vi "SetList.vi"() -> ()   [LabVIEW 2013]
uses:
  ColumnVIs/Column/Column.lvclass
  ColumnVIs/ModeCol/ModeCol.lvclass
  ColumnVIs/GroupCol/GroupCol.lvclass
  ColumnVIs/DigitalCol/DigitalCol.lvclass
  ColumnVIs/TriggerCol/TriggerCol.lvclass
  ColumnVIs/SingleValCol/SingleValCol.lvclass
  <vilib>/event_ctls.llb/eventvkey.ctl
  <vilib>/Utility/miscctls.llb/LVRowAndColumnTypeDef.ctl
  TypeDefs/RowType.ctl
  TypeDefs/TableHistory.ctl
  TypeDefs/TableArray.ctl
  DeviceVIs/Device/Device.lvclass
  TypeDefs/PreviousVersionSelect.ctl
  VariableManagerCodes/VariableManager/VariableManager.lvclass
  <vilib>/Utility/miscctls.llb/LVRowAndColumnUnsignedTypeDef.ctl
  Utils/InsertMenu/InsertFunctionMenu.lvclass
  Utils/ExternalFeedback/JSON/JSONVarSet.ctl
  PackedLibraries/LuaEvaluatorAPI.lvlibp/API/t_Caching_Expression_Evaluator_Methods_Table.ctl
  <vilib>/Utility/miscctls.llb/LVPointTypeDef.ctl
  SetListPrefs/SetListPrefs.lvclass
  <vilib>/Utility/error.llb/DialogType.ctl
  SetListPrefs/SetListPrefs.lvclass/SetListPrefs.ctl
  TypeDefs/SaveCluster.ctl
  <vilib>/Utility/miscctls.llb/LVStringsAndValuesArrayTypeDef_I32.ctl
  TypeDefs/ClickEvent.ctl
  <vilib>/Utility/miscctls.llb/LVPoint32TypeDef.ctl
  TypeDefs/SetListRefs.ctl
  Utils/LVGitInterface/GitCommitCluster/CommitCluster.ctl
  VariableManagerCodes/SequenceIndex/SequenceIndex.lvclass
  Globals/PrefsGlobal.vi
  <vilib>/Utility/cursorutil.llb/Set Cursor (Icon Pict).vi
  VariableManagerCodes/API/VariableManagerAPI.lvlib
  Globals/UserFunctions.vi
  PackedLibraries/LuaEvaluatorAPI.lvlibp
panel:
  in  "CheckSave":bool
  out "Loading Text":string="Loading..."
  in  "Launch Viewer":bool
  out "Cycle Time (s)":dbl
  in  "UpdateHWI Button":bool
  in  "StopExperiment":bool
  in  "Run Seq Button":bool
  in  "RandomSequence":bool
  in  "Run Button":bool
  in  "Cycle":bool
  out "Procedure Name":string="test_branch"
  in  "Tab Control":T1(tab)
  in  "Resume Button":bool
  in  "Program only changes":bool=TRUE
  out "SequenceHistory":string[][](table)
  in  "File Number":i32
  in  "Program during MOT loading":bool
  in  "Additional wait time (s)":dbl
  out "Igor Inform String":string
  in  "FitCol2Text Button":bool
  in  "SetList Table":string[][](table)=[["initialize", "", "Ramp", "1", "1", "0", "0", "0", "0", "0", "0", "0", "0", "0", "0", "0", "0", "0", "0", "0", "0", "0", "0", "0", "0", "0", "0", "0", "0", "100m"]]
  in  "Undo":bool
  in  "Redo":bool
  in  "Select Layout":i32(ring)=-1 items=["(On-the-fly)"=-2, "All"=-1]
  in  "ConfigLayoutsButton":bool
  in  "ManageDevicesButton":bool
  in  "User defined functions":string="-- --------------------------------------------------------------------------\n-- RbYb Beatnote Command \"frequency\" functions\n--      These functions allow us to run a sequence using absolute frequency \n--      detuning by calculating the proper command \"frequency\"\n--\n--      NOTE: Only use one TA or Re \"comm\" function, or it isn't clear which setpoint will be used\n--\n--      18.Aug.2010: Updated Master AOM offset (40 --> 42.342).\n-----------------------------------------------------------------------------\nfunction TASlowComm(Detuning,AOM)\n    return (-1*Detuning+1126.48-60.32-42.342-2*AOM)/8\n   --positive detuning is BLUE detuned, zero detuning sets TA slower beam to the 87-Rb F=2 to F'=3\nend\n\nfunction TAMOTComm(Detuning,AOM)\n    return (-1*Detuning+1126.48-60.32-42.342+AOM)/8\n   --positive detuning is BLUE detuned, zero detuning sets TA MOT beam to the 87-Rb F=2 to F'=3\nend\n\nfunction TAPComm(Detuning,AOM)\n    return (-1*Detuning+1126.48-60.32-42.342+AOM)/8\n   --positive detuning is BLUE detuned, zero detuning sets TA Probe beam to the 87-Rb F=2 to F'=3\nend\n\nfunction ReMOTComm(Detuning,AOM)\n    return (Detuning+6568.03-1126.48+60.32+42.342-2*AOM)/64\n    --positive detuning is BLUE detuned, zero detuning sets Repump MOT beam to the 87-Rb F=1 to F'=2\nend\n\nfunction ReSlowComm(Detuning,AOM)\n    return (Detuning+6568.03-1126.48+60.32+42.342+2*AOM)/64\n    --positive detuning is BLUE detuned, zero detuning sets Repump slower beam to the 87-Rb F=1 to F'=2\nend\n\n--RbLi Probe (transverse coolign launch)\nfunction PComm(Detuning)\n    return (-1*Detuning+986.16)/8\n    --positive detuning is BLUE detuned, zero detuning sets Repump slower beam to the 87-Rb F=1 to F'=2\nend\n\n-- Creates an exponential ramp from A to B in tEnd seconds\n-- useful for stopping a ramp at different times to measure T, N\nfunction ExpRampStep(t, a, b, tau, tEnd)\n   return (b - a*exp(tEnd / tau) + (a-b)*exp(t/tau))/ ( 1 - exp(tEnd / tau) );\nend\n\nfunction ExpRampEnd(tEv, a, b, tau, tEnd)\n   return (b - a*exp(tEnd / tau) + (a-b)*exp(tEv/tau))/ ( 1 - exp(tEnd / tau) );\nend\n\nfunction ExpRamp2(t,a,tau)\n   return a*exp(-t/tau)\nend\n\nfunction ExpRamp2End(tEnd,a,tau)\n   return a*exp(-tEnd/tau)\nend\n\n-- Added log chip amplifier (1 V per decade) so now we provide linear ramp to get exponential\n--     note: log() is base 'e', log10 base '10'\nfunction LineEvap(t,a,tau)\n   return 1.027*(log10(a)-t/(2.30*tau))+0.0343\nend\n\n-- final value log(V) for LineEvap\nfunction LineEvapEnd(tEnd,a,tau)\n   return 1.027*(log10(a)-tEnd/(2.30*tau))+0.0343\nend\n\n-- Convert real dipole power to log chip request V\nfunction PtoV(pow)\n   return 1.010*log10(pow/0.770)\nend\n\n-- Convert 532 horizontal (main) beam power (in mW) to V-req\nfunction PtoV532m(pow)\n   return 1.01378*log10(pow/0.54672)\nend\n\n-- Convert 532 vertical (crossing) beam power (in mW) to V-req\nfunction PtoV532c(pow)\n   return 1.03459*log10(pow/0.619665)\nend\n\n-- Convert 1064 horizontal (main) beam power (in mW) to V-req\nfunction PtoV1064m(pow)\n   return 1.0035*log10(pow/1.2104)\nend\n----------------------------------------\n-- The following functions are part of the \"standard load\" of functions and should not be messed with\n-- They are here for reference only.\n-- Please add any user functions above this comment\n-- -------------------------------------------------------------------------------------------\n\n-- Creates a linear ramp from A to B\nfunction LineRamp(f, Initial, Final)\n    return (1-f)*Initial + f*Final;\nend\n\n-- Creates an exponential ramp from A to B\nfunction ExpRamp(t, a, b, tau)\n   return (b - a*exp(tMax / tau) + (a-b)*exp(t/tau))/ ( 1 - exp(tMax / tau) );\nend\n\n-- Creates a sinewave\nfunction SinRamp(t,Offset,A,Freq, Phase)\n    return Offset + A * sin(2*pi*Freq*t + Phase)\nend\n\n-- Creates a blackman pulse\nfunction Blackman(f, Offset, A)\n    return Offset +  A*sqrt(0.5*cos(3.1415*(2*f-1))+0.08*cos(2*pi*(2*f-1))+0.42);\nend\n\n-- Creates a half-gauss ramp\nfunction HalfGaussRamp(t, a, b, Width)\n    local y;\n    y = exp(-(tMax^2)/Width^2);\n    y = (a -  b*y)/(1-y)  +  ((b-a)/(1-y))*exp(-((t-tMax)^2)/Width^2);\n    return y;\nend\n\n-- Creates an \"O'Hara\" ramp from A to B, for dipole evaporation\nfunction EvapRamp(t, a, b, tau)\n   local y;\n  y = log(a/b) / log(1+tMax/tau);\n  y = a * (1+t/tau)^(-y);\n  return y;\nend\n"
  in  "Save to File":bool
  in  "ImportToRepo":bool
  in  "Author":u16(ring) items=["SetList Program <JQIbot@users.noreply.github.com>"]
  out "Loaded Description":string
  out "LoadHash":string caption="Loaded Hash"
  in  "Load from File":bool
  in  "Description (Repo Only)":string
  in  "SaveTitle":string caption="Title/Filename"
  in  "Load keep cur. format":bool
  in  "Version Selection":T2=enum."Load DDS 4.10"
  in  "Old HWGlobals Path":path=path "C:/Experiment/Data Acquisition/Hardware Control/Hardware/2014/6Jun2014_PowerCal" caption="This file has not been loaded or saved"
  in  "Old HWGlobals History":string(combo)
  in  "Old Procedure Path":path=path "C:/Experiment/Data Acquisition/Hardware Control/procedures/Benchmarks/12Feb2014_RbQuad" caption="This file has not been loaded or saved"
  in  "Old Procedure History":string(combo)
  in  "Load Old":bool
  in  "Load Recent":string(combo)
  in  "Save to Repo":bool
  in  "Load from Repo":bool
  out "Loaded Version":string="testing"
  out "SaveHash":string caption="Saved Hash"
  in  "Error Log":i32(listbox)
  out "Table error":errorcluster
  out "Run/Sequence Error":errorcluster
  out "Update Error":errorcluster
  out "Load Long Hash/Filename":string
  out "LoadRecentFile":string
  out "TCP Quit Signal":bool
  in  "FunctionMenu":refnum<class "InsertFunctionMenu.lvclass">
  out "Index Values":T3
  out "#chg":i16
  out "Defer Pnl Upd":bool=TRUE
  out "diag. loop cnt":i32
  out "Key Focus":bool
  out "Edit Position":T4={"Row"=-2, "Column"=-2}
  out "withinSelection?":bool
  out "Val Change":bool=TRUE
  out "Selection Size":T4
  out "Selection Start":T4={"Row"=25, "Column"=30}
  out "Char":i16
  out "VKey":T5
  out "withinData?":bool=TRUE
  out "data cols":i32=134
  out "data rows":i32=26
  out "Number of Rows":u32=36
  out "Number of Columns":u32=62
  in  "Devices":refnum<class "Device.lvclass">[](array[class])
  out "Devices queue":refnum<queue>
  out "DevNums":i32[](array[numeric])=[0, 0, 0, 0, 0, 0, 0, 0, 0, 0, 0, 0, 0, 0, 0, 0, 0, 0, 0, 0, 0, 0, 0, 0, 0, 0, 0, 0, 0, 0, 1, 1, 1, 1, 1, 1, 1, 1, 1, 1, 1, 1, 1, 1, 1, 1, 1, 1, 1, 1, 2, 2, 2, 2, 2, 2, 2, 2, 2, 2, 2, 2, 2, 2, 2, 2, 2, 2, 2, 2, 3, 3, 3, 3, 3, 3, 3, 3, 3, 3, 3, 3, 3, 3, 3, 3, 3, 3, 3, 3, 4, 4, 4, 4, 4, 4, 4, 4, 5, 5, 5, 5, 5, 5, 5, 5, 5, 5, 5, 5, 6, 6, 6, 6, 6, 6, 6, 6, 6, 6, 6, 6, 7, 7, 7, 7, 7, 7, 7, 7, 7, 7, 7, 7]
  out "Col array":refnum<class "Column.lvclass">[](array[class])
  out "Seq. Event":refnum<user-event>
  out "Update Event":refnum<user-event>
  out "Update Notifier":refnum<notifier>
  out "Dyn. Regist. Update Event":refnum<event-registration>
  out "Dyn.\nRegist.\nSeq.\nEvent":refnum<event-registration>
  out "Dyn.\nRegist.\nCycleX\nEvent":refnum<event-registration>
  out "CycleX Event":refnum<user-event>
  in  "row type":T6=enum."within data"
  out "Button\n(Mouse Down?)":u16
  in  "VariableManager":refnum<class "VariableManager.lvclass">=refnum
  out "Igor Inform Array":string[](array[string])
  out "Clipboard":string[][](array[string])
  out "Table History":T7
  in  "Diag. loop?":bool
  in  "PreserveHist?":bool
  out "Hist. size":i32=2
  in  "Defer Updates?":bool=TRUE
  in  "initialize?":bool
  in  "Debug: apply appearance":bool
  out "Viewer ref":refnum<vi>
  out "LoadRecentHash":string
  out "FBVarSeqSetJSON queue":refnum<queue>
  in  "SetSharedVarIP":bool
  in  "Shared Variable Deploy IP":string
  in  "Git Authors":string[][](table)
  in  "ManGitCmd":bool
  in  "AutoGitCmd":bool
  out "Git Command":string
  in  "Procedure Repository":path
  in  "DetachVMUIonStart":bool
  in  "Auto PressHWUpdate":bool
  in  "Hide Checked Devices":i32(listbox)=3
  in  "Reset to Saved Window Position":bool
  in  "Save Current Window Position":bool
  in  "Reset at Startup":bool
  in  "quit":bool
  # "What do we actually need from old CycleX here?\n   - Inform Igor?\n   - Program changes/ during MOT load?"
  # "(not presently implemented)"
  # "To End Table Editing:\n  - Press <Ctrl>-<Return>\n  - Press <Keypad Enter>\n  - Click outside the table"
  # "Variable Manager will be initialized when the VI is run.\n\nIf it is currently running and you can see this message, then you've \"popped out\" the Variable manager.\nClose it with the \"red-x\" to replace it here."
  # "Note: For each index <idx>, the names <idx>_f and <idx>_max\nare also defined as the fractional sequence step and max steps."
  # "NOTE: these persist until LabVIEW is closed or you overwrite them."
  # "In the context of ramps several variables are passed or specified that may be used here:\n\n   - f the fractional position of a point in a ramp\n   - t the current time in a ramp\n   - dt the current timestep size.\n   - tMax the total duration of the ramp\n\ntemporary \"storage\":\n-- not functionality for strings (always treated as double)\nfunction bnot(a)\n   -- this \"(bool exp.) and b or c\" is equivalent to \"(bool exp.) ? b : c\" syntax.\n   -- caution: undefined variables evaluate to \"false\" so will NOT throw an error as argument\n   return a==0 and 1 or 0\nend"
  # "Present Version"
  # "Save/Load from present version (select single file):\nWe need to save the following:\n   - Devices (with the columns and data pushed from table first!)\n   - Layout ring (for layout names, #s)\n   - variables\n   - user functions\n   - ... ?"
  # "Load... and Save... bring up dialog box.\nLoad Recent will load the selected procedure.\nBUG: not a value change if select what's on top!"
  # "Load from older versions (select Procedure and Hardware globals)\n(1) reformat old file to give device array\n(2) collect variables and send them to variable manager\n(3) load user functions\n(4) construct layouts, if any (at least a default \"all on\" layout)\n(5) ...?"
  # "Previous Versions"
  # "Most of these controls/indicators MUST exist. At the bottom and right are some diagnostics."
  # "\"Diagnostics\" we can't delete:\nRow Type, ..."
  # "(must abort to stop,\nstill better to QUIT first)"
  # "diagnostics:"
  # "presently not set\nfor row header"
  # "The table size in (rows, cols) is NOT same as\nthe size of the data array displayed in table."
  # "SetList was developed for the JQI neutral atom cooling/trapping groups. \nPrimary contributions authored by Zack Seigel, Creston Herold, Joe Tiamsuphat, Bob Wyllie, Zach Smith.\n\nFAQs\n------\n * How are digital variables interpreted?\n     Any value not equal to 0 is high, only 0 is low.\n\n * What does Ramp mean?\n     Slave devices will be triggered (if necessary) during a Ramp line with a period given by \"Step.\" The output\n     is determined with Lua \"User Functions\" and the reserved f,t variables described on that tab.\n     Master (PulseBlaster) channels will output a *static* output during ramps. That means functions of f or t\n     will only be evaluated at their *first* point for Master channels.\n\n * How do you use Loop - EndLoop?\n     The \"Step\" column on a Loop line is for # loops and is ignored on an EndLoop line. Nesting is supported\n     up to 7 levels deep, but only Master (PulseBlaster) outputs can change. Therefore Ramps are not allowed \n     within loops.\n\n * How does Halt work?\n     On a Halt line, the Master (PulseBlaster) will change to the selected outputs and then wait for a trigger.\n     Upon receiving a trigger (hardware or software), it will wait for the specified Delay and then go to the \n     next instruction.\n\n * Where can I learn more?\n     Complete documentation of this code, including adding your own custom device can be found on the\n     JQI wiki (https://jqi-wiki.physics.umd.edu, login required)."
  # "Git Save System Settings"
  # "To setup git:\n     1) Click 'Auto-Detect Command' to find the git installation on your computer\n     2) Point 'Procedure Repository' to the path to store save files by typing or browsing.\n     (Optional) Add authors"
  # "Leave email blank to use \"JQIbot@users.noreply.github.com\""
  # "Won't show checked items in the \"Add Device...\" dropdown of the \"Manage Devices\" window"
  # "Window Position"
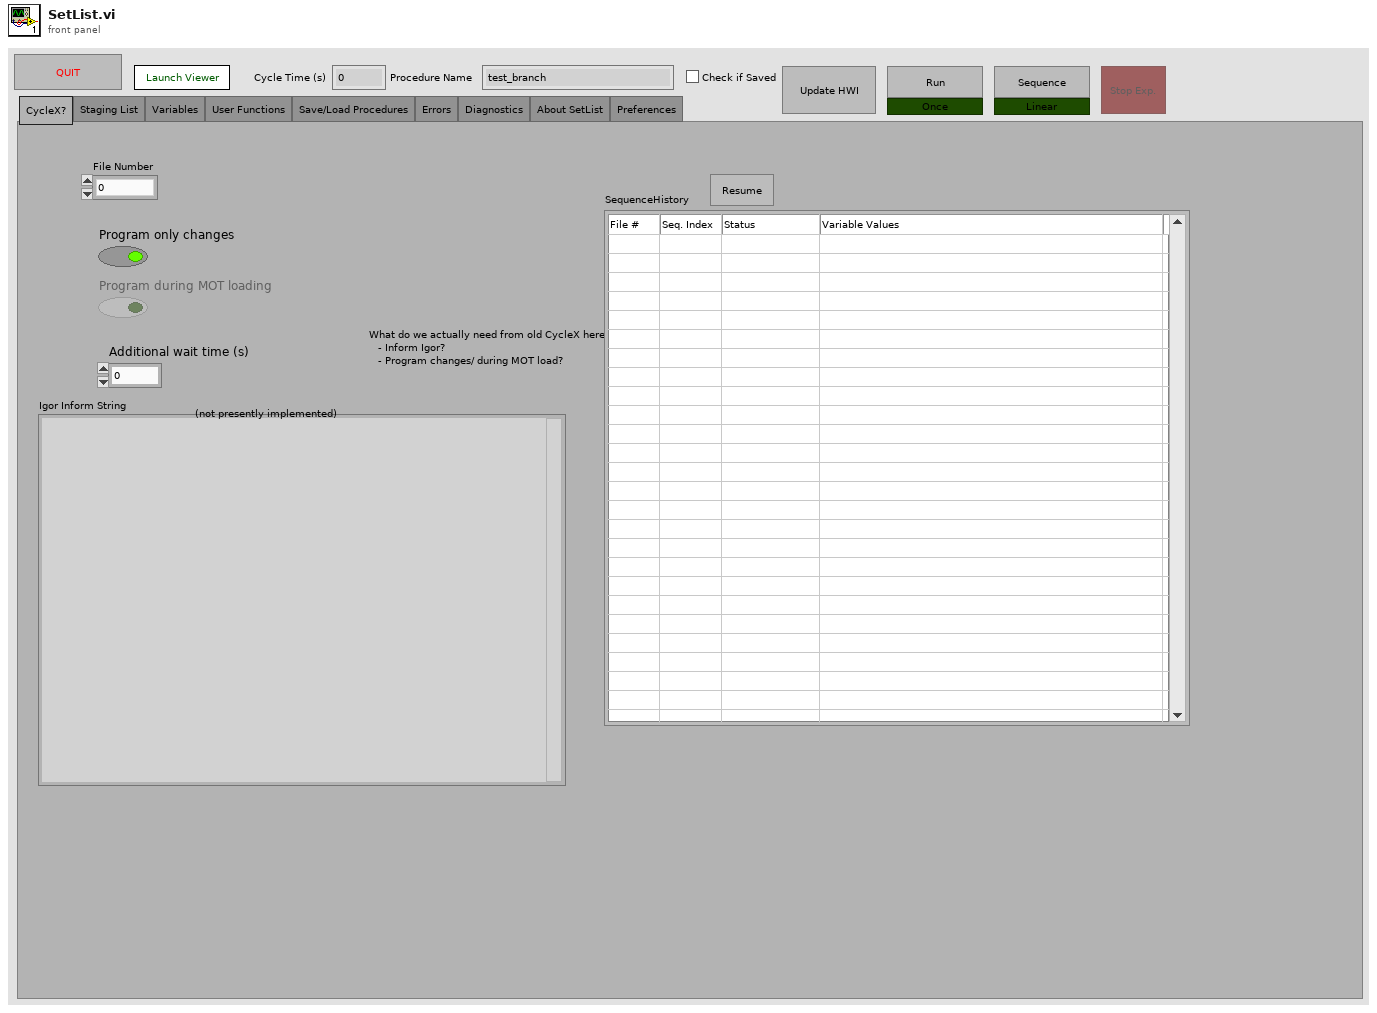
[diagram p1: front panel]
types:
  T1 = enum32{"CycleX?", "Staging List", "Variables", "User Functions", "Save/Load Procedures", "Errors", "Diagnostics", "About SetList", "Preferences"}
  T2 = typedef "PreviousVersionSelect.ctl" = enum32{"Load PreDDS 4.10", "Load early 2009 files", "Load 2009-2010 files", "Load DDS 4.10", "Load v4.09"}
  T3 = typedef "LVRowAndColumnUnsignedTypeDef.ctl" = cluster{"Row":u32, "Column":u32}
  T4 = typedef "LVRowAndColumnTypeDef.ctl" = cluster{"Row":i32, "Column":i32}
  T5 = typedef "eventvkey.ctl" = enum16{"ASCII", "Enter", "Return", "Shift", "Ctrl", "Alt", "Cmd", "Opt", "Caps", "NumLock", "Clear", "Break", "Up", "Down", "Left", "Right", "Insert", "Delete", "Home", "End", "PageUp", "PageDown", "Escape", "Help", "Pause", "ScrollLock", "F1", "F2", "F3", "F4", "F5", "F6", "F7", "F8", "F9", "F10", "F11", "F12", "F13", "F14", "F15", "F16", "F17", "F18", "F19", "F20", "F21", "F22", "F23", "F24", "Play", "VolumeUp", "VolumeDown", "Mute", "Two Byte Char"}
  T6 = typedef "RowType.ctl" = enum16{"below data", "within data", "column header", "first row"}
  T7 = typedef "TableHistory.ctl" = cluster{"Undo pointer":i32, "OldTable Array":T8}
  T8 = typedef "TableArray.ctl" = string[]
  T9 = typedef "JSONVarSet.ctl" = string[]
  T10 = typedef "LVPointTypeDef.ctl" = cluster{"Horizontal":i16, "Vertical":i16}
  T11 = typedef "LuaEvaluatorAPI.lvlibp/t_Caching_Expression_Evaluator_Methods_Table.ctl" = enum16{"set", "get", "eval", "assign", "isvalid", "execute", "evaltable", "close"}
  T12 = enum8{"Enabled", "Disabled", "Disabled and Grayed Out"}
  T13 = typedef "LVRectTypeDef.ctl" = cluster{"Left":i16, "Top":i16, "Right":i16, "Bottom":i16}
  T14 = cluster{"WindowBounds":T13, "ResetPositionAtStartup":bool}
  T15 = cluster{"Device Class Name":string, "Class Path":path}[]
  T16 = typedef "ClickEvent.ctl" = cluster{"CtlRef":refnum<vi>, "Coords":T17, "Button":u16, "Mods":cluster{"Double Click":bool, "Menu Key":bool}, "PlatMods":cluster{"Shift":bool, "Ctrl":bool, "Alt":bool, "Cmd":bool, "Opt":bool}}
  T17 = typedef "LVPoint32TypeDef.ctl" = cluster{"Horizontal":i32, "Vertical":i32}
  T18 = typedef "SetListRefs.ctl" = cluster{"Clipboard":refnum<vi>, "Layout Ring Refnum":refnum<vi>, "Col Array Ref in":refnum<vi>, "VariableManagerRef":refnum<vi>, "Table CtlRef In":refnum<vi>, "Table History ref":refnum<vi>, "Devices queue":refnum<queue>, "FunctionMenu Ref":refnum<vi>}
  T19 = typedef "SaveCluster.ctl" = cluster{"Version":string, "Devices":refnum<class "Device.lvclass">[], "Select Layout":i32, "Layout:Strings And Values []":T20, "User defined functions":string, "VariableManager":refnum<class "VariableManager.lvclass">}
  T20 = typedef "LVStringsAndValuesArrayTypeDef_I32.ctl" = cluster{"String":string, "Value":i32}[]
  T21 = cluster{"Title":string, "Description":string, "Author":string}
  T22 = typedef "CommitCluster.ctl" = cluster{"Hash":string, "Date":string, "Name":string}
  T23 = enum32{"CycleX?", "Staging List", "Variables", "User Functions", "Save/Load Procedures", "Errors", "Diagnostics", "About SetList"}
  T24 = cluster{"Shift":bool, "Ctrl":bool, "Alt":bool, "Cmd":bool, "Opt":bool}
  T25 = typedef "ClickReturn.ctl" = cluster{"Button":u16, "Mods":cluster{"Double Click":bool, "Menu Key":bool}, "PlatMods":cluster{"Shift":bool, "Ctrl":bool, "Alt":bool, "Cmd":bool, "Opt":bool}, "Discard?":bool}
  T26 = typedef "DialogType.ctl" = u16
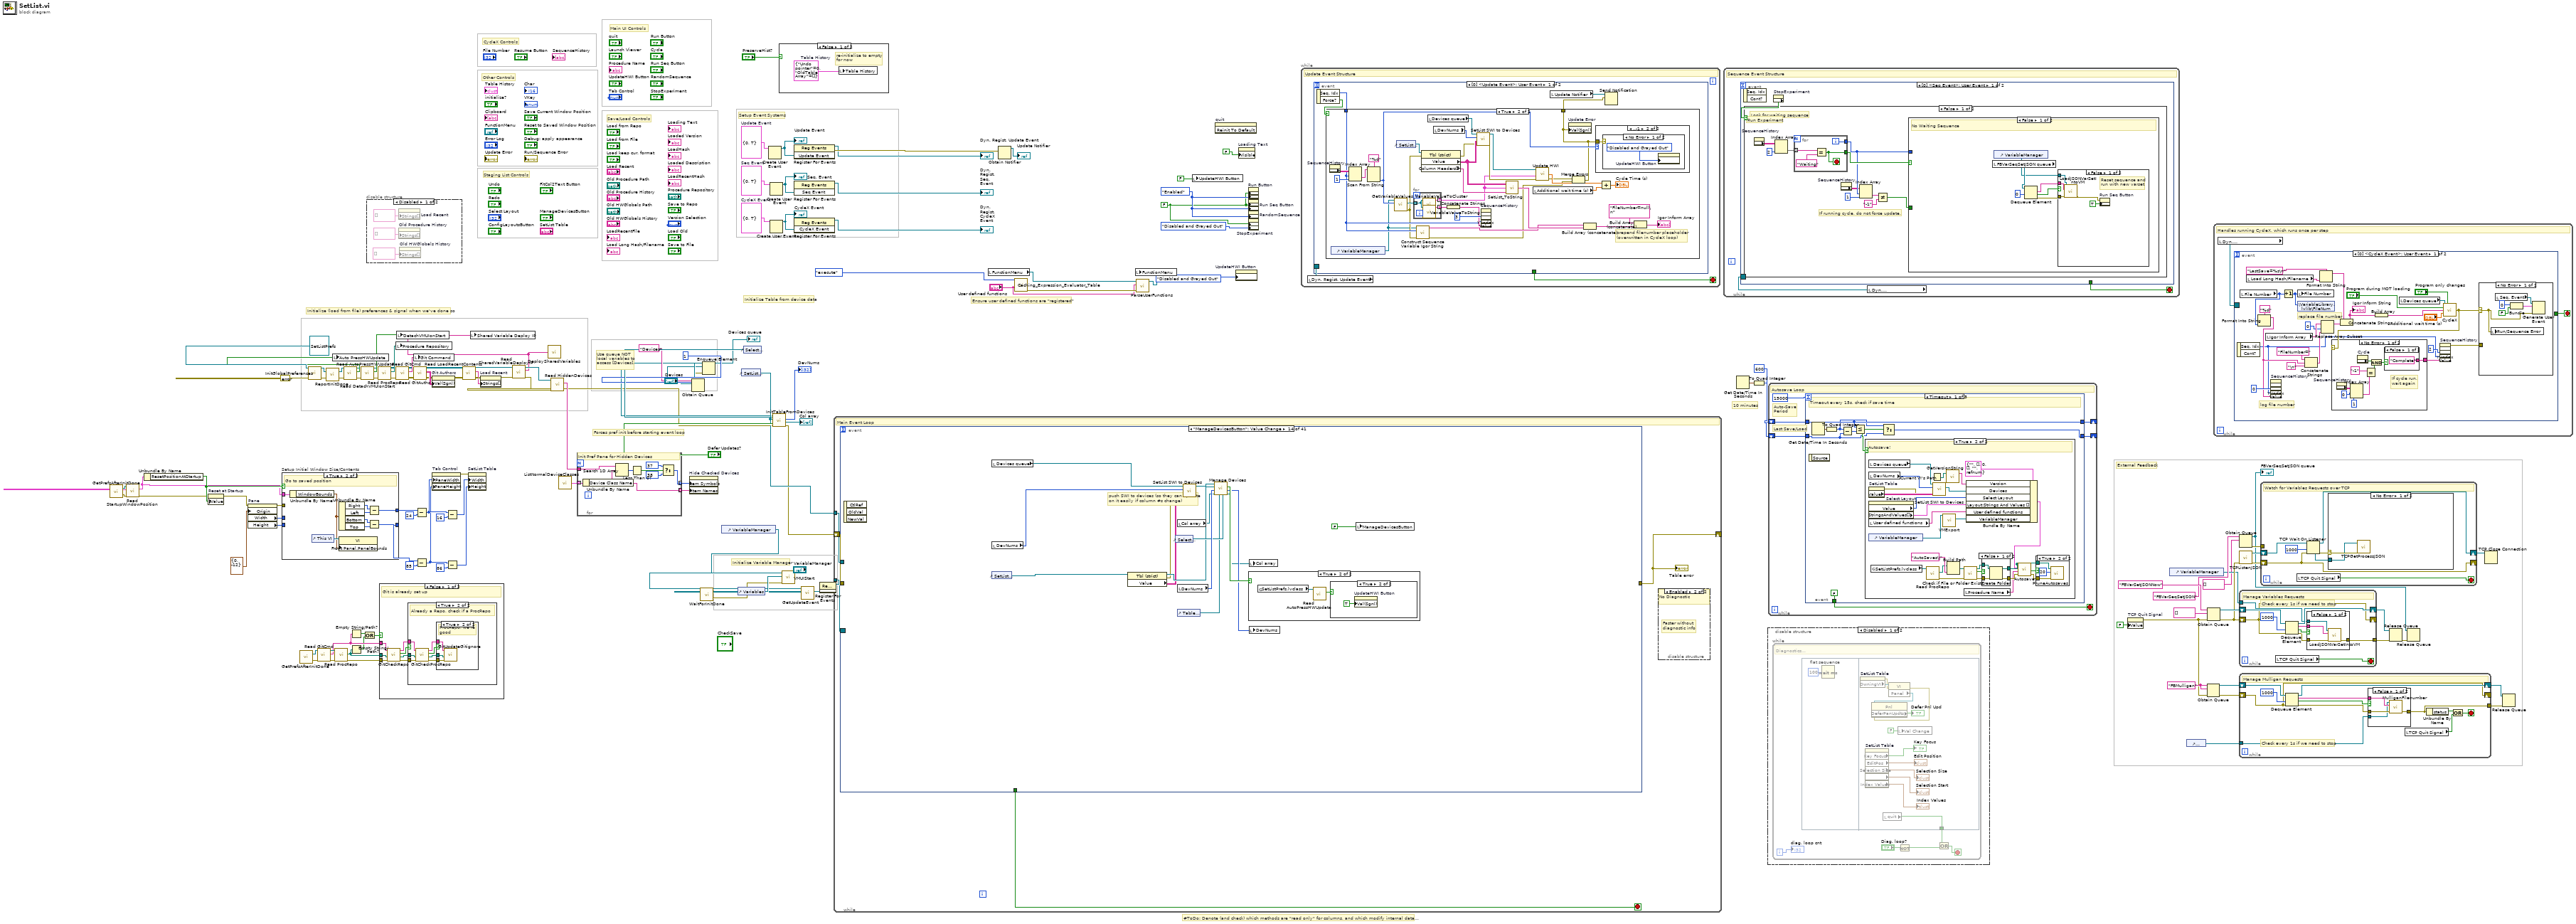
[diagram p0: block diagram]
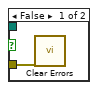
[diagram p8: hidden frame]
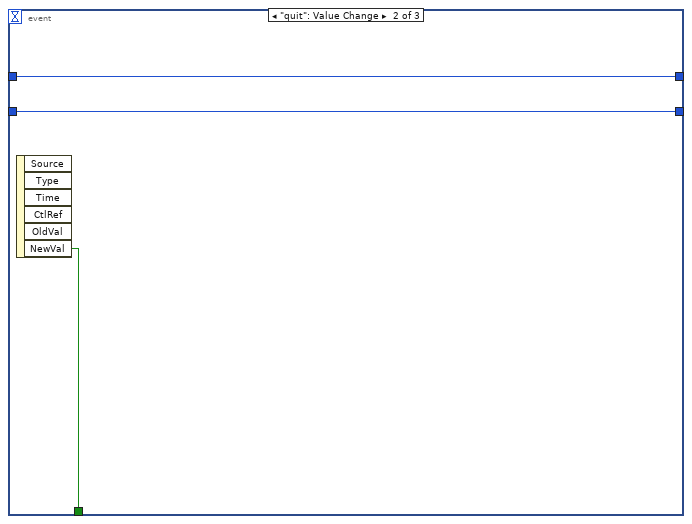
[diagram p9: hidden frame]
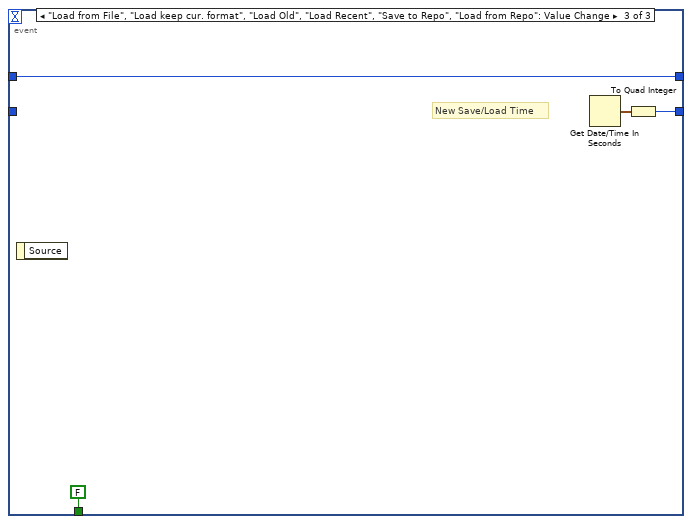
[diagram p10: hidden frame]
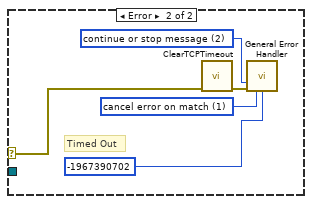
[diagram p11: hidden frame]
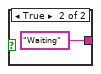
[diagram p15: hidden frame]
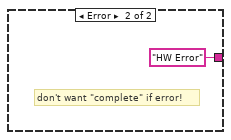
[diagram p16: hidden frame]
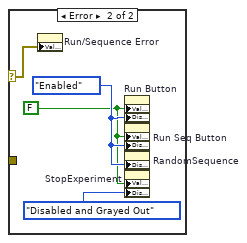
[diagram p17: hidden frame]
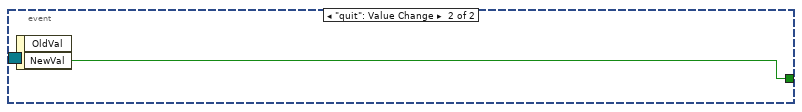
[diagram p18: hidden frame]
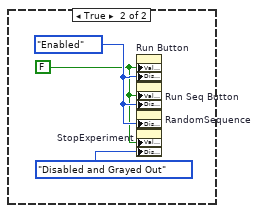
[diagram p20: hidden frame]
diagram:
  w56 = "FBMulligan" ("name (unnamed)")
  w110 = T12."Enabled" ("Disabled")
  w109 = FALSE
  w120 = cluster{"Seq. Idx":i32, "Cont?":bool} {"Seq. Idx"=0, "Cont?"=TRUE}  # CycleX Event
  w129 = cluster{"Seq. Idx":i32, "Cont?":bool} {"Seq. Idx"=0, "Cont?"=TRUE}  # Seq Event
  w130 = cluster{"Seq. Idx":i32, "Force?":bool} {"Seq. Idx"=0, "Force?"=TRUE}  # Update Event
  # "External Feedback"
  # "10 minutes"
  # "Forces pref init before starting event loop"
  # "Initialize (load from file) preferences & signal when we've done so"
  # "CycleX Controls"
  # "Main UI Controls"
  # "Other Controls"
  # "Save/Load Controls"
  # "Staging List Controls"
  # "Setup Event Systems"
  # "Use queue NOT\nlocal variables to\naccess [Devices]."
  # "Ensure user defined functions are \"registered\""
  # "Initialize Variable Manager"
  # "Initialize Table from device data"
  # "#ToDo: Denote (and check) which methods are \"read only\" for columns, and which modify internal data..."
  n1 = call "GetPrefsAfterInitDone.vi"() -> ("error out"=w82:errorcluster, "Preferences out"=w81:refnum<class "SetListPrefs.lvclass">)  [unwired: 2 in]
  n2 = call "Read StartupWindowPosition.vi"("error in (no error)"=w82, "SetListPrefs in"=w81) -> ("error out"=w79:errorcluster, "StartupWindowPosition"=w78:T14)  [unwired: 7 in, 1 out]
  n3 = Unbundle By Name(w78) -> ("ResetPositionAtStartup"=w80:bool)
  n4 = property on="Reset at Startup" class="Bool (strict)"(error in=w79, "Value"=w80) -> (error out=w77:errorcluster)  [unwired: 1 in, 1 out]
  n5 = property on="Pane" class="Pane"(error in=w77, "Origin"=T10 {"Horizontal"=0, "Vertical"=-12}) -> (error out=w76:errorcluster, "Width"=w75:u32, "Height"=w74:u32)  [unwired: 1 in, 1 out]
  n6 = case "Setup Initial Window Size/Contents" shown="True" w80 {
    tunnel: w78 -> [_ w142]
    tunnel: w76 -> [_ _]
    tunnel: w75 -> [w133 _]
    tunnel: w74 -> [w134 _]
    tunnel: [w133 w136] -> w73
    tunnel: [w134 w135] -> w72
    frame False {
      # "Keep current, but still resize contents"
    }
    frame True {
      # "Go to saved position"
      n7 = Unbundle By Name(w142) -> ("WindowBounds"=w137:T13)
      n8 = control-ref of="This VI"() -> (w143:refnum<vi>)
      n9 = Unbundle By Name(w137) -> ("Right"=w141:i16, "Left"=w140:i16, "Bottom"=w139:i16, "Top"=w138:i16)
      n10 = property class="VI"(reference=w143, "Front Panel.PanelBounds"=w137) -> ()  [unwired: 1 in, 2 out]
      n11 = Subtract(x=w141, y=w140) -> (x-y=w136:i16)
      n12 = Subtract(x=w139, y=w138) -> (x-y=w135:i16)
    }
  }
  n13 = call "GetPrefsAfterInitDone.vi"() -> ("error out"=w20:errorcluster, "Preferences out"=w19:refnum<class "SetListPrefs.lvclass">)  [unwired: 2 in]
  n14 = call-dynamic "InitGlobalPreferences.vi"("error in (no error)"=errorcluster {"status"=FALSE, "code"=0, "source"=""} ("error out"), "Preferences in"=refnum<class "SetListPrefs.lvclass"> refnum ("SetListPrefs.lvclass")) -> ("error out"=w84:errorcluster, "Preferences out"=w83:refnum<class "SetListPrefs.lvclass">)  [unwired: 7 in, 1 out]
  n15 = call "Read GitCmd.vi"("error in (no error)"=w20, "SetListPrefs in"=w19) -> ("error out"=w18:errorcluster, "GitCmd"=w15:string, "SetListPrefs out"=w16:refnum<class "SetListPrefs.lvclass">)  [unwired: 7 in]
  n16 = call "ReportInitDone.vi"("error in (no error)"=w84, "Preferences in"=w83) -> ("error out"=w67:errorcluster, "Preferences out"=w68:refnum<class "SetListPrefs.lvclass">)
  n17 = call "Read ProcRepo.vi"("error in (no error)"=w18, "SetListPrefs in"=w16) -> ("error out"=w17:errorcluster, "ProcRepo"=w14:path)  [unwired: 7 in, 1 out]
  n18 = call "Read AutoPressHWUpdate.vi"("error in (no error)"=w67, "SetListPrefs in"=w68) -> ("error out"=w64:errorcluster, "AutoPressHWUpdate"=w66:bool, "SetListPrefs out"=w63:refnum<class "SetListPrefs.lvclass">)  [unwired: 7 in]
  n19 = local write "Auto PressHWUpdate"(w66) -> ()
  n20 = Empty String/Path?(string/path=w15) -> (empty?=w13:bool)
  n21 = Empty String/Path?(string/path=w14) -> (empty?=w12:bool)
  n22 = call "Read DetachVMUIonStart.vi"("error in (no error)"=w64, "SetListPrefs in"=w63) -> ("error out"=w42:errorcluster, "DetachVMUIonStart"=w62:bool, "SetListPrefs out"=w40:refnum<class "SetListPrefs.lvclass">)  [unwired: 7 in]
  n23 = Or(x=w13, y=w12) -> (x .or. y?=w11:bool)
  n24 = disable-structure shown="Disabled" {
    frame Disabled {
      n25 = property on="Load Recent" class="CmbBox"("Strings[]"=string[] [] ("Strings []")) -> ()  [unwired: 2 in, 2 out]
      n26 = property on="Old Procedure History" class="CmbBox"("Strings[]"=string[] [] ("Strings []")) -> ()  [unwired: 2 in, 2 out]
      n27 = property on="Old HWGlobals History" class="CmbBox"("Strings[]"=string[] [] ("Strings []")) -> ()  [unwired: 2 in, 2 out]
    }
    frame Enabled {
    }
  }
  n28 = call "Read ProcRepo.vi"("error in (no error)"=w42, "SetListPrefs in"=w40) -> ("error out"=w39:errorcluster, "ProcRepo"=w41:path, "SetListPrefs out"=w38:refnum<class "SetListPrefs.lvclass">)  [unwired: 7 in]
  n29 = case shown="False" w11 {
    tunnel: w15 -> [w153 _]
    tunnel: w17 -> [w148 _]
    tunnel: w14 -> [w147 _]
    frame False {
      # "Git is already set up"
      n30 = call "GitCheckRepo.vi"("error in (no error)"=w148, "Directory"=w147, "Git exec"=w153) -> ("error out"=w150:errorcluster, "Directory out"=w151:path, "ProcedureRepo?"=w149:bool, "Git exec out"=w152:string)  [unwired: 5 in]
      n31 = case shown="True" w149 {
        tunnel: w150 -> [_ w160]
        tunnel: w151 -> [_ w159]
        tunnel: w152 -> [_ w158]
        frame False {
          # "Do Nothing"
        }
        frame True {
          # "Already a Repo, check if a ProcRepo"
          n32 = call "GitCheckProcRepo.vi"("error in (no error)"=w160, "Directory"=w159, "Git exec"=w158) -> ("error out"=w156:errorcluster, "Directory out"=w155:path, "ProcedureRepo?"=w154:bool, "Git exec out"=w157:string)  [unwired: 5 in]
          n33 = case shown="True" w154 {
            tunnel: w157 -> [_ w161]
            tunnel: w156 -> [_ w163]
            tunnel: w155 -> [_ w162]
            frame False {
              # "Do Nothing"
            }
            frame True {
              # "ProcRepo, we're good"
              n34 = call "GitUpdateGitignore.vi"("error in (no error)"=w163, "Directory in"=w162, "Git exec in"=w161) -> ()  [unwired: 6 in, 3 out]
            }
          }
        }
      }
    }
    frame True {
      # "Git isn't fully set up yet."
    }
  }
  n35 = local write "Procedure Repository"(w41) -> ()
  n36 = call "Read GitCmd.vi"("error in (no error)"=w39, "SetListPrefs in"=w38) -> ("error out"=w36:errorcluster, "GitCmd"=w37:string, "SetListPrefs out"=w35:refnum<class "SetListPrefs.lvclass">)  [unwired: 7 in]
  n37 = local write "DetachVMUIonStart"(w62) -> ()
  n38 = local write "Git Command"(w37) -> ()
  n39 = call "Read GitAuths.vi"("error in (no error)"=w36, "SetListPrefs in"=w35) -> ("error out"=w33:errorcluster, "GitAuths"=w34:string[][], "SetListPrefs out"=w32:refnum<class "SetListPrefs.lvclass">)  [unwired: 7 in]
  n40 = Subtract(x=w73, y=u32 24) -> (x-y=w89:u32)
  n41 = Subtract(x=w72, y=u32 85) -> (x-y=w88:u32)
  n42 = property on="Git Authors" class="Tbl (strict)"(error in=w33, "Val(Sgnl)"=w34) -> (error out=w31:errorcluster)  [unwired: 1 in, 1 out]
  n43 = property on="Tab Control" class="TabCtl (strict)"("PaneWidth"=w89, "PaneHeight"=w88) -> (error out=w90:errorcluster)  [unwired: 2 in, 1 out]
  n44 = Subtract(x=w89, y=u32 16) -> (x-y=w92:u32)
  n45 = Subtract(x=w88, y=u32 86) -> (x-y=w91:u32)
  n46 = call "Read LoadRecentContents.vi"("error in (no error)"=w31, "SetListPrefs in"=w32) -> ("error out"=w30:errorcluster, "LoadRecentContents"=w29:string[], "SetListPrefs out"=w6:refnum<class "SetListPrefs.lvclass">)  [unwired: 7 in]
  n47 = property on="SetList Table" class="Tbl (strict)"(error in=w90, "Width"=w92, "Height"=w91) -> ()  [unwired: 1 in, 2 out]
  n48 = property on="Load Recent" class="CmbBox"(error in=w30, "Strings[]"=w29) -> (error out=w8:errorcluster)  [unwired: 1 in, 1 out]
  n49 = call "Read SharedVariableDeployIP.vi"("error in (no error)"=w8, "SetListPrefs in"=w6) -> ("error out"=w7:errorcluster, "SharedVariableDeployIP"=w4:string, "SetListPrefs out"=w5:refnum<class "SetListPrefs.lvclass">)  [unwired: 7 in]
  n50 = local write "Shared Variable Deploy IP"(w4) -> ()
  n51 = call "DeploySharedVariables.vi"("Target IPAddress"=w4) -> ()  [unwired: 1 out]
  n52 = call "Read HiddenDevices.vi"("error in (no error)"=w7, "SetListPrefs in"=w5) -> ("error out"=w10:errorcluster, "HiddenDevices"=w69:string[])  [unwired: 7 in, 1 out]
  n53 = call "ListNormalDeviceClasses.vi"() -> ("Detected Device Classes"=w9:T15)  [unwired: 1 in]
  n54 = for {
    tunnel: [w164] -> w71 mode=indexing
    tunnel: [w169] -> w70 mode=indexing
    tunnel: w69 -> [w168]
    tunnel: w9 -> [w165] mode=indexing
    # "Init Pref Pane for Hidden Devices"
    n55 = Unbundle By Name(w165) -> ("Device Class Name"=w164:string)
    n56 = Search 1D Array(1D array=w168, element=w164) -> (index of element=w167:i32)  [unwired: 1 in]
    n57 = Less Than 0?(x=w167) -> (x < 0?=w166:bool)
    n58 = Select(t=37, s=w166, f=38) -> (s? t:f=w169:i32)
  }
  n59 = property on="Hide Checked Devices" class="LstBox (strict)"("Item Symbols"=w70, "Item Names"=w71) -> ()  [unwired: 2 in, 2 out]
  n60 = Obtain Queue(max queue size (-1, unlimited)=1, name (unnamed)="Devices", element data type="Devices") -> (queue out=w103:refnum<queue>, error out=w102:errorcluster)  [unwired: 2 in, 1 out]
  n61 = call "WaitForInitDone.vi"() -> ("error out"=w65:errorcluster)  [unwired: 2 in, 1 out]
  n62 = Enqueue Element(queue=w103, element="Devices", error in (no error)=w102) -> (queue out=w101:refnum<queue>)  [unwired: 1 in, 2 out]
  "Devices queue" <- w101
  n63 = control-ref of="VariableManager"() -> (w23:refnum<vi>)
  n64 = control-ref of="Variables"() -> (w112:refnum<vi>)
  n65 = control-ref of="SetList Table"() -> (w114:refnum<vi>)
  n66 = control-ref of="Select Layout"() -> (w125:refnum<vi>)
  n67 = Create User Event(user event datatype=w130) -> (user event=w131:refnum<user-event>)  [unwired: 1 in, 1 out]
  "Update Event" <- w131
  n68 = Create User Event(user event datatype=w129) -> (user event=w117:refnum<user-event>)  [unwired: 1 in, 1 out]
  "Seq. Event" <- w117
  n69 = Create User Event(user event datatype=w120) -> (user event=w119:refnum<user-event>)  [unwired: 1 in, 1 out]
  "CycleX Event" <- w119
  n70 = call "InitTableFromDevices.vi"("Defer Updates? (T)"="Defer Updates?", "Layout Ref"=w125, "error in (no error)"=w10, "Table Ref in"=w114, "Devices queue"=w101) -> ("error out"=w113:errorcluster, "Col array"=→"Col array":refnum<class "Column.lvclass">[], "DevNums"=→"DevNums":i32[])  [unwired: 3 in, 1 out]
  n71 = case shown="False" "PreserveHist?" {
    frame False {
      w172 = T7 {"Undo pointer"=0, "OldTable Array"=[]}  # Table History
      # "re-initialize to empty\nfor now"
      n72 = local write "Table History"(w172) -> ()
    }
    frame True {
    }
  }
  n73 = call "VMUIStart.vi"("error in (no error)"=w65, "SubPanelRef"=w112, "VariableManagerRef in"=w23) -> ("VariableManagerRef out"=w108:refnum<vi>)  [unwired: 7 in, 1 out]
  n74 = register-events(w131) -> (reference out=→"Dyn. Regist. Update Event":refnum<event-registration>, error out=w127:errorcluster)  [unwired: 2 in]
  n75 = register-events(w117) -> (reference out=→"Dyn.\nRegist.\nSeq.\nEvent":refnum<event-registration>)  [unwired: 2 in, 1 out]
  n76 = register-events(w119) -> (reference out=→"Dyn.\nRegist.\nCycleX\nEvent":refnum<event-registration>)  [unwired: 2 in, 1 out]
  n77 = call "GetUpdateEvent.vi"("VariableManagerRef in"=w108) -> ("UpdateEvent"=w107:refnum<user-event>)  [unwired: 8 in, 2 out]
  n78 = register-events(w107) -> (reference out=w106:refnum<event-registration>)  [unwired: 2 in, 1 out]
  n79 = while {
    shift-right: [w175] -> _
    shift-left: w113 -> [w176]
    tunnel: w114 -> [w174]
    tunnel: w106 -> [w173]
    stop <- w177 stop-if-true
    # "Main Event Loop"
    n80 = event shown="[13] \"ManageDevicesButton\": Value Change" {
      selector: w173 -> [_ _ _ _ _ _ _ _ _ _ _ _ _ _ _ _ _ _ _ _ _ _ _ _ _ _ _ _ _ _ _ _ _ _ _ _ _ _ _ _ _]
      dyn-events: _ -> [_ _ _ _ _ _ _ _ _ _ _ _ _ _ _ _ _ _ _ _ _ _ _ _ _ _ _ _ _ _ _ _ _ _ _ _ _ _ _ _ _]
      timeout: _ -> [_ _ _ _ _ _ _ _ _ _ _ _ _ _ _ _ _ _ _ _ _ _ _ _ _ _ _ _ _ _ _ _ _ _ _ _ _ _ _ _ _]
      tunnel: [_ _ _ _ _ _ _ _ _ _ _ _ _ _ w471 _ _ _ _ _ _ _ _ _ _ _ _ _ _ _ _ _ _ _ _ _ _ _ _ _ _] -> w177
      tunnel: [w183 w191 w257 _ w276 w330 w341 w344 w353 _ w393 w398 w421 _ w461 w483 w512 _ _ _ _ _ _ _ _ w793 _ _ w813 _ _ _ _ _ _ _ _ _ _ _ _] -> w175
      tunnel: w176 -> [w186 w195 w245 w270 w302 w336 w342 w345 w350 _ w394 w400 w425 _ w466 w482 w514 _ _ _ _ _ _ _ _ w789 _ _ _ _ _ _ _ _ _ _ _ _ _ _ _]
      tunnel: w174 -> [_ _ _ _ _ _ _ _ _ _ w392 _ w424 _ _ w480 w509 _ _ _ _ _ _ _ _ _ _ _ _ _ _ _ _ _ _ _ _ _ _ _ _]
      event "initialize?": Value Change {
        # "using invoke node slows down button reset,\ndisplaying \"initializing...\" to user"
        # "This VI is also be called on Load and when the program is first run."
        n81 = event-data() -> ()  [unwired: 1 in, 1 out]
        n82 = local read "Devices queue"() -> (w181:refnum<queue>)
        n83 = control-ref of="Select Layout"() -> (w187:refnum<vi>)
        n84 = control-ref of="SetList Table"() -> (w188:refnum<vi>)
        n85 = local read "Defer Updates?"() -> (w185:bool)
        n86 = call "InitTableFromDevices.vi"("Defer Updates? (T)"=w185, "Layout Ref"=w187, "error in (no error)"=w186, "Table Ref in"=w188, "Devices queue"=w181) -> ("error out"=w184:errorcluster, "Col array"=w182:refnum<class "Column.lvclass">[], "DevNums"=w189:i32[])  [unwired: 3 in, 1 out]
        n87 = local write "Col array"(w182) -> ()
        n88 = local write "DevNums"(w189) -> ()
        n89 = invoke on="initialize?" class="Bool (strict)" method="Reinit To Default"(error in=w184) -> (error out=w183:errorcluster)  [unwired: 2 in, 2 out]
      }
      event "SetList Table": Value Change {
        # "presently assumes value change to single cell!"
        # "need to catch digital value change ->appear change"
        # "Value change (e.g. tab and enter) shouldn't change array size.\nOnly way to add/remove rows is through mouse clicks..."
        # "monitor sizes"
        n90 = event-data() -> ("CtlRef"=w194:refnum<vi>, "OldVal"=w196:string[][], "NewVal"=w193:string[][])  [unwired: 1 in]
        n91 = Array Size(array=w196) -> (size(s)=w204:i32[])
        n92 = Array Size(array=w193) -> (size(s)=w207:i32[])
        n93 = property on="Property Node" class="Tbl (strict)"(reference=w194, error in=w195) -> (error out=w192:errorcluster, "Number of Rows"=→"Number of Rows":u32, "Number of Columns"=→"Number of Columns":u32)  [unwired: 1 out]
        n94 = Index Array(array=w207) -> (element #1=w203:i32, element #2=w202:i32)  [unwired: 2 in]
        n95 = Index Array(array=w204) -> (element #1=w199:i32, element #2=w198:i32)  [unwired: 2 in]
        "data rows" <- w199
        "data cols" <- w198
        n96 = Equal?(x=w203, y=w199) -> (x = y?=w200:bool)
        n97 = Equal?(x=w202, y=w198) -> (x = y?=w201:bool)
        n98 = And(x=w200, y=w201) -> (x .and. y?=w197:bool)
        n99 = case shown="True" w197 {
          tunnel: w196 -> [w209 w216]
          tunnel: w193 -> [_ w220]
          tunnel: w192 -> [w208 w217]
          tunnel: [w208 w221] -> w191
          frame False {
            # "non-allowed resize:\nrevert back to previous table"
            # "Changed outside existing data; discard"
            n100 = local write "SetList Table"(w209) -> ()
          }
          frame True {
            # "Change within existing data"
            n101 = Not Equal?(x=w216, y=w220) -> (x != y?=w214:bool[][])
            n102 = control-ref of="Table History"() -> (w215:refnum<vi>)
            n103 = Boolean To (0,1)(Boolean=w214) -> (0, 1=w213:i16[][])
            n104 = Add Array Elements(numeric array=w213) -> (sum=→"#chg":i16)
            n105 = Or Array Elements(Boolean array=w214) -> (logical OR=w219:bool)
            n106 = call "SaveToTblHist.vi"("error in (no error)"=w217, "OldTable (reset)"=w216, "Table History ref"=w215) -> ("error out"=w218:errorcluster)  [unwired: 8 in]
            n107 = case shown="True" w219 {
              tunnel: w214 -> [_ w238]
              tunnel: w218 -> [w224 w227]
              tunnel: [w224 w235] -> w221
              tunnel: w220 -> [_ w231]
              frame False {
                # "No value change! (debugging event)"
              }
              frame True {
                # "new val"
                # "Find col, row of value change; notify column"
                n108 = for {
                  tunnel: w238 -> [w242] mode=indexing
                  tunnel: [w242] -> w237
                  tunnel: [w241] -> w230
                  i -> [w241]
                  stop <- w243 stop-if-true
                  # "which row?"
                  n109 = Or Array Elements(Boolean array=w242) -> (logical OR=w243:bool)
                }
                n110 = for {
                  tunnel: w237 -> [w239] mode=indexing
                  tunnel: [w240] -> w229
                  i -> [w240]
                  stop <- w239 stop-if-true
                  # "which col?"
                }
                n111 = Bundle By Name(cluster=T4 {"Row"=0, "Column"=0} ("Cell Position"), "Row"=w230, "Column"=w229) -> (w233:T4)
                n112 = Index Array(array=w231, index (row)=w230, index (col)=w229) -> (element=w228:string)
                n113 = local read "Col array"() -> (w226:refnum<class "Column.lvclass">[])
                n114 = Index Array(array=w226, index=w229) -> (element=w232:refnum<class "Column.lvclass">)
                n115 = control-ref of="SetList Table"() -> (w234:refnum<vi>)
                n116 = control-ref of="Col array"() -> (w225:refnum<vi>)
                n117 = call-dynamic "ValChange.vi"("Value"=w228, "Col Array Ref in"=w225, "error in (no error)"=w227, "Table CtlRef In"=w234, "Cell Position"=w233, "Column in"=w232) -> ("error out"=w235:errorcluster)  [unwired: 3 in, 2 out]
              }
            }
            n118 = global read "PrefsGlobal.vi" "SetListPrefs.lvclass"() -> (w211:refnum<class "SetListPrefs.lvclass">)
            n119 = call "Read AutoPressHWUpdate.vi"("SetListPrefs in"=w211) -> ("AutoPressHWUpdate"=w210:bool)  [unwired: 8 in, 2 out]
            n120 = case shown="False" w210 {
              frame False {
                n121 = property on="UpdateHWI Button" class="Bool (strict)"("DisabledEnum"=T12."Enabled" ("Disabled")) -> ()  [unwired: 2 in, 2 out]
              }
              frame True {
                n122 = property on="UpdateHWI Button" class="Bool (strict)"("Val(Sgnl)"=TRUE ("Value (Signaling)")) -> ()  [unwired: 2 in, 2 out]
              }
            }
          }
        }
        "Val Change" <- TRUE ("Val Change")
      }
      event "SetList Table": Mouse Down? {
        # "Note: need to check comments in shortcut menu events and update \"mouse down?\" references to new event."
        # "Filter Mouse Down click so that (1) columns can choose to change button (like mode column) and (2) so that some clicks can (sparingly!) be discarded.\nEach column will provide a MouseDown method.\n\nSortClicks (which ultimately called LeftClick) will be moved to Mouse Up event. (is this possible? if shortcut menu is activated, Mouse Up is skipped!)"
        # "No need for DeferPanUpdts here... In fact it screws up click-and-drag!"
        n123 = event-data() -> ("CtlRef"=w262:refnum<vi>, "Coords"=w261:T17, "Button"=w260:u16, "Mods"=w259:cluster{"Double Click":bool, "Menu Key":bool}, "PlatMods"=w258:T24)  [unwired: 1 in]
        "Button\n(Mouse Down?)" <- w260
        n124 = local read "Col array"() -> (w244:refnum<class "Column.lvclass">[])
        n125 = control-ref of="Table History"() -> (w252:refnum<vi>)
        n126 = Bundle By Name(cluster=T16 {"CtlRef"=refnum, "Coords"={"Horizontal"=0, "Vertical"=0}, "Button"=0, "Mods"={"Double Click"=FALSE, "Menu Key"=FALSE}, "PlatMods"={"Shift"=FALSE, "Ctrl"=FALSE, "Alt"=FALSE, "Cmd"=FALSE, "Opt"=FALSE}} ("ClickEvent"), "CtlRef"=w262, "Coords"=w261, "Button"=w260, "Mods"=w259, "PlatMods"=w258) -> (w251:T16)
        n127 = call "SortClicks.vi"("Table History ref"=w252, "error in (no error)"=w245, "ClickEvent in"=w251, "Col array in"=w244) -> ("error out"=w257:errorcluster, "Row Type"=w254:T6, "Click out"=w250:T25, "Col array out"=w255:refnum<class "Column.lvclass">[], "Update HWI?"=w253:bool, "withinData?"=→"withinData?":bool)  [unwired: 2 in]
        n128 = case shown="True" w253 {
          frame False {
          }
          frame True {
            n129 = global read "PrefsGlobal.vi" "SetListPrefs.lvclass"() -> (w266:refnum<class "SetListPrefs.lvclass">)
            n130 = call "Read AutoPressHWUpdate.vi"("SetListPrefs in"=w266) -> ("AutoPressHWUpdate"=w265:bool)  [unwired: 8 in, 2 out]
            n131 = case shown="True" w265 {
              frame False {
                n132 = property on="UpdateHWI Button" class="Bool (strict)"("DisabledEnum"=T12."Enabled" ("Disabled")) -> ()  [unwired: 2 in, 2 out]
              }
              frame True {
                n133 = property on="UpdateHWI Button" class="Bool (strict)"("Val(Sgnl)"=TRUE ("Value (Signaling)")) -> ()  [unwired: 2 in, 2 out]
              }
            }
          }
        }
        n134 = local write "row type"(w254) -> ()
        n135 = disable-structure shown="Disabled" {
          disable-tunnel: w255 -> [w264 _]
          frame Disabled {
            n136 = local write "Col array"(w264) -> ()
          }
          frame Enabled {
          }
        }
        n137 = Unbundle By Name(w250) -> ("Button"=w248:u16, "Mods"=w247:cluster{"Double Click":bool, "Menu Key":bool}, "PlatMods"=w246:T24, "Discard?"=w249:bool)
        n138 = event-data("Button"=w248, "Mods"=w247, "PlatMods"=w246, "Discard?"=w249) -> ()  [unwired: 1 in, 1 out]
      }
      event "SetList Table": Mouse Up {
        # "Mouse Up is now where the action happens. If up occurs over the same cell as down, it is a \"click\" and left click is called after sorting buttions.\nHowever if up occurs over a different cell than down, we do nothing and let LabVIEW give click-and-drag selection for FREE! Of course, we still\nneed to coerce selection to be within data bounds."
        n139 = event-data() -> ("CtlRef"=w269:refnum<vi>)  [unwired: 1 in, 4 out]
        n140 = call "CoerceSelection.vi"("error in (no error)"=w270, "SetList Table ref"=w269) -> ()  [unwired: 9 in, 1 out]
      }
      event "SetList Table": Shortcut Menu Activation? {
        # "No need for DeferPanUpdts here..."
        # "click within selection?"
        # "row type set after determining click is in a \nvalid column. (Mouse down? event)"
        # "Removed all right-clicks that aren't in a data column\nin Mouse Down? event..."
        n141 = event-data() -> ("CtlRef"=w301:refnum<vi>, "Coords"=w300:T17, "MenuRef"=w289:refnum<k9>)  [unwired: 1 in]
        n142 = invoke class="Tbl (strict)" method="Point To Row Column"(reference=w301, error in=w302, "Point"=w300) -> (reference out=w293:refnum<vi>, error out=w291:errorcluster, "CellPosition"=w281:T4)  [unwired: 3 in, 3 out]
        n143 = Unbundle By Name(w281) -> ("Column"=w298:i32)
        n144 = local read "Col array"() -> (w272:refnum<class "Column.lvclass">[])
        n145 = control-ref of="VariableManager"() -> (w271:refnum<vi>)
        n146 = property class="Tbl (strict)"(reference=w293, error in=w291) -> (reference out=w292:refnum<vi>, error out=w290:errorcluster, "Selection Size"=w288:T4, "Selection Start"=w287:T4)
        n147 = Index Array(array=w272, index=w298) -> (element=w299:refnum<class "Column.lvclass">)
        n148 = Add(x=w288, y=w287) -> (x+y=w296:T4)
        n149 = control-ref of="Clipboard"() -> (w283:refnum<vi>)
        n150 = local read "Button\n(Mouse Down?)"() -> (w282:u16)
        n151 = Greater?(x=w296, y=w281) -> (0:w295:cluster{"Row":bool, "Column":bool})
        n152 = Less Or Equal?(x=w287, y=w281) -> (x <= y?=w294:cluster{"Row":bool, "Column":bool})
        n153 = And(x=w295, y=w294) -> (x .and. y?=w286:cluster{"Row":bool, "Column":bool})
        n154 = Cluster To Array(cluster=w286) -> (array=w285:bool[])
        n155 = local read "FunctionMenu"() -> (w275:refnum<class "InsertFunctionMenu.lvclass">)
        n156 = And Array Elements(Boolean array=w285) -> (logical AND=w284:bool)
        "withinSelection?" <- w284
        n157 = call-dynamic "MenuBuild.vi"("Column in"=w299, "row type"="row type", "Clipboard"=w283, "MenuRef In"=w289, "Click Position"=w281, "Table CtlRef In"=w292, "error in (no error)"=w290, "withinSelection?"=w284, "Button\n(Mouse Down?)"=w282) -> ("MenuRef Out"=w280:refnum<k9>, "error out"=w279:errorcluster)  [unwired: 3 in, 2 out]
        n158 = call "InsertVariableMenuBuild.vi"("error in (no error)"=w279, "Insert Tag"="USERVAR_TOP", "menu reference in"=w280, "VariableManager Ref in"=w271) -> ("error out"=w277:errorcluster, "menu reference out"=w274:refnum<k9>)  [unwired: 6 in]
        n159 = call-dynamic "MenuBuild.vi"("error in (no error)"=w277, "Insert Tag"="USERFUNC_TOP", "menu reference"=w274, "InsertFunctionMenu in"=w275) -> ("error out"=w276:errorcluster)  [unwired: 5 in, 2 out]
        n160 = event-data() -> ()  [unwired: 2 in, 1 out]
      }
      event "SetList Table": Shortcut Menu Selection (User) {
        # "Don't check error or panel it\nmay prevent panel being updated!"
        n161 = event-data() -> ("CtlRef"=w326:refnum<vi>, "Coords"=w335:T17, "ItemTag"=w334:string)  [unwired: 1 in, 2 out]
        n162 = local read "Defer Updates?"() -> (w327:bool)
        n163 = invoke class="Tbl (strict)" method="Point To Row Column"(reference=w326, error in=w336, "Point"=w335) -> (reference out=w317:refnum<vi>, error out=w319:errorcluster, "CellPosition"=w333:T4)  [unwired: 3 in, 3 out]
        n164 = property class="Tbl (strict)"(reference=w317, error in=w319) -> (reference out=w316:refnum<vi>, error out=w318:errorcluster, "Value"=w315:string[][])
        n165 = local read "Devices queue"() -> (w311:refnum<queue>)
        n166 = local read "DevNums"() -> (w323:i32[])
        n167 = call "DefPnlAndCursor.vi"("AllowDefPan? (T)"=w327, "error in (no error)"=w318, "DeferPanUpdts?"=TRUE ("DeferPanUPdts?"), "Tbl Ctrl Refnum"=w316) -> ("error out"=w321:errorcluster)  [unwired: 7 in]
        n168 = control-ref of="VariableManager"() -> (w306:refnum<vi>)
        n169 = control-ref of="FunctionMenu"() -> (w308:refnum<vi>)
        n170 = call "ModeFromDevices.vi"("error in (no error)"=w321, "Devices queue"=w311) -> ("error out"=w322:errorcluster, "Mode Col"=w325:i32)  [unwired: 8 in]
        n171 = control-ref of="Table History"() -> (w309:refnum<vi>)
        n172 = control-ref of="Clipboard"() -> (w303:refnum<vi>)
        n173 = control-ref of="Col array"() -> (w304:refnum<vi>)
        n174 = control-ref of="Select Layout"() -> (w305:refnum<vi>)
        n175 = call "SetList SWI to Devices.vi"("error in (no error)"=w322, "SWI table"=w315, "DevNums In"=w323, "Devices queue"=w311) -> ("error out"=w320:errorcluster, "Devices queue out"=w312:refnum<queue>)  [unwired: 5 in, 1 out]
        n176 = Unbundle By Name(w333) -> ("Column"=w314:i32)
        n177 = local read "Col array"() -> (w313:refnum<class "Column.lvclass">[])
        n178 = Bundle By Name(cluster=T18 {"Clipboard"=refnum, "Layout Ring Refnum"=refnum, "Col Array Ref in"=refnum, "VariableManagerRef"=refnum, "Table CtlRef In"=refnum, "Table History ref"=refnum, "Devices queue"=refnum, "FunctionMenu Ref"=refnum} ("SetList Refs"), "Devices queue"=w312, "Clipboard"=w303, "Layout Ring Refnum"=w305, "Col Array Ref in"=w304, "VariableManagerRef"=w306, "Table CtlRef In"=w317, "Table History ref"=w309, "FunctionMenu Ref"=w308) -> (w310:T18)
        n179 = Index Array(array=w313, index=w314) -> (element=w332:refnum<class "Column.lvclass">)
        n180 = call-dynamic "MenuDo.vi"("ModeCol Index"=w325, "Cell Position"=w333, "error in (no error)"=w320, "SetList Refs"=w310, "ItemTag"=w334, "Column in"=w332) -> ("error out"=w331:errorcluster, "Update HWI?"=w324:bool)  [unwired: 1 in, 3 out]
        n181 = call "DefPnlAndCursor.vi"("AllowDefPan? (T)"=w327, "error in (no error)"=w331, "DeferPanUpdts?"=FALSE ("DeferPanUPdts?"), "Tbl Ctrl Refnum"=w317) -> ("error out"=w330:errorcluster)  [unwired: 7 in]
        n182 = case shown="True" w324 {
          frame False {
          }
          frame True {
            n183 = global read "PrefsGlobal.vi" "SetListPrefs.lvclass"() -> (w338:refnum<class "SetListPrefs.lvclass">)
            n184 = call "Read AutoPressHWUpdate.vi"("SetListPrefs in"=w338) -> ("AutoPressHWUpdate"=w337:bool)  [unwired: 8 in, 2 out]
            n185 = case shown="True" w337 {
              frame False {
                n186 = property on="UpdateHWI Button" class="Bool (strict)"("DisabledEnum"=T12."Enabled" ("Disabled")) -> ()  [unwired: 2 in, 2 out]
              }
              frame True {
                n187 = property on="UpdateHWI Button" class="Bool (strict)"("Val(Sgnl)"=TRUE ("Value (Signaling)")) -> ()  [unwired: 2 in, 2 out]
              }
            }
          }
        }
      }
      event "SetList Table": Mouse Enter {
        # "Change to hand inside table"
        n188 = event-data() -> ()  [unwired: 1 in, 1 out]
        n189 = call-poly <vilib>:"Set Cursor.vi"("error in (no error)"=w342, "icon"=6) -> ("error out"=w341:errorcluster)  [unwired: 8 in, 1 out]
      }
      event "SetList Table": Mouse Leave {
        # "Change back to default pointer outside table control"
        n190 = event-data() -> ()  [unwired: 1 in, 1 out]
        n191 = call-poly <vilib>:"Set Cursor.vi"("error in (no error)"=w345, "icon"=0) -> ("error out"=w344:errorcluster)  [unwired: 8 in, 1 out]
      }
      event "User defined functions": Value Change {
        # "Closing allows a user to delete\na \"defined function\" simply by \nremoving it. Then only what remains\nis re-registered.\n\n(This also throws away cached variables!)"
        n192 = event-data() -> ("OldVal"=w352:string, "NewVal"=w347:string)  [unwired: 1 in, 1 out]
        n193 = call "Caching_Expression_Evaluator_Table.vi"("method"=t_Caching_Expression_Evaluator_Methods_Table."close", "error in (no error)"=w350) -> ("error out"=w349:errorcluster)  [unwired: 11 in, 2 out]
        n194 = call "Caching_Expression_Evaluator_Table.vi"("method"=t_Caching_Expression_Evaluator_Methods_Table."execute", "expression/scriptlet"=w347, "error in (no error)"=w349) -> ("error out"=w354:errorcluster)  [unwired: 10 in, 2 out]
        n195 = case shown="Error" w354 {
          selector: w354 -> [_ w363]
          tunnel: [w359 errorcluster {"status"=FALSE, "code"=0, "source"=""} ("error out")] -> w353
          tunnel: w352 -> [_ w367]
          tunnel: w347 -> [w360 _]
          frame No Error {
            # "successful function \"registration\"; all other \"caching eval table\" calls will know functions now"
            n196 = global read "PrefsGlobal.vi" "SetListPrefs.lvclass"() -> (w355:refnum<class "SetListPrefs.lvclass">)
            n197 = local read "FunctionMenu"() -> (w358:refnum<class "InsertFunctionMenu.lvclass">)
            n198 = call-dynamic "ParseUserFunctions.vi"("User defined functions in"=w360, "FunctionMenu in"=w358) -> ("error out"=w359:errorcluster, "FunctionMenu out"=w357:refnum<class "InsertFunctionMenu.lvclass">)  [unwired: 8 in]
            n199 = call "Read AutoPressHWUpdate.vi"("SetListPrefs in"=w355) -> ("AutoPressHWUpdate"=w356:bool)  [unwired: 8 in, 2 out]
            n200 = local write "FunctionMenu"(w357) -> ()
            n201 = case shown="True" w356 {
              frame False {
                n202 = property on="UpdateHWI Button" class="Bool (strict)"("DisabledEnum"=T12."Enabled" ("Disabled")) -> ()  [unwired: 2 in, 2 out]
              }
              frame True {
                n203 = property on="UpdateHWI Button" class="Bool (strict)"("Val(Sgnl)"=TRUE ("Value (Signaling)")) -> ()  [unwired: 2 in, 2 out]
              }
            }
          }
          frame Error {
            # "reset old, valid functions"
            # "on parsing error: reset functions to last, Clear error (and present warning dialog)"
            n204 = call "Caching_Expression_Evaluator_Table.vi"("method"=t_Caching_Expression_Evaluator_Methods_Table."execute", "expression/scriptlet"=w367) -> ("error out"=w365:errorcluster)  [unwired: 11 in, 2 out]
            n205 = Merge Errors(w365, w363) -> (w364:errorcluster)
            n206 = local write "User defined functions"(w367) -> ()
            n207 = disable-structure shown="Enabled" {
              disable-tunnel: w364 -> [w372 _]
              frame Enabled {
                w374 = T26 1 items=["no dialog", "OK message", "continue or stop message", "OK message + warnings", "continue/stop + warnings"] ("type of dialog (OK msg:1)")
                n208 = Unbundle By Name(w372) -> ("source"=w370:string)
                n209 = Concatenate Strings("\n*User Functions* error: \n" ("string"), w370) -> (w371:string)
                n210 = Bundle By Name(cluster=w372, "source"=w371) -> (w373:errorcluster)
                n211 = call <vilib>:"Simple Error Handler.vi"("type of dialog (OK msg:1)"=w374, "error in (no error)"=w373) -> ()  [unwired: 3 in, 5 out]
              }
              frame Disabled {
              }
            }
          }
        }
      }
      event Panel Resize {
        # "Resize the tab & table controls to match window size"
        n212 = event-data() -> ("NewBnds"=w388:T13)  [unwired: 1 in]
        n213 = Unbundle By Name(w388) -> ("Right"=w387:i16, "Left"=w386:i16, "Bottom"=w384:i16, "Top"=w383:i16)
        n214 = Subtract(x=w387, y=w386) -> (x-y=w385:i16)
        n215 = Subtract(x=w384, y=w383) -> (x-y=w382:i16)
        n216 = Subtract(x=w385, y=u32 24) -> (x-y=w375:u32)
        n217 = Subtract(x=w382, y=u32 85) -> (x-y=w376:u32)
        n218 = property on="Tab Control" class="TabCtl (strict)"("PaneWidth"=w375, "PaneHeight"=w376) -> (error out=w377:errorcluster)  [unwired: 2 in, 1 out]
        n219 = Subtract(x=w375, y=u32 16) -> (x-y=w379:u32)
        n220 = Subtract(x=w376, y=u32 86) -> (x-y=w378:u32)
        n221 = property on="SetList Table" class="Tbl (strict)"(error in=w377, "Width"=w379, "Height"=w378) -> ()  [unwired: 1 in, 2 out]
      }
      event "Select Layout": Value Change {
        n222 = event-data() -> ("NewVal"=w396:i32)  [unwired: 1 in]
        n223 = local read "Defer Updates?"() -> (w395:bool)
        n224 = local read "Col array"() -> (w391:refnum<class "Column.lvclass">[])
        n225 = call "ApplySelectedLayout.vi"("Defer Updates? (T)"=w395, "error in (no error)"=w394, "Layout index"=w396, "Col array"=w391, "Tbl Refnum"=w392) -> ("error out"=w393:errorcluster)  [unwired: 6 in]
      }
      event "ConfigLayoutsButton": Value Change {
        # "Make sure col array is updated \nwith \"filmstrip\" sequence!"
        # "Want preview of layouts as we make them\n-->VI gets panel reference from table control to defer updates as required."
        n226 = event-data() -> ()  [unwired: 1 in, 3 out]
        n227 = disable-structure shown="Enabled" {
          frame Enabled {
            # "reset button"
            n228 = local write "ConfigLayoutsButton"(FALSE) -> ()
          }
          frame Disabled {
          }
        }
        n229 = flat-sequence {
          tunnel: w400 -> [w413]
          tunnel: [w409] -> w399
          tunnel: [w405] -> w397
          tunnel: [w417] -> w398
          tunnel: w399 -> [w418]
          tunnel: w397 -> [w415]
          frame #0 {
            n230 = local read "Devices queue"() -> (w402:refnum<queue>)
            n231 = local read "Defer Updates?"() -> (w410:bool)
            n232 = local read "DevNums"() -> (w408:i32[])
            n233 = control-ref of="SetList Table"() -> (w412:refnum<vi>)
            n234 = control-ref of="Col array"() -> (w401:refnum<vi>)
            n235 = control-ref of="Select Layout"() -> (w411:refnum<vi>)
            n236 = Dequeue Element(queue=w402) -> (queue out=w407:refnum<queue>, element=w404:refnum<class "Device.lvclass">[], error out=w406:errorcluster)  [unwired: 2 in, 1 out]
            n237 = call "GetNameList.vi"("Devices"=w404) -> ("Names in use"=w403:string[])  [unwired: 8 in, 2 out]
            n238 = call "ConfigLayouts.vi"("DevNums"=w408, "Dev Names"=w403, "Defer Updates? (True)"=w410, "Tbl Refnum"=w412, "error in (no error)"=w413, "Col Array Refnum"=w401, "Layout Ring Refnum"=w411) -> ("error out"=w409:errorcluster)  [unwired: 4 in]
            n239 = Enqueue Element(queue=w407, element=w404, error in (no error)=w406) -> (queue out=w405:refnum<queue>)  [unwired: 1 in, 2 out]
          }
          frame #1 {
            # "Need to push appearance changes\nto the columns! (or change layout\nto act on devices...)"
            n240 = local read "Col array"() -> (w414:refnum<class "Column.lvclass">[])
            n241 = local read "DevNums"() -> (w416:i32[])
            n242 = call "SetList Columns to Devices.vi"("error in (no error)"=w418, "Col array in"=w414, "DevNums In"=w416, "Devices queue"=w415) -> ("error out"=w417:errorcluster)  [unwired: 6 in, 1 out]
          }
        }
      }
      event "FitCol2Text Button": Value Change {
        # "Resizes all displayed columns"
        n243 = event-data() -> ()  [unwired: 1 in, 3 out]
        n244 = local read "Col array"() -> (w420:refnum<class "Column.lvclass">[])
        n245 = local read "Defer Updates?"() -> (w422:bool)
        n246 = local read "Select Layout"() -> (w423:i32)
        n247 = local write "FitCol2Text Button"(FALSE ("FitCol2Text Button")) -> ()
        n248 = call "FitCol2Text.vi"("Defer Updates?"=w422, "error in (no error)"=w425, "SetList Table ref"=w424, "Col array"=w420, "Select Layout"=w423) -> ("error out"=w421:errorcluster)  [unwired: 6 in]
      }
      event "ManageDevicesButton": Value Change {
        # "push SWI to devices (so they can operate\non it easily if column #s change)"
        n249 = event-data() -> ()  [unwired: 1 in, 3 out]
        n250 = local read "Devices queue"() -> (w429:refnum<queue>)
        n251 = local read "DevNums"() -> (w436:i32[])
        n252 = control-ref of="SetList Table"() -> (w438:refnum<vi>)
        n253 = property class="Tbl (strict)"(reference=w438) -> (reference out=w437:refnum<vi>, error out=w435:errorcluster, "Value"=w434:string[][])  [unwired: 1 in]
        n254 = control-ref of="Select Layout"() -> (w439:refnum<vi>)
        n255 = local read "Col array"() -> (w428:refnum<class "Column.lvclass">[])
        n256 = local read "DevNums"() -> (w440:i32[])
        n257 = control-ref of="Table History"() -> (w432:refnum<vi>)
        n258 = call "SetList SWI to Devices.vi"("error in (no error)"=w435, "SWI table"=w434, "DevNums In"=w436, "Devices queue"=w429) -> ("Devices queue out"=w431:refnum<queue>)  [unwired: 5 in, 2 out]
        n259 = call "Manage Devices.vi"("Devices queue"=w431, "Table Ref In"=w437, "DevNums In"=w440, "Col array in"=w428, "Table History ref"=w432, "Layout ref"=w439) -> ("Changes Made?"=w433:bool, "DevNums Out"=w430:i32[], "Col array out"=w427:refnum<class "Column.lvclass">[])  [unwired: 1 in, 1 out]
        n260 = case shown="True" w433 {
          frame False {
          }
          frame True {
            n261 = global read "PrefsGlobal.vi" "SetListPrefs.lvclass"() -> (w442:refnum<class "SetListPrefs.lvclass">)
            n262 = call "Read AutoPressHWUpdate.vi"("SetListPrefs in"=w442) -> ("AutoPressHWUpdate"=w443:bool)  [unwired: 8 in, 2 out]
            n263 = case shown="True" w443 {
              frame False {
                n264 = property on="UpdateHWI Button" class="Bool (strict)"("DisabledEnum"=T12."Enabled" ("Disabled")) -> ()  [unwired: 2 in, 2 out]
              }
              frame True {
                n265 = property on="UpdateHWI Button" class="Bool (strict)"("Val(Sgnl)"=TRUE ("Value (Signaling)")) -> ()  [unwired: 2 in, 2 out]
              }
            }
          }
        }
        n266 = local write "Col array"(w427) -> ()
        n267 = local write "DevNums"(w430) -> ()
        n268 = local write "ManageDevicesButton"(FALSE) -> ()
      }
      event "quit": Value Change {
        # "These prefs aren't used after startup, so we only bother writing on quit"
        # "Need to close viewer?"
        # "store devices state on Quit.\nThis should be the ONLY local variable call!!!"
        # "Save SWI to device array. If VI is restarted, the table will be re-initialized\nfrom device array, erasing any bug-causing user edits to table control\nthe user made while VI was stopped."
        # "Stop VMUI when stopping SetList (otherwise Actor stays in memory until LabView closed.)"
        n269 = event-data() -> ("NewVal"=w471:bool)  [unwired: 1 in, 1 out]
        n270 = control-ref of="SetList Table"() -> (w470:refnum<vi>)
        n271 = control-ref of="VariableManager"() -> (w448:refnum<vi>)
        n272 = property class="Tbl (strict)"(reference=w470, error in=w466) -> (error out=w468:errorcluster, "Value"=w467:string[][])  [unwired: 1 out]
        n273 = disable-structure shown="Enabled" {
          frame Enabled {
            # "this goes a long way towards solving bug where\nvariables/functions persist after VI is stopped.\nWe'll also need to add this to Save/Load AND \nmake sure to \"nil\" deleted variables from VM."
            # "test closing Lua state"
            n274 = call "Caching_Expression_Evaluator_Table.vi"("method"=t_Caching_Expression_Evaluator_Methods_Table."close") -> ()  [unwired: 12 in, 3 out]
          }
          frame Disabled {
          }
        }
        n275 = local read "Devices queue"() -> (w447:refnum<queue>)
        n276 = local read "DevNums"() -> (w469:i32[])
        n277 = call "VMUIStop.vi"("VariableManagerRef in"=w448) -> ()  [unwired: 9 in, 2 out]
        n278 = call "SetList SWI to Devices.vi"("error in (no error)"=w468, "SWI table"=w467, "DevNums In"=w469, "Devices queue"=w447) -> ("error out"=w461:errorcluster, "Devices queue out"=w464:refnum<queue>)  [unwired: 5 in, 1 out]
        n279 = Dequeue Element(queue=w464) -> (queue out=w463:refnum<queue>, element=w446:refnum<class "Device.lvclass">[], error out=w462:errorcluster)  [unwired: 2 in, 1 out]
        n280 = global read "PrefsGlobal.vi" "SetListPrefs.lvclass"() -> (w459:refnum<class "SetListPrefs.lvclass">)
        n281 = local write "Devices"(w446) -> ()
        n282 = property on="Load Recent" class="CmbBox"() -> (error out=w458:errorcluster, "Strings[]"=w457:string[])  [unwired: 2 in, 1 out]
        n283 = Release Queue(queue=w463, error in (no error)=w462) -> ()  [unwired: 1 in, 3 out]
        n284 = call "Write LoadRecentContents.vi"("error in (no error)"=w458, "LoadRecentContents"=w457, "SetListPrefs in"=w459) -> ("error out"=w455:errorcluster, "SetListPrefs out"=w456:refnum<class "SetListPrefs.lvclass">)  [unwired: 7 in]
        n285 = call "Write ResetPositionAtStartup.vi"("error in (no error)"=w455, "ResetPositionAtStartup"="Reset at Startup", "SetListPrefs in"=w456) -> ("error out"=w451:errorcluster, "SetListPrefs out"=w452:refnum<class "SetListPrefs.lvclass">)  [unwired: 7 in]
        n286 = call "Write DetachVMUIonStart.vi"("error in (no error)"=w451, "DetachVMUIonStart"="DetachVMUIonStart", "SetListPrefs in"=w452) -> ("error out"=w453:errorcluster, "SetListPrefs out"=w454:refnum<class "SetListPrefs.lvclass">)  [unwired: 7 in]
        n287 = local write "quit"(FALSE ("quit")) -> ()
        n288 = call "SaveOnly.vi"("error in (no error)"=w453, "Preferences in"=w454) -> ()  [unwired: 7 in, 3 out]
        "TCP Quit Signal" <- TRUE ("TCP Quit Signal")
      }
      event "Undo": Value Change {
        n289 = event-data() -> ()  [unwired: 1 in, 3 out]
        n290 = local read "Defer Updates?"() -> (w481:bool)
        n291 = disable-structure shown="Enabled" {
          disable-tunnel: [w495 w497] -> w478
          disable-tunnel: w482 -> [w494 w497]
          disable-tunnel: w481 -> [w493 _]
          disable-tunnel: w480 -> [w492 _]
          frame Disabled {
            n292 = call "DefPnlAndCursor.vi"("AllowDefPan? (T)"=w493, "error in (no error)"=w494, "DeferPanUpdts?"=TRUE ("DeferPanUPdts?"), "Tbl Ctrl Refnum"=w492) -> ("error out"=w495:errorcluster)  [unwired: 7 in]
          }
          frame Enabled {
          }
        }
        n293 = local write "Undo"(FALSE ("Undo")) -> ()
        n294 = local read "Devices queue"() -> (w474:refnum<queue>)
        n295 = call "ModeFromDevices.vi"("error in (no error)"=w478, "Devices queue"=w474) -> ("error out"=w477:errorcluster, "Mode Col"=w479:i32)  [unwired: 8 in]
        n296 = local read "Col array"() -> (w473:refnum<class "Column.lvclass">[])
        n297 = control-ref of="Select Layout"() -> (w486:refnum<vi>)
        n298 = control-ref of="Table History"() -> (w488:refnum<vi>)
        n299 = control-ref of="SetList Table"() -> (w489:refnum<vi>)
        n300 = call "Un(Re)doTblChng.vi"("Undo/Redo"=enum16{"Undo", "Redo"}."Undo", "ModeCol Index"=w479, "Layout Ref"=w486, "error in (no error)"=w477, "Table CtlRef In"=w489, "Col Array in"=w473, "Table History ref"=w488) -> ("error out"=w484:errorcluster)  [unwired: 4 in]
        n301 = disable-structure shown="Enabled" {
          disable-tunnel: w484 -> [w501 w503]
          disable-tunnel: [w500 w503] -> w483
          disable-tunnel: w481 -> [w499 _]
          disable-tunnel: w480 -> [w498 _]
          frame Disabled {
            n302 = call "DefPnlAndCursor.vi"("AllowDefPan? (T)"=w499, "error in (no error)"=w501, "DeferPanUpdts?"=FALSE ("DeferPanUPdts?"), "Tbl Ctrl Refnum"=w498) -> ("error out"=w500:errorcluster)  [unwired: 7 in]
          }
          frame Enabled {
          }
        }
        n303 = global read "PrefsGlobal.vi" "SetListPrefs.lvclass"() -> (w476:refnum<class "SetListPrefs.lvclass">)
        n304 = call "Read AutoPressHWUpdate.vi"("SetListPrefs in"=w476) -> ("AutoPressHWUpdate"=w475:bool)  [unwired: 8 in, 2 out]
        n305 = case shown="True" w475 {
          frame False {
            n306 = property on="UpdateHWI Button" class="Bool (strict)"("DisabledEnum"=T12."Enabled" ("Disabled")) -> ()  [unwired: 2 in, 2 out]
          }
          frame True {
            n307 = property on="UpdateHWI Button" class="Bool (strict)"("Val(Sgnl)"=TRUE ("Value (Signaling)")) -> ()  [unwired: 2 in, 2 out]
          }
        }
      }
      event "Redo": Value Change {
        n308 = event-data() -> ()  [unwired: 1 in, 3 out]
        n309 = local read "Defer Updates?"() -> (w510:bool)
        n310 = disable-structure shown="Enabled" {
          disable-tunnel: w514 -> [w525 w527]
          disable-tunnel: [w524 w527] -> w513
          disable-tunnel: w510 -> [w523 _]
          disable-tunnel: w509 -> [w522 _]
          frame Disabled {
            n311 = call "DefPnlAndCursor.vi"("AllowDefPan? (T)"=w523, "error in (no error)"=w525, "DeferPanUpdts?"=TRUE ("DeferPanUPdts?"), "Tbl Ctrl Refnum"=w522) -> ("error out"=w524:errorcluster)  [unwired: 7 in]
          }
          frame Enabled {
          }
        }
        n312 = local write "Redo"(FALSE) -> ()
        n313 = local read "Devices queue"() -> (w505:refnum<queue>)
        n314 = local read "Col array"() -> (w504:refnum<class "Column.lvclass">[])
        n315 = control-ref of="Select Layout"() -> (w515:refnum<vi>)
        n316 = control-ref of="Table History"() -> (w518:refnum<vi>)
        n317 = control-ref of="SetList Table"() -> (w519:refnum<vi>)
        n318 = call "ModeFromDevices.vi"("Devices queue"=w505) -> ("Mode Col"=w508:i32)  [unwired: 9 in, 1 out]
        n319 = call "Un(Re)doTblChng.vi"("Undo/Redo"=enum16{"Undo", "Redo"}."Redo", "ModeCol Index"=w508, "Layout Ref"=w515, "error in (no error)"=w513, "Table CtlRef In"=w519, "Col Array in"=w504, "Table History ref"=w518) -> ("error out"=w511:errorcluster)  [unwired: 4 in]
        n320 = global read "PrefsGlobal.vi" "SetListPrefs.lvclass"() -> (w507:refnum<class "SetListPrefs.lvclass">)
        n321 = disable-structure shown="Enabled" {
          disable-tunnel: [w531 w533] -> w512
          disable-tunnel: w511 -> [w530 w533]
          disable-tunnel: w510 -> [w529 _]
          disable-tunnel: w509 -> [w528 _]
          frame Disabled {
            n322 = call "DefPnlAndCursor.vi"("AllowDefPan? (T)"=w529, "error in (no error)"=w530, "DeferPanUpdts?"=FALSE ("DeferPanUPdts?"), "Tbl Ctrl Refnum"=w528) -> ("error out"=w531:errorcluster)  [unwired: 7 in]
          }
          frame Enabled {
          }
        }
        n323 = call "Read AutoPressHWUpdate.vi"("SetListPrefs in"=w507) -> ("AutoPressHWUpdate"=w506:bool)  [unwired: 8 in, 2 out]
        n324 = case shown="True" w506 {
          frame False {
            n325 = property on="UpdateHWI Button" class="Bool (strict)"("DisabledEnum"=T12."Enabled" ("Disabled")) -> ()  [unwired: 2 in, 2 out]
          }
          frame True {
            n326 = property on="UpdateHWI Button" class="Bool (strict)"("Val(Sgnl)"=TRUE ("Value (Signaling)")) -> ()  [unwired: 2 in, 2 out]
          }
        }
      }
      event "Launch Viewer": Value Change {
        w538 = refnum<vi> refnum  # type specifier VI Refnum (for type only)
        # "When to close?\nAlso need to handle multiple button presses (they add calls\nto a queue which get called when Viewer \"Close\" is pressed.)"
        # "call and forget."
        # "Asynchronous viewer call (don't block execution in SetList)."
        n327 = event-data() -> ()  [unwired: 1 in, 6 out]
        n328 = control-ref of="Procedure Repository"() -> (w540:refnum<vi>)
        n329 = control-ref of="Git Command"() -> (w539:refnum<vi>)
        n330 = control-ref of="Col array"() -> (w537:refnum<vi>)
        n331 = control-ref of="Clipboard"() -> (w543:refnum<vi>)
        n332 = control-ref of="Select Layout"() -> (w541:refnum<vi>)
        n333 = control-ref of="VariableManager"() -> (w536:refnum<vi>)
        n334 = local read "Devices queue"() -> (w535:refnum<queue>)
        n335 = local write "Launch Viewer"(FALSE ("Launch Viewer")) -> ()
        n336 = Open VI Reference(type specifier VI Refnum (for type only)=w538, vi path=path "Utils/Viewer.vi", options=128) -> (vi reference=w545:refnum<vi>, error out=w544:errorcluster)  [unwired: 3 in]
        n337 = call-by-ref "Start Asynchronous Call"(reference=w545, error in=w544, "Col Array Refnum"=w537, "RepoPath Refnum"=w540, "SetList Layout Ref"=w541, "GitCmd Refnum"=w539, "SetList Dev queue"=w535, "SetList VariableManager ref"=w536, "SetList Clipboard ref"=w543) -> (reference out=→"Viewer ref":refnum<vi>)  [unwired: 5 in, 1 out]
      }
      event "Save to File", "Save to Repo": Value Change {
        n338 = event-data() -> ("CtlRef"=w551:refnum<vi>, "NewVal"=w552:bool)  [unwired: 1 in, 1 out]
        n339 = property class="Bool (strict)"(reference=w551) -> ("Label.Text"=w550:string)  [unwired: 1 in, 2 out]
        n340 = property on="Save to Repo" class="Bool (strict)"() -> ("Label.Text"=w549:string)  [unwired: 2 in, 2 out]
        n341 = Equal?(x=w549, y=w550) -> (x = y?=w548:bool)
        n342 = case shown="True" w552 {
          tunnel: w548 -> [_ w555]
          frame False {
          }
          frame True {
            # "Also need to push SWI to devices prior to saving!\nWhat about HWI?"
            n343 = local read "Devices queue"() -> (w560:refnum<queue>)
            n344 = local read "DevNums"() -> (w573:i32[])
            n345 = property on="SetList Table" class="Tbl (strict)"() -> (error out=w572:errorcluster, "Value"=w568:string[][])  [unwired: 2 in, 1 out]
            n346 = property on="Select Layout" class="Ring (strict)"() -> ("Value"=w558:i32, "StringsAndValues[]"=w557:T20)  [unwired: 2 in, 2 out]
            n347 = local read "User defined functions"() -> (w556:string)
            n348 = control-ref of="VariableManager"() -> (w562:refnum<vi>)
            n349 = Current VI's Path() -> (path=w567:path)
            n350 = call "SetList SWI to Devices.vi"("error in (no error)"=w572, "SWI table"=w568, "DevNums In"=w573, "Devices queue"=w560) -> ("error out"=w571:errorcluster, "Devices out"=w561:refnum<class "Device.lvclass">[])  [unwired: 5 in, 1 out]
            n351 = call "VMExport.vi"("VariableManagerRef in"=w562) -> ("VariableManagerExportCopy"=w563:refnum<class "VariableManager.lvclass">)  [unwired: 8 in, 2 out]
            n352 = call "GetVersionString.vi"("SetList root path"=w567) -> ("Version String"=w566:string)  [unwired: 2 in]
            n353 = Bundle By Name(cluster=T19 {"Version"="", "Devices"=[], "Select Layout"=0, "Layout:Strings And Values []"=[], "User defined functions"="", "VariableManager"=refnum}, "Version"=w566, "Devices"=w561, "Select Layout"=w558, "Layout:Strings And Values []"=w557, "User defined functions"=w556, "VariableManager"=w563) -> (w564:T19)
            n354 = case shown="True" w555 {
              tunnel: w571 -> [w588 w609]
              tunnel: ["<FromFile>" ("Hash") w590] -> w570
              tunnel: [w577 w606] -> w569
              tunnel: [w583 w602] -> w565
              tunnel: w564 -> [w587 w600]
              tunnel: [w584 w596] -> w554
              tunnel: [w574 w589] -> w553
              frame False {
                w581 = "<Loaded from file>" ("Loaded Description")
                # "Save to File"
                n355 = call "Save_v5.vi"("error in"=w588, "Save Cluster"=w587) -> ("error out"=w578:errorcluster, "cancelled"=w579:bool, "Procedure Name"=w585:string, "Chosen Path"=w575:path)  [unwired: 6 in]
                n356 = local write "Save to File"(FALSE ("Load from Disk")) -> ()
                n357 = Or(x=w579, y=w578) -> (x .or. y?=w577:bool)
                n358 = Path To String(path=w575) -> (string=w574:string)
                n359 = Bundle By Name(cluster=T21 {"Title"="", "Description"="", "Author"=""} ("Commit Meta-Info"), "Title"=w585, "Description"=w581, "Author"=w581) -> (w583:T21)
                n360 = Concatenate Strings("From File: " ("string"), w574) -> (w584:string)
              }
              frame True {
                # "Save to Repo"
                n361 = local read "Git Command"() -> (w603:string)
                n362 = local read "Procedure Repository"() -> (w594:path)
                n363 = property on="Author" class="Ring (strict)"() -> ("RingText.Text"=w607:string)  [unwired: 2 in, 2 out]
                n364 = local write "Save to Repo"(FALSE ("Load from Disk")) -> ()
                n365 = Bundle By Name(cluster=T21 {"Title"="", "Description"="", "Author"=""} ("Commit Meta-Info"), "Title"="SaveTitle", "Description"="Description (Repo Only)", "Author"=w607) -> (w602:T21)
                n366 = call "GitSave.vi"("Commit Meta-Info"=w602, "Make LAST_SAVED"=TRUE, "error in (no error)"=w609, "Save Repo Path"=w594, "Save Cluster"=w600, "Git exec"=w603) -> ("error out"=w604:errorcluster, "User Cancelled"=w605:bool, "Saved Hash"=w590:string, "Git exec out"=w595:string)  [unwired: 2 in]
                n367 = Or(x=w605, y=w604) -> (x .or. y?=w606:bool)
                n368 = call "GitLog.vi"("Directory"=w594, "Number"=1, "Git exec"=w595) -> ("Directory out"=w591:path, "Commit Info"=w597:T22[], "Git exec out"=w592:string)  [unwired: 5 in, 1 out]
                n369 = call "GitGetFullHash.vi"("Directory"=w591, "Partial Hash"=w590, "Git exec"=w592) -> ("Full Hash"=w589:string)  [unwired: 5 in, 3 out]
                n370 = Index Array(array=w597) -> (element=w599:T22)  [unwired: 1 in]
                n371 = call "CommitCluster-to-MenuString.vi"("Commit"=w599) -> ("Menu String"=w596:string)  [unwired: 2 in]
              }
            }
            n372 = case shown="False" w569 {
              tunnel: w570 -> [w614 _]
              tunnel: w566 -> [w620 _]
              tunnel: w565 -> [w619 _]
              tunnel: w554 -> [w617 _]
              tunnel: w553 -> [w613 _]
              frame False {
                # "user saved!"
                n373 = Unbundle By Name(w619) -> ("Title"=w618:string, "Description"=w615:string)
                n374 = local write "Loaded Version"(w620) -> ()
                n375 = local write "Load Long Hash/Filename"(w613) -> ()
                n376 = local write "LoadHash"(w614) -> ()
                n377 = local write "Procedure Name"(w618) -> ()
                n378 = local write "Loaded Description"(w615) -> ()
                n379 = control-ref of="Load Recent"() -> (w622:refnum<vi>)
                n380 = call "Load_HistoryUpdate.vi"("Limit to 30"=TRUE, "History ref"=w622, "New Path"=w617) -> ()  [unwired: 1 in]
                n381 = Format Into String(format string="Based on %s (%s)\n%s", w614, w613, w615) -> (resulting string=w612:string)  [unwired: 2 in, 1 out]
                n382 = local write "Description (Repo Only)"(w612) -> ()
                "SaveHash" <- w614
              }
              frame True {
                # "user cancelled"
              }
            }
          }
        }
      }
      event "Load from Repo", "Load keep cur. format", "Load from File": Value Change {
        n383 = event-data() -> ("NewVal"=w628:bool)  [unwired: 1 in]
        n384 = local read "LoadRecentFile"() -> (w623:string)
        n385 = local read "Load from File"() -> (w625:bool)
        n386 = local read "LoadRecentHash"() -> (w626:string)
        n387 = String To Path(string=w623) -> (path=w624:path)
        n388 = case shown="True" w628 {
          tunnel: ["" ""] -> w627
          tunnel: w626 -> [_ w633]
          tunnel: w625 -> [_ w634]
          tunnel: w624 -> [_ w632]
          frame False {
          }
          frame True {
            w635 = FALSE ("Load from Disk")
            # "ToDo: Also need to initialize table from devices!!!"
            n389 = case shown="False" w634 {
              tunnel: [w644 w681] -> w643
              tunnel: [w657 w680] -> w642
              tunnel: [w646 w674] -> w641
              tunnel: [w648 w676] -> w640
              tunnel: [w656 "<Loaded from file>" ("Loaded Description")] -> w639
              tunnel: w633 -> [w653 _]
              tunnel: w632 -> [_ w670]
              tunnel: ["" w666] -> w631
              tunnel: [w645 w666] -> w630
              frame False {
                n390 = local read "Procedure Repository"() -> (w654:path)
                n391 = local read "Git Command"() -> (w655:string)
                n392 = call "GitLoad.vi"("Directory"=w654, "LoadThisHash"=w653, "Git exec"=w655) -> ("error out"=w651:errorcluster, "Directory out"=w650:path, "Save Cluster"=w657:T19, "Git exec out"=w649:string, "Loaded Description"=w656:string, "User Cancelled"=w644:bool, "Loaded Commit Info"=w648:T22)  [unwired: 2 in]
                n393 = Unbundle By Name(w648) -> ("Hash"=w647:string)
                n394 = case shown="False" w644 {
                  tunnel: w651 -> [w663 w665]
                  tunnel: w650 -> [w662 _]
                  tunnel: w649 -> [w661 _]
                  tunnel: w647 -> [w660 _]
                  tunnel: [w659 w665] -> w646
                  tunnel: [w658 ""] -> w645
                  frame False {
                    n395 = call "GitGetFullHash.vi"("error in (no error)"=w663, "Directory"=w662, "Partial Hash"=w660, "Git exec"=w661) -> ("error out"=w659:errorcluster, "Full Hash"=w658:string)  [unwired: 4 in, 2 out]
                  }
                  frame True {
                  }
                }
              }
              frame True {
                n396 = call "Load_v5.vi"("Path (open dialog)"=w670) -> ("error out"=w675:errorcluster, "cancelled"=w681:bool, "Procedure Name"=w677:string, "Chosen Path"=w667:path, "Save Cluster"=w680:T19)  [unwired: 6 in]
                n397 = File/Directory Info(path=w667, error in=w675) -> (last mod=w668:timestamp, error out=w674:errorcluster)  [unwired: 5 out]
                n398 = call "LVtoISO8601.vi"("Labview Timestamp"=w668) -> ("ISO8601 Timestamp"=w669:string)
                n399 = Path To String(path=w667) -> (string=w666:string)
                n400 = String Subset(string=w669, length (rest)=19 ("length (rest)")) -> (substring=w672:string)  [unwired: 1 in]
                n401 = Bundle By Name(cluster=T22 {"Hash"="", "Date"="", "Name"=""} ("Loaded Commit Info"), "Name"=w677, "Date"=w672, "Hash"="<FromFile>") -> (w676:T22)
              }
            }
            n402 = local write "Load from Repo"(w635) -> ()
            n403 = local write "Load from File"(w635) -> ()
            n404 = local read "Load keep cur. format"() -> (w638:bool)
            n405 = case shown="False" w643 {
              tunnel: w642 -> [w708 _]
              tunnel: w641 -> [w707 w722]
              tunnel: [FALSE ("Visible") _] -> w637
              tunnel: w640 -> [w699 _]
              tunnel: w639 -> [w683 _]
              tunnel: w638 -> [w697 _]
              tunnel: w634 -> [w687 _]
              tunnel: w631 -> [w688 _]
              tunnel: w630 -> [w684 _]
              frame False {
                # "user saved!"
                n406 = control-ref of="SetList Table"() -> (w704:refnum<vi>)
                n407 = Unbundle By Name(w699) -> ("Name"=w696:string, "Hash"=w685:string)
                n408 = case shown="True" w687 {
                  tunnel: w699 -> [w714 _]
                  tunnel: [w713 w717] -> w694
                  tunnel: w688 -> [_ w715]
                  frame False {
                    # "Save to Recent Menu"
                    n409 = call "CommitCluster-to-MenuString.vi"("Commit"=w714) -> ("Menu String"=w713:string)  [unwired: 2 in]
                  }
                  frame True {
                    # "Load from file"
                    n410 = Concatenate Strings("From File: " ("string"), w715) -> (w717:string)
                  }
                }
                n411 = local write "Procedure Name"(w696) -> ()
                n412 = local write "LoadHash"(w685) -> ()
                n413 = local write "Load Long Hash/Filename"(w684) -> ()
                n414 = control-ref of="VariableManager"() -> (w690:refnum<vi>)
                n415 = property on="Loading Text" class="Str"("Visible"=TRUE) -> ()  [unwired: 2 in, 2 out]
                n416 = Format Into String(format string="Based on %s (%s)\n%s", w685, w684, w683) -> (resulting string=w682:string)  [unwired: 2 in, 1 out]
                n417 = local read "Defer Updates?"() -> (w711:bool)
                n418 = local read "Devices queue"() -> (w689:refnum<queue>)
                n419 = global read "PrefsGlobal.vi" "SetListPrefs.lvclass"() -> (w702:refnum<class "SetListPrefs.lvclass">)
                n420 = local write "Description (Repo Only)"(w682) -> ()
                n421 = control-ref of="Select Layout"() -> (w709:refnum<vi>)
                n422 = local write "Loaded Description"(w683) -> ()
                n423 = local write "SaveTitle"(w696) -> ()
                n424 = control-ref of="Load Recent"() -> (w693:refnum<vi>)
                n425 = call "LoadedCluster_toSetList_v5.vi"("Devices queue"=w689, "Layout Ref"=w709, "Load w/o format? (F)"=w697, "Save Cluster"=w708, "Table Ref in"=w704, "VariableManagerRef"=w690, "error in (no error)"=w707, "Defer Updates? (T)"=w711) -> ("Loaded Version"=w710:string, "DevNums"=w712:i32[], "Col array"=w691:refnum<class "Column.lvclass">[], "User defined functions"=w703:string, "error out"=w698:errorcluster)  [unwired: 2 in, 1 out]
                n426 = disable-structure shown="Disabled" {
                  disable-tunnel: w703 -> [w720 w721]
                  frame Disabled {
                    n427 = local write "User defined functions"(w720) -> ()
                    n428 = global write "UserFunctions.vi" "User Functions"(w720) -> ()
                  }
                  frame Enabled {
                    n429 = property on="User defined functions" class="Str"("Val(Sgnl)"=w721) -> ()  [unwired: 2 in, 2 out]
                  }
                }
                n430 = local write "Loaded Version"(w710) -> ()
                n431 = call "Read AutoPressHWUpdate.vi"("error in (no error)"=w698, "SetListPrefs in"=w702) -> ("AutoPressHWUpdate"=w701:bool)  [unwired: 7 in, 2 out]
                n432 = call "Load_HistoryUpdate.vi"("Limit to 30"=TRUE, "History ref"=w693, "New Path"=w694) -> ()  [unwired: 1 in]
                n433 = local write "DevNums"(w712) -> ()
                n434 = local write "Col array"(w691) -> ()
                n435 = case shown="True" w701 {
                  frame False {
                    n436 = property on="UpdateHWI Button" class="Bool (strict)"("DisabledEnum"=T12."Enabled" ("Disabled")) -> ()  [unwired: 2 in, 2 out]
                  }
                  frame True {
                    n437 = property on="UpdateHWI Button" class="Bool (strict)"("Val(Sgnl)"=TRUE ("Value (Signaling)")) -> ()  [unwired: 2 in, 2 out]
                  }
                }
                n438 = local write "SaveHash"("<Loaded>" ("SaveHash")) -> ()
                n439 = control-ref of="Table History"() -> (w700:refnum<vi>)
                n440 = call "SaveToTblHist.vi"("Table History ref"=w700) -> ()  [unwired: 10 in, 1 out]
              }
              frame True {
                # "user cancelled"
                n441 = call <vilib>:"Clear Errors.vi"("error in (no error)"=w722) -> ()  [unwired: 6 in, 1 out]
              }
            }
            n442 = property on="Loading Text" class="Str"("Visible"=w637) -> ()  [unwired: 2 in, 2 out]
            n443 = local write "Load keep cur. format"(w637) -> ()
          }
        }
        n444 = local write "LoadRecentHash"(w627) -> ()
        n445 = local write "LoadRecentFile"(w627) -> ()
      }
      event "ImportToRepo": Value Change {
        n446 = event-data() -> ()  [unwired: 1 in, 6 out]
        n447 = case shown="True" "ImportToRepo" {
          tunnel: ["Import to Repo..." ("BoolText.Text") "Import to Repo..." ("BoolText.Text")] -> w723
          frame False {
          }
          frame True {
            n448 = local read "Procedure Repository"() -> (w731:path)
            n449 = local read "Git Command"() -> (w732:string)
            n450 = property on="ImportToRepo" class="Bool (strict)"("BoolText.Text"="Importing (Please Wait)..." ("Boolean Text.Text"), "Value"=FALSE ("ImportToRepo")) -> (error out=w729:errorcluster)  [unwired: 2 in, 1 out]
            n451 = control-ref of="This VI"() -> (w727:refnum<vi>)
            n452 = call "GitImportDir.vi"("VI reference (current VI)"=w727, "error in (no error)"=w729, "Save Repo Path"=w731, "Git exec"=w732) -> ()  [unwired: 3 in, 5 out]
          }
        }
        n453 = property on="ImportToRepo" class="Bool (strict)"("BoolText.Text"=w723) -> ()  [unwired: 2 in, 2 out]
      }
      event "Load Recent": Value Change {
        n454 = event-data() -> ("NewVal"=w735:string)  [unwired: 1 in, 2 out]
        n455 = Match True/False String(2:"!@#$%^&*()" ("false string"), 3:"From File: " ("true string"), 4:w735) -> (0:w737:bool, 1:w736:string)
        n456 = case shown="False" w737 {
          tunnel: w735 -> [w742 _]
          tunnel: w736 -> [_ w746]
          frame False {
            # "Grab the hash and have it load via a Val Change event"
            n457 = Match Pattern(string=w742, regular expression="[a-fA-F0-9]+") -> (match substring=w738:string, offset past match=w740:i32)  [unwired: 1 in, 2 out]
            n458 = Greater Or Equal To 0?(x=w740) -> (x >= 0?=w739:bool)
            n459 = case shown="True" w739 {
              tunnel: w738 -> [_ w743]
              frame False {
              }
              frame True {
                n460 = property on="LoadRecentHash" class="Str"("Value"=w743) -> (error out=w745:errorcluster)  [unwired: 2 in, 1 out]
                n461 = property on="Load from Repo" class="Bool (strict)"(error in=w745, "Val(Sgnl)"=TRUE ("Value (Signaling)")) -> ()  [unwired: 1 in, 2 out]
              }
            }
          }
          frame True {
            n462 = property on="LoadRecentFile" class="Str"("Value"=w746) -> (error out=w748:errorcluster)  [unwired: 2 in, 1 out]
            n463 = property on="Load from File" class="Bool (strict)"(error in=w748, "Val(Sgnl)"=TRUE ("Value (Signaling)")) -> ()  [unwired: 1 in, 2 out]
          }
        }
      }
      event "Load Old": Value Change {
        n464 = event-data() -> ("NewVal"=w750:bool)  [unwired: 1 in, 2 out]
        n465 = case shown="True" w750 {
          tunnel: [_ FALSE ("Load from Disk")] -> w749
          frame False {
          }
          frame True {
            n466 = control-ref of="Old Procedure History"() -> (w758:refnum<vi>)
            n467 = local read "Old HWGlobals Path"() -> (w759:path)
            n468 = local read "Old Procedure Path"() -> (w760:path)
            n469 = local read "Version Selection"() -> (w768:T2)
            n470 = control-ref of="Old HWGlobals History"() -> (w756:refnum<vi>)
            n471 = local write "Load Old"(FALSE ("Load from Disk")) -> ()
            n472 = property on="Loading Text" class="Str"("Visible"=TRUE ("Load from Disk")) -> ()  [unwired: 2 in, 2 out]
            n473 = Path To String(path=w759) -> (string=w757:string)
            n474 = Path To String(path=w760) -> (string=w755:string)
            n475 = global read "PrefsGlobal.vi" "SetListPrefs.lvclass"() -> (w763:refnum<class "SetListPrefs.lvclass">)
            n476 = call "convertOldSetlist_toCluster_v5.vi"("HW settings path"=w759, "Load pre 5.6 Globals?"=TRUE, "Procedure path"=w760, "Version Selection"=w768) -> ("Procedure Name"=w771:string, "Save Cluster"=w770:T19, "error out"=w769:errorcluster)  [unwired: 9 in]
            n477 = call "Load_HistoryUpdate.vi"("History ref"=w756, "New Path"=w757) -> ()  [unwired: 2 in]
            n478 = call "Load_HistoryUpdate.vi"("History ref"=w758, "New Path"=w755) -> ()  [unwired: 2 in]
            n479 = local write "Procedure Name"(w771) -> ()
            n480 = control-ref of="Table History"() -> (w761:refnum<vi>)
            n481 = call "Read AutoPressHWUpdate.vi"("SetListPrefs in"=w763) -> ("AutoPressHWUpdate"=w762:bool)  [unwired: 8 in, 2 out]
            n482 = call "SaveToTblHist.vi"("Table History ref"=w761) -> ()  [unwired: 10 in, 1 out]
            n483 = case shown="True" w762 {
              frame False {
                n484 = property on="UpdateHWI Button" class="Bool (strict)"("DisabledEnum"=T12."Enabled" ("Disabled")) -> ()  [unwired: 2 in, 2 out]
              }
              frame True {
                n485 = property on="UpdateHWI Button" class="Bool (strict)"("Val(Sgnl)"=TRUE ("Value (Signaling)")) -> ()  [unwired: 2 in, 2 out]
              }
            }
            n486 = control-ref of="Select Layout"() -> (w774:refnum<vi>)
            n487 = local read "Devices queue"() -> (w752:refnum<queue>)
            n488 = control-ref of="SetList Table"() -> (w765:refnum<vi>)
            n489 = control-ref of="VariableManager"() -> (w753:refnum<vi>)
            n490 = local read "Defer Updates?"() -> (w754:bool)
            n491 = call "LoadedCluster_toSetList_v5.vi"("Devices queue"=w752, "Layout Ref"=w774, "Save Cluster"=w770, "Table Ref in"=w765, "VariableManagerRef"=w753, "error in (no error)"=w769, "Defer Updates? (T)"=w754) -> ("Loaded Version"=w775:string, "DevNums"=w773:i32[], "Col array"=w751:refnum<class "Column.lvclass">[], "User defined functions"=w764:string)  [unwired: 3 in, 2 out]
            n492 = local write "Loaded Version"(w775) -> ()
            n493 = local write "DevNums"(w773) -> ()
            n494 = local write "Col array"(w751) -> ()
            n495 = disable-structure shown="Disabled" {
              disable-tunnel: w764 -> [w779 w780]
              frame Disabled {
                n496 = local write "User defined functions"(w779) -> ()
                n497 = global write "UserFunctions.vi" "User Functions"(w779) -> ()
              }
              frame Enabled {
                n498 = property on="User defined functions" class="Str"("Val(Sgnl)"=w780) -> ()  [unwired: 2 in, 2 out]
              }
            }
          }
        }
        n499 = property on="Loading Text" class="Str"("Visible"=w749) -> ()  [unwired: 2 in, 2 out]
      }
      event "Old Procedure History": Value Change {
        n500 = event-data() -> ("NewVal"=w781:string)  [unwired: 1 in, 2 out]
        n501 = String To Path(string=w781) -> (path=w782:path)
        n502 = local write "Old Procedure Path"(w782) -> ()
      }
      event "Old HWGlobals History": Value Change {
        n503 = event-data() -> ("NewVal"=w783:string)  [unwired: 1 in, 2 out]
        n504 = String To Path(string=w783) -> (path=w784:path)
        n505 = local write "Old HWGlobals Path"(w784) -> ()
      }
      event "Debug: apply appearance": Value Change {
        n506 = event-data() -> ()  [unwired: 1 in, 3 out]
        n507 = control-ref of="Select Layout"() -> (w792:refnum<vi>)
        n508 = control-ref of="SetList Table"() -> (w794:refnum<vi>)
        n509 = local read "Col array"() -> (w785:refnum<class "Column.lvclass">[])
        n510 = local read "Devices queue"() -> (w786:refnum<queue>)
        n511 = local read "Defer Updates?"() -> (w791:bool)
        n512 = call "ModeFromDevices.vi"("error in (no error)"=w789, "Devices queue"=w786) -> ("error out"=w788:errorcluster, "Mode Col"=w787:i32)  [unwired: 8 in]
        n513 = call "ApplyTableAppearance_benchmarking.vi"("Defer Updates? (T)"=w791, "Layout Ring Ref"=w792, "error in (no error)"=w788, "Mode Index"=w787, "Col Array in"=w785, "Table Ref in"=w794) -> ("error out"=w790:errorcluster)  [unwired: 4 in, 1 out]
        n514 = invoke on="Debug: apply appearance" class="Bool (strict)" method="Reinit To Default"(error in=w790) -> (error out=w793:errorcluster)  [unwired: 2 in, 2 out]
      }
      event "UpdateHWI Button": Value Change {
        n515 = event-data() -> ("CtlRef"=w803:refnum<vi>)  [unwired: 1 in, 3 out]
        n516 = local read "Update Event"() -> (w799:refnum<user-event>)
        n517 = property class="Bool (strict)"(reference=w803, "Value"=FALSE) -> ()  [unwired: 1 in, 2 out]
        n518 = Bundle(0, TRUE) -> (w796:cluster{i32, bool})  [unwired: 1 in]
        n519 = property on="SequenceHistory" class="Tbl (strict)"("Value"=string[][] [["", "-1", "Waiting", ""]] ("SequenceHistory"), "Index Values"=T3 {"Row"=0, "Column"=0}) -> (error out=w801:errorcluster)  [unwired: 2 in, 1 out]
        n520 = Generate User Event(user event=w799, event data cluster=w796, error in=w801) -> ()  [unwired: 1 in, 2 out]
      }
      event User Event {
        # "VariableManager Update Events"
        n521 = event-data() -> ("UpdateEvent"=w804:string)  [unwired: 1 in, 4 out]
        n522 = case shown="\"SequenceIndices\", \"UpdateEvent\", \"Variables\", Default" w804 {
          frame "SequenceIndices", "UpdateEvent", "Variables", Default {
            # "Re-enable UpdateHWI button if there is a change to VariableManager definition"
            n523 = global read "PrefsGlobal.vi" "SetListPrefs.lvclass"() -> (w806:refnum<class "SetListPrefs.lvclass">)
            n524 = call "Read AutoPressHWUpdate.vi"("SetListPrefs in"=w806) -> ("AutoPressHWUpdate"=w805:bool)  [unwired: 8 in, 2 out]
            n525 = case shown="True" w805 {
              frame False {
                n526 = property on="UpdateHWI Button" class="Bool (strict)"("DisabledEnum"=T12."Enabled" ("Disabled")) -> ()  [unwired: 2 in, 2 out]
              }
              frame True {
                n527 = property on="UpdateHWI Button" class="Bool (strict)"("Val(Sgnl)"=TRUE ("Value (Signaling)")) -> ()  [unwired: 2 in, 2 out]
              }
            }
          }
          frame "VariableGroups" {
          }
          frame "SequenceValues" {
          }
          frame "LastAcquireValues" {
          }
          frame "StopUI" {
          }
        }
      }
      event "Run Seq Button": Value Change {
        n528 = event-data() -> ("CtlRef"=w814:refnum<vi>, "NewVal"=w810:bool)  [unwired: 1 in, 1 out]
        n529 = local read "CheckSave"() -> (w812:bool)
        n530 = And(x=w812, y=w810) -> (x .and. y?=w811:bool)
        n531 = case shown="True" w811 {
          tunnel: [w815 w816] -> w809
          tunnel: w810 -> [w815 _]
          frame False {
          }
          frame True {
            n532 = local read "Devices queue"() -> (w825:refnum<queue>)
            n533 = local read "DevNums"() -> (w832:i32[])
            n534 = property on="SetList Table" class="Tbl (strict)"() -> (error out=w831:errorcluster, "Value"=w830:string[][])  [unwired: 2 in, 1 out]
            n535 = property on="Select Layout" class="Ring (strict)"() -> ("Value"=w823:i32, "StringsAndValues[]"=w822:T20)  [unwired: 2 in, 2 out]
            n536 = local read "User defined functions"() -> (w821:string)
            n537 = control-ref of="VariableManager"() -> (w827:refnum<vi>)
            n538 = control-ref of="Author"() -> (w843:refnum<vi>)
            n539 = local read "Git Command"() -> (w838:string)
            n540 = local read "Procedure Repository"() -> (w839:path)
            n541 = local read "SaveTitle"() -> (w840:string)
            n542 = local read "Description (Repo Only)"() -> (w841:string)
            n543 = Current VI's Path() -> (path=w829:path)
            n544 = call "SetList SWI to Devices.vi"("error in (no error)"=w831, "SWI table"=w830, "DevNums In"=w832, "Devices queue"=w825) -> ("error out"=w819:errorcluster, "Devices out"=w826:refnum<class "Device.lvclass">[])  [unwired: 5 in, 1 out]
            n545 = call "VMExport.vi"("VariableManagerRef in"=w827) -> ("VariableManagerExportCopy"=w828:refnum<class "VariableManager.lvclass">)  [unwired: 8 in, 2 out]
            n546 = call "GetVersionString.vi"("SetList root path"=w829) -> ("Version String"=w820:string)  [unwired: 2 in]
            n547 = Bundle By Name(cluster=T21 {"Title"="", "Description"="", "Author"=""} ("Current Save Panel Info"), "Title"=w840, "Description"=w841) -> (w837:T21)
            n548 = Bundle By Name(cluster=T19 {"Version"="", "Devices"=[], "Select Layout"=0, "Layout:Strings And Values []"=[], "User defined functions"="", "VariableManager"=refnum}, "Version"=w820, "Devices"=w826, "Select Layout"=w823, "Layout:Strings And Values []"=w822, "User defined functions"=w821, "VariableManager"=w828) -> (w818:T19)
            n549 = local read "LoadHash"() -> (w817:string)
            n550 = call "GitCheckSaveNeeded.vi"("Git exec"=w838, "AuthorRing"=w843, "Save Cluster"=w818, "Loaded Hash"=w817, "Save Repo Path"=w839, "error in (no error)"=w819, "Current Save Panel Info"=w837) -> ("Saved"=w836:bool, "Git exec out"=w835:string, "Continue"=w816:bool, "Saved Hash"=w833:string, "Save Repo Path Out"=w834:path)  [unwired: 3 in, 1 out]
            n551 = case shown="True" w836 {
              tunnel: w835 -> [_ w859]
              tunnel: w834 -> [_ w860]
              tunnel: w833 -> [_ w846]
              tunnel: w820 -> [_ w853]
              frame False {
              }
              frame True {
                n552 = local write "Loaded Version"(w853) -> ()
                n553 = call "GitHashToInfo.vi"("Directory"=w860, "Hash"=w846, "Git exec"=w859) -> ("error out"=w852:errorcluster, "Directory out"=w851:path, "Commit Info"=w855:T22, "Git exec out"=w850:string, "Description"=w847:string)  [unwired: 4 in]
                n554 = local write "SaveHash"(w846) -> ()
                n555 = local write "LoadHash"(w846) -> ()
                n556 = call "GitGetFullHash.vi"("error in (no error)"=w852, "Directory"=w851, "Partial Hash"=w846, "Git exec"=w850) -> ("Full Hash"=w845:string)  [unwired: 4 in, 3 out]
                n557 = local write "Loaded Description"(w847) -> ()
                n558 = call "CommitCluster-to-MenuString.vi"("Commit"=w855) -> ("Menu String"=w858:string)  [unwired: 2 in]
                n559 = local write "Load Long Hash/Filename"(w845) -> ()
                n560 = control-ref of="Load Recent"() -> (w857:refnum<vi>)
                n561 = Unbundle By Name(w855) -> ("Name"=w854:string)
                n562 = Format Into String(format string="Based on %s (%s)\n%s", w846, w845, w847) -> (resulting string=w848:string)  [unwired: 2 in, 1 out]
                n563 = local write "Description (Repo Only)"(w848) -> ()
                n564 = call "Load_HistoryUpdate.vi"("Limit to 30"=TRUE, "History ref"=w857, "New Path"=w858) -> ()  [unwired: 1 in]
                n565 = local write "SaveTitle"(w854) -> ()
                n566 = local write "Procedure Name"(w854) -> ()
              }
            }
            n567 = case shown="False" w816 {
              selector: w816 -> [w844 _]
              frame False {
                n568 = local write "Run Seq Button"(w844) -> ()
              }
              frame True {
              }
            }
          }
        }
        n569 = case shown="True" w809 {
          tunnel: w814 -> [_ w865]
          tunnel: [_ w864] -> w813
          frame False {
          }
          frame True {
            n570 = control-ref of="VariableManager"() -> (w861:refnum<vi>)
            n571 = call "GetTotalSequenceSteps.vi"("VariableManagerRef in"=w861) -> ("error out"=w866:errorcluster, "TotalSequenceSteps"=w863:i32, "VariableManagerRef out"=w862:refnum<vi>)  [unwired: 8 in]
            n572 = case shown="No Error" w866 {
              selector: w866 -> [w869 w1068]
              tunnel: w865 -> [_ w1070]
              tunnel: [_ w1068] -> w864
              tunnel: w863 -> [w877 _]
              tunnel: w862 -> [w870 _]
              frame No Error {
                w873 = T12."Disabled" ("Disabled")
                n573 = for {
                  N: w877 -> [_]
                  tunnel: [w1063] -> w876 mode=indexing
                  i -> [w1067]
                  n574 = Number To Decimal String(number=w1067) -> (decimal integer string=w1066:string)  [unwired: 1 in]
                  n575 = Build Array("" ("element"), w1066, "Waiting", "") -> (w1063:string[])
                }
                n576 = property on="Run Button" class="Bool (strict)"("DisabledEnum"=w873) -> ()  [unwired: 2 in, 2 out]
                n577 = property on="Run Seq Button" class="Bool (strict)"("DisabledEnum"=w873) -> ()  [unwired: 2 in, 2 out]
                n578 = property on="RandomSequence" class="Bool (strict)"("DisabledEnum"=w873) -> ("Value"=w872:bool)  [unwired: 2 in, 2 out]
                n579 = property on="StopExperiment" class="Bool (strict)"("DisabledEnum"=T12."Enabled" ("Disabled")) -> ()  [unwired: 2 in, 2 out]
                n580 = case shown="True" w872 {
                  tunnel: w877 -> [_ w884]
                  tunnel: w876 -> [w881 w885]
                  tunnel: [w881 w883] -> w868
                  tunnel: w870 -> [_ w888]
                  tunnel: w869 -> [_ w887]
                  frame False {
                  }
                  frame True {
                    n581 = call "VMExport.vi"("error in (no error)"=w887, "VariableManagerRef in"=w888) -> ("error out"=w886:errorcluster, "VariableManagerExportCopy"=w882:refnum<class "VariableManager.lvclass">)  [unwired: 7 in, 1 out]
                    n582 = case shown="No Error" w886 {
                      selector: w886 -> [w891 _]
                      tunnel: w885 -> [w895 w1061]
                      tunnel: w884 -> [w897 _]
                      tunnel: [w896 w1061] -> w883
                      tunnel: w882 -> [w889 _]
                      frame No Error {
                        n583 = property class="VariableManager.lvclass"(reference=w889, error in=w891) -> ("Accessors:SequenceIndices"=w890:refnum<class "SequenceIndex.lvclass">[])  [unwired: 2 out]
                        n584 = To Unsigned Long Integer(number=w897) -> (unsigned 32bit integer=w894:u32)
                        n585 = Reverse 1D Array(array=w890) -> (reversed array=w893:refnum<class "SequenceIndex.lvclass">[])
                        n586 = Array Size(array=w890) -> (size(s)=w898:i32)
                        n587 = for {
                          N: w898 -> [w907]
                          tunnel: w893 -> [w917] mode=indexing
                          shift-right: [w914] -> w896
                          shift-left: w895 -> [w915]
                          shift-right: [w908] -> _
                          shift-left: w894 -> [w911]
                          tunnel: w894 -> [w912]
                          tunnel: w893 -> [w904]
                          shift-right: [w902] -> _
                          shift-left: u32 1 ("Accessors:Steps") -> [w901]
                          i -> [w903]
                          n588 = Decrement(x=w907) -> (x-1=w906:i32)
                          n589 = property class="SequenceIndex.lvclass"(reference=w917) -> ("Accessors:Steps"=w900:u32, "Accessors:Keep Linear on Random"=w916:bool, "Accessors:Block Randomize"=w909:bool)  [unwired: 1 in, 2 out]
                          n590 = Quotient & Remainder(x=w912, y=w911) -> (floor(x/y)=w910:u32)  [unwired: 1 out]
                          n591 = Multiply(x=w900, y=w901) -> (x*y=w899:u32)
                          n592 = Quotient & Remainder(x=w911, y=w899) -> (floor(x/y)=w913:u32)  [unwired: 1 out]
                          n593 = Less?(x=w903, y=w906) -> (x < y?=w905:bool)
                          n594 = for {
                            N: w910 -> [_]
                            tunnel: w916 -> [w930]
                            tunnel: w899 -> [w929]
                            tunnel: w913 -> [w928]
                            shift-right: [w925] -> w914
                            shift-left: w915 -> [w927]
                            tunnel: w911 -> [w919]
                            tunnel: w909 -> [w924]
                            tunnel: [w923] -> w908
                            tunnel: w905 -> [w922]
                            tunnel: w904 -> [w921]
                            tunnel: w903 -> [w920]
                            tunnel: [w918] -> w902
                            i -> [w926]
                            n595 = case shown="False" w924 {
                              tunnel: w930 -> [w935 w1039]
                              tunnel: w929 -> [w943 w1038]
                              tunnel: w928 -> [w942 w1029]
                              tunnel: w927 -> [w941 w1037]
                              tunnel: w926 -> [w940 w1035]
                              tunnel: w919 -> [w938 w1034]
                              tunnel: [w939 w1031] -> w925
                              tunnel: [w937 w1029] -> w923
                              tunnel: w922 -> [w936 _]
                              tunnel: w921 -> [w934 _]
                              tunnel: w920 -> [w933 _]
                              tunnel: w919 -> [w932 _]
                              tunnel: [w931 u32 1 ("Accessors:Steps")] -> w918
                              frame False {
                                n596 = Multiply(x=w938, y=w940) -> (x*y=w944:u32)
                                n597 = Delete From Array(array=w941, length=w938, index (row)=w944) -> (deleted portion=w947:string[][], array with subset deleted=w946:string[][])  [unwired: 1 in]
                                n598 = case shown="True" w936 {
                                tunnel: [w951 w984] -> w945
                                tunnel: w943 -> [w953 w979]
                                tunnel: w942 -> [w949 w983]
                                tunnel: w947 -> [w952 w985]
                                tunnel: [w949 w982] -> w937
                                tunnel: w935 -> [w950 w986]
                                tunnel: w934 -> [_ w980]
                                tunnel: w933 -> [_ w981]
                                tunnel: w932 -> [_ w978]
                                tunnel: [w948 w977] -> w931
                                frame False {
                                n599 = case shown="False" w950 {
                                tunnel: w953 -> [w959 _]
                                tunnel: w952 -> [w958 w976]
                                tunnel: [w956 w976] -> w951
                                tunnel: w949 -> [w955 _]
                                tunnel: [u32 1 ("Accessors:Steps") u32 1 ("Accessors:Steps")] -> w948
                                frame False {
                                n600 = for {
                                N: w959 -> [w974]
                                shift-right: [w972] -> _
                                shift-left: w958 -> [w965]
                                tunnel: w955 -> [w960]
                                shift-right: [w964] -> w956
                                shift-left: string[][] [] ("deleted portion") -> [w962]
                                i -> [w963]
                                n601 = Random Number (0-1)() -> (number: 0 to 1=w970:dbl)
                                n602 = Subtract(x=w974, y=w963) -> (x-y=w973:i32)
                                n603 = Multiply(x=w960, y=w963) -> (x*y=w961:u32)
                                n604 = Multiply(x=w973, y=w970) -> (x*y=w971:dbl)
                                n605 = Round Toward -Infinity(1:w971) -> (0:w969:dbl)
                                n606 = To Unsigned Long Integer(number=w969) -> (unsigned 32bit integer=w968:u32)
                                n607 = Multiply(x=w968, y=w960) -> (x*y=w967:u32)
                                n608 = Delete From Array(array=w965, length=w960, index (row)=w967) -> (deleted portion=w966:string[][], array with subset deleted=w972:string[][])  [unwired: 1 in]
                                n609 = Insert Into Array(array=w962, index (row)=w961, new element=w966) -> (w964:string[][])  [unwired: 1 in]
                                }
                                }
                                frame True {
                                }
                                }
                                }
                                frame True {
                                n610 = case shown="False" w986 {
                                tunnel: w985 -> [w993 w1027]
                                tunnel: [w992 w1027] -> w984
                                tunnel: w983 -> [w990 w1026]
                                tunnel: [w989 w1026] -> w982
                                tunnel: w981 -> [w999 _]
                                tunnel: w980 -> [w998 _]
                                tunnel: w979 -> [w991 _]
                                tunnel: w978 -> [w988 _]
                                tunnel: [w987 u32 1 ("Accessors:Steps")] -> w977
                                frame False {
                                n611 = Increment(x=w999) -> (x+1=w1000:i32)
                                n612 = Index Array(array=w998, index=w1000) -> (element=w997:refnum<class "SequenceIndex.lvclass">)
                                n613 = property class="SequenceIndex.lvclass" props=["Accessors:Steps", "Accessors:Keep Linear on Random", "Accessors:Block Randomize"](reference=w997) -> ("Accessors:Keep Linear on Random"=w995:bool, "Accessors:Block Randomize"=w996:bool)  [unwired: 1 in, 3 out]
                                n614 = Or(x=w995, y=w996) -> (x .or. y?=w994:bool)
                                n615 = case shown="True" w994 {
                                tunnel: w993 -> [w1003 w1009]
                                tunnel: [w1003 w1008] -> w992
                                tunnel: w991 -> [w1001 w1006]
                                tunnel: w990 -> [_ w1005]
                                tunnel: [w1002 w1005] -> w989
                                tunnel: w988 -> [w1002 _]
                                tunnel: [w1001 u32 1 ("Accessors:Steps")] -> w987
                                frame False {
                                }
                                frame True {
                                n616 = for {
                                N: w1006 -> [w1024]
                                shift-right: [w1022] -> _
                                shift-left: w1009 -> [w1015]
                                tunnel: w1005 -> [w1010]
                                shift-right: [w1014] -> w1008
                                shift-left: string[][] [] ("deleted portion") -> [w1012]
                                i -> [w1013]
                                n617 = Random Number (0-1)() -> (number: 0 to 1=w1020:dbl)
                                n618 = Subtract(x=w1024, y=w1013) -> (x-y=w1023:i32)
                                n619 = Multiply(x=w1010, y=w1013) -> (x*y=w1011:u32)
                                n620 = Multiply(x=w1023, y=w1020) -> (x*y=w1021:dbl)
                                n621 = Round Toward -Infinity(1:w1021) -> (0:w1019:dbl)
                                n622 = To Unsigned Long Integer(number=w1019) -> (unsigned 32bit integer=w1018:u32)
                                n623 = Multiply(x=w1018, y=w1010) -> (x*y=w1017:u32)
                                n624 = Delete From Array(array=w1015, length=w1010, index (row)=w1017) -> (deleted portion=w1016:string[][], array with subset deleted=w1022:string[][])  [unwired: 1 in]
                                n625 = Insert Into Array(array=w1012, index (row)=w1011, new element=w1016) -> (w1014:string[][])  [unwired: 1 in]
                                }
                                }
                                }
                                }
                                frame True {
                                }
                                }
                                }
                                }
                                n626 = Insert Into Array(array=w946, index (row)=w944, new element=w945) -> (w939:string[][])  [unwired: 1 in]
                              }
                              frame True {
                                n627 = Multiply(x=w1034, y=w1035) -> (x*y=w1030:u32)
                                n628 = Delete From Array(array=w1037, length=w1034, index (row)=w1030) -> (deleted portion=w1036:string[][], array with subset deleted=w1033:string[][])  [unwired: 1 in]
                                n629 = case shown="False" w1039 {
                                tunnel: [w1040 w1060] -> w1032
                                tunnel: w1038 -> [w1044 _]
                                tunnel: w1029 -> [w1043 _]
                                tunnel: w1036 -> [w1042 w1060]
                                frame False {
                                n630 = for {
                                N: w1044 -> [w1059]
                                shift-right: [w1057] -> _
                                shift-left: w1042 -> [w1050]
                                tunnel: w1043 -> [w1048]
                                shift-right: [w1049] -> w1040
                                shift-left: string[][] [] ("deleted portion") -> [w1046]
                                i -> [w1047]
                                n631 = Random Number (0-1)() -> (number: 0 to 1=w1055:dbl)
                                n632 = Subtract(x=w1059, y=w1047) -> (x-y=w1058:i32)
                                n633 = Multiply(x=w1048, y=w1047) -> (x*y=w1045:u32)
                                n634 = Multiply(x=w1058, y=w1055) -> (x*y=w1056:dbl)
                                n635 = Round Toward -Infinity(1:w1056) -> (0:w1054:dbl)
                                n636 = To Unsigned Long Integer(number=w1054) -> (unsigned 32bit integer=w1053:u32)
                                n637 = Multiply(x=w1053, y=w1048) -> (x*y=w1052:u32)
                                n638 = Delete From Array(array=w1050, length=w1048, index (row)=w1052) -> (deleted portion=w1051:string[][], array with subset deleted=w1057:string[][])  [unwired: 1 in]
                                n639 = Insert Into Array(array=w1046, index (row)=w1045, new element=w1051) -> (w1049:string[][])  [unwired: 1 in]
                                }
                                }
                                frame True {
                                }
                                }
                                n640 = Insert Into Array(array=w1033, index (row)=w1030, new element=w1032) -> (w1031:string[][])  [unwired: 1 in]
                              }
                            }
                          }
                        }
                      }
                      frame Error {
                      }
                    }
                  }
                }
                n641 = local read "Seq. Event"() -> (w867:refnum<user-event>)
                n642 = property on="SequenceHistory" class="Tbl (strict)"("Value"=w868, "Index Values"=T3 {"Row"=0, "Column"=0}) -> (error out=w875:errorcluster)  [unwired: 2 in, 1 out]
                n643 = Bundle("milliseconds to wait"=u32 0, FALSE) -> (w879:cluster{"milliseconds to wait":u32, bool})  [unwired: 1 in]
                n644 = Generate User Event(user event=w867, event data cluster=w879, error in=w875) -> ()  [unwired: 1 in, 2 out]
              }
              frame Error {
                n645 = property class="Bool (strict)"(reference=w1070, "Value"=FALSE) -> ()  [unwired: 1 in, 2 out]
              }
            }
          }
        }
      }
      event "Run Button": Value Change {
        n646 = event-data() -> ("NewVal"=w1073:bool)  [unwired: 1 in, 2 out]
        n647 = local read "CheckSave"() -> (w1071:bool)
        n648 = And(x=w1071, y=w1073) -> (x .and. y?=w1072:bool)
        n649 = case shown="False" w1072 {
          tunnel: [w1075 w1076] -> w1074
          tunnel: w1073 -> [w1075 _]
          frame False {
          }
          frame True {
            n650 = local read "Devices queue"() -> (w1085:refnum<queue>)
            n651 = local read "DevNums"() -> (w1092:i32[])
            n652 = property on="SetList Table" class="Tbl (strict)"() -> (error out=w1091:errorcluster, "Value"=w1090:string[][])  [unwired: 2 in, 1 out]
            n653 = property on="Select Layout" class="Ring (strict)"() -> ("Value"=w1083:i32, "StringsAndValues[]"=w1082:T20)  [unwired: 2 in, 2 out]
            n654 = local read "User defined functions"() -> (w1081:string)
            n655 = control-ref of="VariableManager"() -> (w1087:refnum<vi>)
            n656 = control-ref of="Author"() -> (w1103:refnum<vi>)
            n657 = local read "Git Command"() -> (w1098:string)
            n658 = local read "Procedure Repository"() -> (w1099:path)
            n659 = local read "SaveTitle"() -> (w1100:string)
            n660 = local read "Description (Repo Only)"() -> (w1101:string)
            n661 = Current VI's Path() -> (path=w1089:path)
            n662 = call "SetList SWI to Devices.vi"("error in (no error)"=w1091, "SWI table"=w1090, "DevNums In"=w1092, "Devices queue"=w1085) -> ("error out"=w1079:errorcluster, "Devices out"=w1086:refnum<class "Device.lvclass">[])  [unwired: 5 in, 1 out]
            n663 = call "VMExport.vi"("VariableManagerRef in"=w1087) -> ("VariableManagerExportCopy"=w1088:refnum<class "VariableManager.lvclass">)  [unwired: 8 in, 2 out]
            n664 = call "GetVersionString.vi"("SetList root path"=w1089) -> ("Version String"=w1080:string)  [unwired: 2 in]
            n665 = Bundle By Name(cluster=T21 {"Title"="", "Description"="", "Author"=""} ("Current Save Panel Info"), "Title"=w1100, "Description"=w1101) -> (w1097:T21)
            n666 = Bundle By Name(cluster=T19 {"Version"="", "Devices"=[], "Select Layout"=0, "Layout:Strings And Values []"=[], "User defined functions"="", "VariableManager"=refnum}, "Version"=w1080, "Devices"=w1086, "Select Layout"=w1083, "Layout:Strings And Values []"=w1082, "User defined functions"=w1081, "VariableManager"=w1088) -> (w1078:T19)
            n667 = local read "LoadHash"() -> (w1077:string)
            n668 = call "GitCheckSaveNeeded.vi"("Git exec"=w1098, "AuthorRing"=w1103, "Save Cluster"=w1078, "Loaded Hash"=w1077, "Save Repo Path"=w1099, "error in (no error)"=w1079, "Current Save Panel Info"=w1097) -> ("Saved"=w1096:bool, "Git exec out"=w1095:string, "Continue"=w1076:bool, "Saved Hash"=w1093:string, "Save Repo Path Out"=w1094:path)  [unwired: 3 in, 1 out]
            n669 = case shown="True" w1096 {
              tunnel: w1095 -> [_ w1119]
              tunnel: w1094 -> [_ w1120]
              tunnel: w1093 -> [_ w1105]
              tunnel: w1080 -> [_ w1113]
              frame False {
              }
              frame True {
                n670 = local write "Loaded Version"(w1113) -> ()
                n671 = call "GitHashToInfo.vi"("Directory"=w1120, "Hash"=w1105, "Git exec"=w1119) -> ("error out"=w1112:errorcluster, "Directory out"=w1111:path, "Commit Info"=w1115:T22, "Git exec out"=w1110:string, "Description"=w1107:string)  [unwired: 4 in]
                n672 = local write "SaveHash"(w1105) -> ()
                n673 = local write "LoadHash"(w1105) -> ()
                n674 = local write "Loaded Description"(w1107) -> ()
                n675 = call "GitGetFullHash.vi"("error in (no error)"=w1112, "Directory"=w1111, "Partial Hash"=w1105, "Git exec"=w1110) -> ("Full Hash"=w1106:string)  [unwired: 4 in, 3 out]
                n676 = call "CommitCluster-to-MenuString.vi"("Commit"=w1115) -> ("Menu String"=w1118:string)  [unwired: 2 in]
                n677 = local write "Load Long Hash/Filename"(w1106) -> ()
                n678 = control-ref of="Load Recent"() -> (w1117:refnum<vi>)
                n679 = Unbundle By Name(w1115) -> ("Name"=w1114:string)
                n680 = Format Into String(format string="Based on %s (%s)\n%s", w1105, w1106, w1107) -> (resulting string=w1108:string)  [unwired: 2 in, 1 out]
                n681 = local write "Description (Repo Only)"(w1108) -> ()
                n682 = call "Load_HistoryUpdate.vi"("Limit to 30"=TRUE, "History ref"=w1117, "New Path"=w1118) -> ()  [unwired: 1 in]
                n683 = local write "SaveTitle"(w1114) -> ()
                n684 = local write "Procedure Name"(w1114) -> ()
              }
            }
            n685 = case shown="False" w1076 {
              selector: w1076 -> [w1104 _]
              frame False {
                n686 = local write "Run Button"(w1104) -> ()
              }
              frame True {
              }
            }
          }
        }
        n687 = case shown="True" w1074 {
          frame False {
          }
          frame True {
            w1128 = T12."Disabled" ("Disabled")
            n688 = local read "Update Event"() -> (w1126:refnum<user-event>)
            n689 = Bundle("dimension size"=0, TRUE) -> (w1121:cluster{"dimension size":i32, bool})  [unwired: 1 in]
            n690 = property on="SequenceHistory" class="Tbl (strict)"("Value"=string[][] [["", "-1", "Waiting", ""]] ("SequenceHistory"), "Index Values"=T3 {"Row"=0, "Column"=0}) -> (error out=w1125:errorcluster)  [unwired: 2 in, 1 out]
            n691 = Generate User Event(user event=w1126, event data cluster=w1121, error in=w1125) -> (error out=w1124:errorcluster)  [unwired: 1 in, 1 out]
            n692 = local read "Seq. Event"() -> (w1133:refnum<user-event>)
            n693 = Bundle("dimension size"=0, FALSE) -> (w1134:cluster{"dimension size":i32, bool})  [unwired: 1 in]
            n694 = Generate User Event(user event=w1133, event data cluster=w1134, error in=w1124) -> ()  [unwired: 1 in, 2 out]
            n695 = property on="Run Button" class="Bool (strict)"("DisabledEnum"=w1128) -> ()  [unwired: 2 in, 2 out]
            n696 = property on="Run Seq Button" class="Bool (strict)"("DisabledEnum"=w1128) -> ()  [unwired: 2 in, 2 out]
            n697 = property on="RandomSequence" class="Bool (strict)"("DisabledEnum"=w1128) -> ()  [unwired: 2 in, 2 out]
            n698 = property on="StopExperiment" class="Bool (strict)"("DisabledEnum"=T12."Enabled" ("Disabled")) -> ()  [unwired: 2 in, 2 out]
          }
        }
      }
      event "SetSharedVarIP": Value Change {
        n699 = event-data() -> ("NewVal"=w1135:bool)  [unwired: 1 in]
        n700 = case shown="True" w1135 {
          frame False {
          }
          frame True {
            n701 = global read "PrefsGlobal.vi" "SetListPrefs.lvclass"() -> (w1138:refnum<class "SetListPrefs.lvclass">)
            n702 = call "DeploySharedVariables.vi"("Target IPAddress"="Shared Variable Deploy IP") -> ("error out"=w1139:errorcluster)
            n703 = case shown="No Error" w1139 {
              selector: w1139 -> [w1140 w1149]
              tunnel: w1138 -> [w1141 w1151]
              tunnel: [w1143 w1150] -> w1137
              tunnel: "Shared Variable Deploy IP" -> [w1142 w1146]
              frame No Error {
                n704 = call "Write SharedVariableDeployIP.vi"("error in (no error)"=w1140, "SharedVariableDeployIP"=w1142, "SetListPrefs in"=w1141) -> ("SetListPrefs out"=w1143:refnum<class "SetListPrefs.lvclass">)  [unwired: 7 in, 1 out]
              }
              frame Error {
                # "Reinstate Old IP"
                n705 = call <vilib>:"Clear Errors.vi"("error in (no error)"=w1149) -> ("error out"=w1148:errorcluster)  [unwired: 6 in]
                n706 = call "Read SharedVariableDeployIP.vi"("error in (no error)"=w1148, "SetListPrefs in"=w1151) -> ("SharedVariableDeployIP"=w1144:string, "SetListPrefs out"=w1150:refnum<class "SetListPrefs.lvclass">)  [unwired: 7 in, 1 out]
                n707 = local write "Shared Variable Deploy IP"(w1144) -> ()
                n708 = Format Into String(format string="Could not deploy to IP\\n%s\\nReturning to prior IP\\n(%s)", w1146, w1144) -> (resulting string=w1147:string)  [unwired: 2 in, 1 out]
                n709 = One Button Dialog(message=w1147) -> ()  [unwired: 1 in, 1 out]
              }
            }
            n710 = global write "PrefsGlobal.vi" "SetListPrefs.lvclass"(w1137) -> ()
          }
        }
      }
      event "Procedure Repository": Value Change {
        n711 = event-data() -> ("NewVal"=w1152:path, "OldVal"=w1157:path)  [unwired: 1 in]
        n712 = global read "PrefsGlobal.vi" "SetListPrefs.lvclass"() -> (w1153:refnum<class "SetListPrefs.lvclass">)
        n713 = call "Read GitCmd.vi"("SetListPrefs in"=w1153) -> ("error out"=w1155:errorcluster, "GitCmd"=w1156:string, "SetListPrefs out"=w1154:refnum<class "SetListPrefs.lvclass">)  [unwired: 8 in]
        n714 = call "GitCheckRepo.vi"("error in (no error)"=w1155, "Directory"=w1152, "Git exec"=w1156) -> ("error out"=w1160:errorcluster, "Directory out"=w1159:path, "ProcedureRepo?"=w1161:bool, "Git exec out"=w1158:string)  [unwired: 5 in]
        n715 = case shown="True" w1161 {
          tunnel: w1160 -> [w1169 w1185]
          tunnel: w1159 -> [w1170 w1184]
          tunnel: w1158 -> [w1171 w1183]
          tunnel: w1157 -> [_ w1178]
          tunnel: w1154 -> [w1168 w1177]
          frame False {
            # "Not a Repo, Init!"
            n716 = call "GitInit.vi"("error in (no error)"=w1169, "Directory"=w1170, "Git exec"=w1171) -> ("error out"=w1174:errorcluster, "Directory out"=w1172:path, "Git exec out"=w1173:string)  [unwired: 5 in, 1 out]
            n717 = call "GitSetup.vi"("error in (no error)"=w1174, "Directory"=w1172, "Git exec"=w1173) -> ("error out"=w1166:errorcluster, "Directory out"=w1164:path, "Git exec out"=w1162:string)  [unwired: 5 in, 1 out]
            n718 = call "GitUpdateGitignore.vi"("error in (no error)"=w1166, "Directory in"=w1164, "Git exec in"=w1162) -> ("error out"=w1165:errorcluster, "Directory out"=w1163:path)  [unwired: 6 in, 1 out]
            n719 = call "Write ProcRepo.vi"("error in (no error)"=w1165, "ProcRepo"=w1163, "SetListPrefs in"=w1168) -> ("error out"=w1176:errorcluster, "SetListPrefs out"=w1175:refnum<class "SetListPrefs.lvclass">)  [unwired: 7 in]
            n720 = call "SaveOnly.vi"("error in (no error)"=w1176, "Preferences in"=w1175) -> ("Preferences out"=w1167:refnum<class "SetListPrefs.lvclass">)  [unwired: 7 in, 2 out]
            n721 = global write "PrefsGlobal.vi" "SetListPrefs.lvclass"(w1167) -> ()
          }
          frame True {
            # "Already a Repo, check if a ProcRepo"
            n722 = call "GitCheckProcRepo.vi"("error in (no error)"=w1185, "Directory"=w1184, "Git exec"=w1183) -> ("error out"=w1181:errorcluster, "Directory out"=w1180:path, "ProcedureRepo?"=w1179:bool, "Git exec out"=w1182:string)  [unwired: 5 in]
            n723 = case shown="True" w1179 {
              tunnel: w1182 -> [_ w1192]
              tunnel: w1181 -> [w1190 w1196]
              tunnel: w1180 -> [w1189 w1193]
              tunnel: w1178 -> [w1191 _]
              tunnel: w1177 -> [_ w1198]
              frame False {
                # "Other Repo, ABORT"
                n724 = property on="Procedure Repository" class="Path"(error in=w1190, "Value"=w1191) -> ()  [unwired: 1 in, 2 out]
                n725 = Path To String(path=w1189) -> (string=w1188:string)
                n726 = Concatenate Strings(w1188, " is not a valid Procedure Repo Location.\nPlease choose a different one." ("string")) -> (w1187:string)
                n727 = One Button Dialog(message=w1187) -> ()  [unwired: 1 in, 1 out]
              }
              frame True {
                # "ProcRepo, we're good"
                n728 = call "GitUpdateGitignore.vi"("error in (no error)"=w1196, "Directory in"=w1193, "Git exec in"=w1192) -> ("error out"=w1195:errorcluster, "Directory out"=w1194:path)  [unwired: 6 in, 1 out]
                n729 = call "Write ProcRepo.vi"("error in (no error)"=w1195, "ProcRepo"=w1194, "SetListPrefs in"=w1198) -> ("error out"=w1200:errorcluster, "SetListPrefs out"=w1199:refnum<class "SetListPrefs.lvclass">)  [unwired: 7 in]
                n730 = call "SaveOnly.vi"("error in (no error)"=w1200, "Preferences in"=w1199) -> ("Preferences out"=w1197:refnum<class "SetListPrefs.lvclass">)  [unwired: 7 in, 2 out]
                n731 = global write "PrefsGlobal.vi" "SetListPrefs.lvclass"(w1197) -> ()
              }
            }
          }
        }
      }
      event "Git Authors": Value Change {
        n732 = event-data() -> ()  [unwired: 1 in, 1 out]
        n733 = for {
          tunnel: "Git Authors" -> [w1223] mode=indexing
          tunnel: [w1219] -> w1209 mode=indexing if=w1210
          n734 = Index Array(array=w1223, index #1=0 ("index"), index #2=1 ("index")) -> (element #1=w1213:string, element #2=w1218:string)
          n735 = call <vilib>:"Trim Whitespace.vi"("string"=w1218) -> ("trimmed string"=w1216:string)  [unwired: 1 in]
          n736 = Empty String/Path?(string/path=w1216) -> (empty?=w1217:bool)
          n737 = call <vilib>:"Trim Whitespace.vi"("string"=w1213) -> ("trimmed string"=w1212:string)  [unwired: 1 in]
          n738 = Empty String/Path?(string/path=w1212) -> (empty?=w1211:bool)
          n739 = Select(t="JQIbot@users.noreply.github.com", s=w1217, f=w1216) -> (s? t:f=w1215:string)
          n740 = Not(x=w1211) -> (.not. x?=w1210:bool)
          n741 = Format Into String(format string="%s <%s>", w1212, w1215) -> (resulting string=w1219:string)  [unwired: 2 in, 1 out]
        }
        n742 = global read "PrefsGlobal.vi" "SetListPrefs.lvclass"() -> (w1205:refnum<class "SetListPrefs.lvclass">)
        n743 = Array Subset(array="Git Authors", index (col)=0 ("index"), length (col)=2 ("length")) -> (w1204:string[][])  [unwired: 2 in]
        n744 = call "Write GitAuths.vi"("GitAuths"=w1204, "SetListPrefs in"=w1205) -> ("SetListPrefs out"=w1206:refnum<class "SetListPrefs.lvclass">)  [unwired: 8 in, 1 out]
        n745 = global write "PrefsGlobal.vi" "SetListPrefs.lvclass"(w1206) -> ()
        n746 = Build Array (concatenate)("SetList Program <JQIbot@users.noreply.github.com>", w1209) -> (w1207:string[])
        n747 = property on="Author" class="Ring (strict)"("Strings []"=w1207) -> ()  [unwired: 2 in, 2 out]
      }
      event "Resume Button": Value Change {
        w1228 = T12."Disabled" ("Disabled")
        n748 = event-data() -> ("CtlRef"=w1231:refnum<vi>)  [unwired: 1 in]
        n749 = property class="Bool (strict)"(reference=w1231, "Value"=FALSE) -> ()  [unwired: 1 in, 2 out]
        n750 = property on="Run Button" class="Bool (strict)"("DisabledEnum"=w1228) -> ()  [unwired: 2 in, 2 out]
        n751 = property on="Run Seq Button" class="Bool (strict)"("DisabledEnum"=w1228, "Value"=TRUE) -> (error out=w1225:errorcluster)  [unwired: 2 in, 1 out]
        n752 = property on="RandomSequence" class="Bool (strict)"("DisabledEnum"=w1228) -> ()  [unwired: 2 in, 2 out]
        n753 = property on="StopExperiment" class="Bool (strict)"("DisabledEnum"=T12."Enabled" ("Disabled"), "Value"=FALSE ("StopExperiment")) -> (error out=w1226:errorcluster)  [unwired: 2 in, 1 out]
        n754 = local read "Seq. Event"() -> (w1233:refnum<user-event>)
        n755 = Bundle("dimension size"=0, FALSE) -> (w1232:cluster{"dimension size":i32, bool})  [unwired: 1 in]
        n756 = Merge Errors(w1225, w1226) -> (w1224:errorcluster)
        n757 = Generate User Event(user event=w1233, event data cluster=w1232, error in=w1224) -> ()  [unwired: 1 in, 2 out]
      }
      event "SequenceHistory": Mouse Down? {
        # "Mulligan functionality"
        n758 = event-data() -> ("CtlRef"=w1241:refnum<vi>, "Coords"=w1240:T17)  [unwired: 1 in]
        n759 = invoke class="Tbl (strict)" method="Point To Row Column"(reference=w1241, "Point"=w1240) -> (reference out=w1238:refnum<vi>, "InBounds"=w1237:bool, "CellPosition"=w1239:T4)  [unwired: 4 in, 3 out]
        n760 = case shown="True" w1237 {
          tunnel: w1239 -> [_ w1248]
          tunnel: w1238 -> [_ w1247]
          frame False {
          }
          frame True {
            # "If click in table"
            n761 = property class="Tbl (strict)"(reference=w1247) -> (reference out=w1244:refnum<vi>, "Value"=w1243:string[][])  [unwired: 1 in, 1 out]
            n762 = Unbundle(w1248) -> ("Row"=w1242:i32)  [unwired: 1 out]
            n763 = Index Array(array=w1243, index (row)=w1242, index (col)=2 ("disabled index (col)")) -> (element=w1245:string)
            n764 = case shown="\"Waiting\"" w1245 {
              tunnel: w1244 -> [_ w1250 w1256]
              tunnel: w1243 -> [_ w1254 w1260]
              tunnel: w1242 -> [_ w1253 w1259]
              frame Default {
              }
              frame "Waiting" {
                n765 = Replace Array Subset(array=w1254, new element="Complete", index (row)=w1253, index (col)=2 ("disabled index (col)")) -> (w1249:string[][])
                n766 = property class="Tbl (strict)"(reference=w1250, "Value"=w1249) -> ()  [unwired: 1 in, 2 out]
              }
              frame "Complete", "HW Error" {
                n767 = Replace Array Subset(array=w1260, new element="Waiting", index (row)=w1259, index (col)=2 ("disabled index (col)")) -> (w1255:string[][])
                n768 = property class="Tbl (strict)"(reference=w1256, "Value"=w1255) -> ()  [unwired: 1 in, 2 out]
              }
            }
          }
        }
        n769 = event-data("Discard?"=w1237) -> ()  [unwired: 4 in, 1 out]
      }
      event "Run/Sequence Error", "Update Error", "Table error": Value Change {
        n770 = event-data() -> ("CtlRef"=w1261:refnum<vi>, "NewVal"=w1263:errorcluster)  [unwired: 1 in]
        n771 = Format Date/Time String() -> (date/time string=w1262:string)  [unwired: 3 in]
        n772 = case shown="Error" w1263 {
          selector: w1263 -> [_ w1276]
          tunnel: w1262 -> [_ w1271]
          tunnel: w1261 -> [_ w1277]
          frame No Error {
          }
          frame Error {
            w1265 = T12."Enabled" ("Disabled")
            w1266 = FALSE
            # "If an error was generated in any part of the program, automatically open the Errors tab."
            n773 = property on="Error Log" class="MCListbox (strict)"() -> (error out=w1268:errorcluster, "ItemNames"=w1281:string[][])  [unwired: 2 in, 1 out]
            n774 = property class="Clust (strict)"(reference=w1277, error in=w1268) -> (error out=w1269:errorcluster, "Label.Text"=w1272:string)  [unwired: 1 out]
            n775 = Unbundle By Name(w1276) -> ("code"=w1275:i32, "source"=w1273:string)
            n776 = Number To Decimal String(number=w1275) -> (decimal integer string=w1274:string)  [unwired: 1 in]
            n777 = Build Array(w1271, w1272, w1274, w1273) -> (w1270:string[])
            n778 = Build Array (concatenate)(w1270, w1281) -> (w1280:string[][])
            n779 = Array Subset(array=w1280, length (row)=10 ("length")) -> (w1279:string[][])  [unwired: 3 in]
            n780 = property on="Error Log" class="MCListbox (strict)"(error in=w1269, "ItemNames"=w1279) -> (error out=w1267:errorcluster)  [unwired: 1 in, 1 out]
            n781 = property on="Tab Control" class="TabCtl (strict)"(error in=w1267, "Value"=T23."Errors" ("Tab Control")) -> ()  [unwired: 1 in, 2 out]
            n782 = property on="Run Button" class="Bool (strict)"("Value"=w1266, "DisabledEnum"=w1265) -> ()  [unwired: 2 in, 2 out]
            n783 = property on="Run Seq Button" class="Bool (strict)"("Value"=w1266, "DisabledEnum"=w1265) -> ()  [unwired: 2 in, 2 out]
            n784 = property on="RandomSequence" class="Bool (strict)"("DisabledEnum"=w1265) -> ()  [unwired: 2 in, 2 out]
            n785 = property on="StopExperiment" class="Bool (strict)"("Value"=w1266, "DisabledEnum"=T12."Disabled and Grayed Out" ("Disabled")) -> ()  [unwired: 2 in, 2 out]
          }
        }
      }
      event "Hide Checked Devices": Mouse Down {
        n786 = event-data() -> ("Button"=w1283:u16)  [unwired: 1 in]
        n787 = case shown="1" w1283 {
          frame 0, Default {
          }
          frame 1 {
            w1294 = 38
            # "Toggle checkbox, change pref."
            n788 = property on="Hide Checked Devices" class="LstBox (strict)"() -> (error out=w1290:errorcluster, "Item Symbols"=w1296:i32[], "Item Names"=w1289:string[])  [unwired: 2 in, 1 out]
            n789 = global read "PrefsGlobal.vi" "SetListPrefs.lvclass"() -> (w1286:refnum<class "SetListPrefs.lvclass">)
            n790 = Index Array(array=w1289, index="Hide Checked Devices") -> (element=w1287:string)
            n791 = Index Array(array=w1296, index="Hide Checked Devices") -> (element=w1295:i32)
            n792 = Equal?(x=w1295, y=w1294) -> (x = y?=w1291:bool)
            n793 = case shown="True" w1291 {
              tunnel: w1290 -> [w1301 w1307]
              tunnel: [w1302 w1306] -> w1284
              tunnel: w1287 -> [w1300 w1305]
              tunnel: [w1299 w1304] -> w1285
              tunnel: w1286 -> [w1298 w1303]
              frame False {
                n794 = call "AddHiddenDevice.vi"("error in (no error)"=w1301, "DeviceToHide"=w1300, "SetListPrefs in"=w1298) -> ("error out"=w1302:errorcluster, "SetListPrefs out"=w1299:refnum<class "SetListPrefs.lvclass">)
              }
              frame True {
                n795 = call "RemoveHiddenDevice.vi"("error in (no error)"=w1307, "DeviceToShow"=w1305, "SetListPrefs in"=w1303) -> ("error out"=w1306:errorcluster, "SetListPrefs out"=w1304:refnum<class "SetListPrefs.lvclass">)
              }
            }
            n796 = Select(t=37, s=w1291, f=w1294) -> (s? t:f=w1292:i32)
            n797 = Replace Array Subset(array=w1296, new element=w1292, index="Hide Checked Devices") -> (w1297:i32[])
            n798 = global write "PrefsGlobal.vi" "SetListPrefs.lvclass"(w1285) -> ()
            n799 = property on="Hide Checked Devices" class="LstBox (strict)"(error in=w1284, "Item Symbols"=w1297) -> ()  [unwired: 1 in, 2 out]
          }
        }
      }
      event "Auto PressHWUpdate": Value Change {
        n800 = event-data() -> ("NewVal"=w1308:bool)  [unwired: 1 in]
        n801 = global read "PrefsGlobal.vi" "SetListPrefs.lvclass"() -> (w1310:refnum<class "SetListPrefs.lvclass">)
        n802 = call "Write AutoPressHWUpdate.vi"("AutoPressHWUpdate"=w1308, "SetListPrefs in"=w1310) -> ("SetListPrefs out"=w1309:refnum<class "SetListPrefs.lvclass">)  [unwired: 8 in, 1 out]
        n803 = global write "PrefsGlobal.vi" "SetListPrefs.lvclass"(w1309) -> ()
      }
      event "Reset to Saved Window Position": Value Change {
        n804 = event-data() -> ("NewVal"=w1311:bool)  [unwired: 1 in]
        n805 = case shown="False" w1311 {
          frame False {
            # "False to catch mouse release"
            n806 = global read "PrefsGlobal.vi" "SetListPrefs.lvclass"() -> (w1313:refnum<class "SetListPrefs.lvclass">)
            n807 = call "Read WindowBounds.vi"("SetListPrefs in"=w1313) -> ("Rect"=w1312:T13)  [unwired: 8 in, 2 out]
            n808 = Unbundle By Name(w1312) -> ("Right"=w1314:i16, "Left"=w1327:i16, "Bottom"=w1326:i16, "Top"=w1325:i16)
            n809 = control-ref of="This VI"() -> (w1330:refnum<vi>)
            n810 = Subtract(x=w1314, y=w1327) -> (x-y=w1315:i16)
            n811 = Subtract(x=w1326, y=w1325) -> (x-y=w1324:i16)
            n812 = property class="VI"(reference=w1330, "Front Panel.PanelBounds"=w1312) -> (error out=w1316:errorcluster)  [unwired: 1 in, 1 out]
            n813 = Subtract(x=w1315, y=u32 24) -> (x-y=w1317:u32)
            n814 = Subtract(x=w1324, y=u32 85) -> (x-y=w1318:u32)
            n815 = property on="Tab Control" class="TabCtl (strict)"(error in=w1316, "PaneWidth"=w1317, "PaneHeight"=w1318) -> (error out=w1319:errorcluster)  [unwired: 1 in, 1 out]
            n816 = Subtract(x=w1317, y=u32 16) -> (x-y=w1321:u32)
            n817 = Subtract(x=w1318, y=u32 86) -> (x-y=w1320:u32)
            n818 = property on="SetList Table" class="Tbl (strict)"(error in=w1319, "Width"=w1321, "Height"=w1320) -> ()  [unwired: 1 in, 2 out]
          }
          frame True {
            # "True: Mouse down, do nothing"
          }
        }
      }
      event "Save Current Window Position": Value Change {
        n819 = event-data() -> ("OldVal"=w1331:bool)  [unwired: 1 in]
        n820 = case shown="True" w1331 {
          frame False {
          }
          frame True {
            n821 = control-ref of="This VI"() -> (w1332:refnum<vi>)
            n822 = global read "PrefsGlobal.vi" "SetListPrefs.lvclass"() -> (w1336:refnum<class "SetListPrefs.lvclass">)
            n823 = property class="VI"(reference=w1332) -> (error out=w1333:errorcluster, "Front Panel.PanelBounds"=w1334:T13)  [unwired: 1 in, 1 out]
            n824 = call "Write WindowBounds.vi"("error in (no error)"=w1333, "Rect"=w1334, "SetListPrefs in"=w1336) -> ("SetListPrefs out"=w1335:refnum<class "SetListPrefs.lvclass">)  [unwired: 7 in, 1 out]
            n825 = global write "PrefsGlobal.vi" "SetListPrefs.lvclass"(w1335) -> ()
          }
        }
      }
      event "AutoGitCmd", "ManGitCmd": Value Change {
        n826 = event-data() -> ()  [unwired: 1 in, 1 out]
        n827 = global read "PrefsGlobal.vi" "SetListPrefs.lvclass"() -> (w1340:refnum<class "SetListPrefs.lvclass">)
        n828 = local read "Git Command"() -> (w1338:string)
        n829 = case shown="False" "AutoGitCmd" {
          tunnel: w1338 -> [w1343 w1357]
          tunnel: [w1342 w1364] -> w1339
          tunnel: w1340 -> [w1341 w1363]
          frame False {
            n830 = case shown="True" "ManGitCmd" {
              tunnel: w1343 -> [w1345 w1348]
              tunnel: [w1345 w1347] -> w1342
              tunnel: w1341 -> [_ w1350]
              frame False {
              }
              frame True {
                n831 = call "Enter Git Command"() -> ("Git Command"=w1349:string, "OK"=w1346:bool)  [unwired: 17 in, 1 out]
                n832 = case shown="True" w1346 {
                  tunnel: w1349 -> [_ w1352]
                  tunnel: w1350 -> [_ w1356]
                  tunnel: w1348 -> [w1351 _]
                  tunnel: [w1351 w1352] -> w1347
                  frame False {
                  }
                  frame True {
                    n833 = call "Write GitCmd.vi"("GitCmd"=w1352, "SetListPrefs in"=w1356) -> ("error out"=w1355:errorcluster, "SetListPrefs out"=w1354:refnum<class "SetListPrefs.lvclass">)  [unwired: 8 in]
                    n834 = call "SaveOnly.vi"("error in (no error)"=w1355, "Preferences in"=w1354) -> ("Preferences out"=w1353:refnum<class "SetListPrefs.lvclass">)  [unwired: 7 in, 2 out]
                    n835 = global write "PrefsGlobal.vi" "SetListPrefs.lvclass"(w1353) -> ()
                  }
                }
              }
            }
          }
          frame True {
            n836 = call "FindGit.vi"() -> ("User Cancelled"=w1360:bool, "Git String"=w1362:string)  [unwired: 9 in, 1 out]
            n837 = Not Equal?(x=w1357, y=w1362) -> (x != y?=w1361:bool)
            n838 = Not(x=w1360) -> (.not. x?=w1359:bool)
            n839 = Select(t=w1357, s=w1360, f=w1362) -> (s? t:f=w1364:string)
            n840 = And(x=w1359, y=w1361) -> (x .and. y?=w1358:bool)
            n841 = case shown="True" w1358 {
              tunnel: w1362 -> [_ w1368]
              tunnel: w1363 -> [_ w1369]
              frame False {
              }
              frame True {
                n842 = call "Write GitCmd.vi"("GitCmd"=w1368, "SetListPrefs in"=w1369) -> ("error out"=w1367:errorcluster, "SetListPrefs out"=w1366:refnum<class "SetListPrefs.lvclass">)  [unwired: 8 in]
                n843 = call "SaveOnly.vi"("error in (no error)"=w1367, "Preferences in"=w1366) -> ("Preferences out"=w1365:refnum<class "SetListPrefs.lvclass">)  [unwired: 7 in, 2 out]
                n844 = global write "PrefsGlobal.vi" "SetListPrefs.lvclass"(w1365) -> ()
              }
            }
          }
        }
        "Git Command" <- w1339
      }
    }
    "Table error" <- w175
    n845 = disable-structure shown="Enabled" {
      frame Disabled {
        # "diagnositc"
        n846 = local read "Table History"() -> (w180:T7)
        n847 = Unbundle By Name(w180) -> ("OldTable Array"=w179:T8)
        n848 = Array Size(array=w179) -> (size(s)=→"Hist. size":i32)
      }
      frame Enabled {
        # "Faster without\ndiagnostic info"
        # "No Diagnostic"
      }
    }
  }
  n849 = local read "FunctionMenu"() -> (w97:refnum<class "InsertFunctionMenu.lvclass">)
  n850 = Obtain Notifier(notification data type=w127) -> (notifier out=→"Update Notifier":refnum<notifier>)  [unwired: 3 in, 2 out]
  n851 = call "Caching_Expression_Evaluator_Table.vi"("method"=t_Caching_Expression_Evaluator_Methods_Table."execute", "expression/scriptlet"="User defined functions") -> ("error out"=w99:errorcluster)  [unwired: 11 in, 2 out]
  n852 = call-dynamic "ParseUserFunctions.vi"("error in (no error)"=w99, "User defined functions in"="User defined functions", "FunctionMenu in"=w97) -> ("FunctionMenu out"=w96:refnum<class "InsertFunctionMenu.lvclass">)  [unwired: 7 in, 1 out]
  n853 = local write "FunctionMenu"(w96) -> ()
  n854 = local write "UpdateHWI Button"(FALSE ("UpdateHWI Button")) -> ()
  n855 = invoke on="quit" class="Bool (strict)" method="Reinit To Default"() -> ()  [unwired: 3 in, 3 out]
  n856 = property on="UpdateHWI Button" class="Bool (strict)"("DisabledEnum"=T12."Disabled and Grayed Out" ("Disabled")) -> ()  [unwired: 2 in, 2 out]
  n857 = property on="Loading Text" class="Str"("Visible"=FALSE ("Load from Disk")) -> ()  [unwired: 2 in, 2 out]
  n858 = property on="Run Button" class="Bool (strict)"("Value"=w109, "DisabledEnum"=w110) -> ()  [unwired: 2 in, 2 out]
  n859 = property on="Run Seq Button" class="Bool (strict)"("Value"=w109, "DisabledEnum"=w110) -> ()  [unwired: 2 in, 2 out]
  n860 = property on="RandomSequence" class="Bool (strict)"("DisabledEnum"=w110) -> ()  [unwired: 2 in, 2 out]
  n861 = property on="StopExperiment" class="Bool (strict)"("Value"=w109, "DisabledEnum"=T12."Disabled and Grayed Out" ("Disabled")) -> ()  [unwired: 2 in, 2 out]
  n862 = while {
    stop <- w1370 stop-if-true
    # "Update Event Structure"
    n863 = local read "Dyn. Regist. Update Event"() -> (w1371:refnum<event-registration>)
    n864 = event shown="[0] <Update Event>: User Event" {
      selector: w1371 -> [_ _]
      dyn-events: _ -> [_ _]
      timeout: _ -> [_ _]
      tunnel: [_ w1413] -> w1370
      event User Event {
        n865 = event-data() -> ("Seq. Idx"=w1372:i32, "Force?"=w1373:bool)  [unwired: 1 in]
        n866 = case shown="True" w1373 {
          tunnel: [_ w1378] -> w1374
          tunnel: w1372 -> [_ w1387]
          frame False {
          }
          frame True {
            # "prepend filenumber placeholder\n(overwritten in CycleX loop)"
            n867 = property on="SequenceHistory" class="Tbl (strict)"() -> ("Value"=w1390:string[][])  [unwired: 2 in, 2 out]
            n868 = control-ref of="VariableManager"() -> (w1377:refnum<vi>)
            n869 = Index Array(array=w1390, index (row)=w1387, index (col)=1 ("disabled index (col)")) -> (element=w1391:string)
            n870 = Scan From String(format string="%d", input string=w1391) -> (output 1=w1386:i32)  [unwired: 3 in, 3 out]
            n871 = call "GetVariableValues.vi"("SequenceStep"=w1386, "VariableManagerRef in"=w1377) -> ("error out"=w1381:errorcluster, "VariableValues"=w1398:refnum<class "VariableValue.lvclass">[])  [unwired: 7 in, 1 out]
            n872 = control-ref of="SetList Table"() -> (w1406:refnum<vi>)
            n873 = for {
              tunnel: w1398 -> [w1409] mode=indexing
              tunnel: [w1410] -> w1399 mode=indexing
              tunnel: [w1408] -> w1397 mode=indexing
              n874 = call "VariableValueToCluster.vi"("VariableValue"=w1409) -> ("VariableValueCluster"=w1408:cluster{"Name":string, "Value":dbl})  [unwired: 10 in]
              n875 = call "VariableValueToString.vi"("VariableValue"=w1409) -> ("VariableValueString"=w1410:string)  [unwired: 10 in]
            }
            n876 = call "Construct Sequence Variable Igor String.vi"("error in (no error)"=w1381, "Current index"=w1387, "VariableManagerRef"=w1377) -> ("error out"=w1380:errorcluster, "Igor Instruction String"=w1382:string[])  [unwired: 7 in]
            n877 = property class="Tbl (strict)"(reference=w1406, error in=w1381) -> (error out=w1400:errorcluster, "Value"=w1403:string[][], "Column Headers[]"=w1402:string[])  [unwired: 1 out]
            n878 = local read "Devices queue"() -> (w1376:refnum<queue>)
            n879 = local read "DevNums"() -> (w1407:i32[])
            n880 = Concatenate Strings(w1399) -> (w1395:string)
            n881 = call "SetList SWI to Devices.vi"("error in (no error)"=w1400, "SWI table"=w1403, "DevNums In"=w1407, "Devices queue"=w1376) -> ("error out"=w1404:errorcluster, "Devices queue out"=w1405:refnum<queue>)  [unwired: 5 in, 1 out]
            n882 = invoke on="SequenceHistory" class="Tbl (strict)" method="Set Cell Value"("X Index"=3 ("disabled index (col)"), "Y Index"=w1387, "Value"=w1395) -> ()  [unwired: 3 in, 6 out]
            n883 = call "SetList_ToString.vi"("Column Names"=w1402, "Current  Variables"=w1397, "Device Data"=w1403) -> ("Igor Inform String"=w1401:string)
            n884 = local read "Additional wait time (s)"() -> (w1385:dbl)
            n885 = call "Update HWI.vi"("Error In"=w1404, "Current Variables"=w1397, "Devices queue"=w1405) -> ("Error Out"=w1379:errorcluster, "Total Time"=w1384:dbl)  [unwired: 1 in, 1 out]
            n886 = Merge Errors(w1379, w1380) -> (w1378:errorcluster)
            n887 = property on="Update Error" class="Clust (strict)"("Val(Sgnl)"=w1378) -> ()  [unwired: 2 in, 2 out]
            n888 = Build Array (concatenate)(w1382, w1401) -> (w1393:string[])
            n889 = case shown="..-1" w1386 {
              tunnel: w1378 -> [_ w1411]
              frame 0, Default {
              }
              frame ..-1 {
                n890 = case shown="No Error" w1411 {
                  frame No Error {
                    n891 = property on="UpdateHWI Button" class="Bool (strict)"("DisabledEnum"=T12."Disabled and Grayed Out" ("Disabled")) -> ()  [unwired: 2 in, 2 out]
                  }
                  frame Error {
                  }
                }
              }
            }
            n892 = Add(x=w1384, y=w1385) -> (x+y=→"Cycle Time (s)":dbl)
            n893 = Build Array (concatenate)("FileNumber=null\n", w1393) -> (→"Igor Inform Array":string[])
          }
        }
        n894 = local read "Update Notifier"() -> (w1375:refnum<notifier>)
        n895 = Send Notification(notification=w1374, notifier=w1375) -> ()  [unwired: 1 in, 2 out]
      }
      event "quit": Value Change {
        # "Tried adding local variable read of Quit outside event loop, but I think it wasn't being read properly.\nIs there a problem having three event loops checking quit? - CDH\nI think if you wanted it to work as intended with the read outside of the loop, you would need to set a timeout value and event case. - ZES"
        n896 = event-data() -> ("NewVal"=w1413:bool)  [unwired: 1 in, 1 out]
      }
    }
  }
  n897 = while {
    stop <- w1414 stop-if-true
    # "Sequence Event Structure"
    n898 = local read "Dyn.\nRegist.\nSeq.\nEvent"() -> (w1415:refnum<event-registration>)
    n899 = event shown="[0] <Seq Event>: User Event" {
      selector: w1415 -> [_ _]
      dyn-events: _ -> [_ _]
      timeout: _ -> [_ _]
      tunnel: [_ w1481] -> w1414
      event User Event {
        n900 = event-data() -> ()  [unwired: 1 in, 2 out]
        n901 = property on="StopExperiment" class="Bool (strict)"() -> ("Value"=w1416:bool)  [unwired: 2 in, 2 out]
        n902 = case shown="False" w1416 {
          frame False {
            # "If running cycle, do not force update."
            # "Look for waiting sequence"
            # "Run Experiment"
            n903 = property on="SequenceHistory" class="Tbl (strict)"() -> ("Value"=w1424:string[][])  [unwired: 2 in, 2 out]
            n904 = Index Array(array=w1424, index (col)=2 ("disabled index (col)")) -> (element=w1426:string[])  [unwired: 1 in]
            n905 = for {
              tunnel: w1426 -> [w1430] mode=indexing
              tunnel: [w1428] -> w1423
              tunnel: [w1427] -> w1421
              i -> [w1427]
              stop <- w1428 stop-if-true
              n906 = Equal?(x=w1430, y="Waiting") -> (x = y?=w1428:bool)
            }
            n907 = property on="SequenceHistory" class="Tbl (strict)"() -> ("Value"=w1417:string[][])  [unwired: 2 in, 2 out]
            n908 = Index Array(array=w1417, index (row)=w1421, index (col)=1 ("disabled index (col)")) -> (element=w1420:string)
            n909 = Not Equal?(x=w1420, y="-1") -> (x != y?=w1418:bool)
            n910 = case shown="False" w1423 {
              tunnel: w1421 -> [_ w1446]
              tunnel: w1418 -> [_ w1445]
              frame False {
                # "No Waiting Sequence"
                n911 = local read "FBVarSeqSetJSON queue"() -> (w1432:refnum<queue>)
                n912 = control-ref of="VariableManager"() -> (w1431:refnum<vi>)
                n913 = Dequeue Element(queue=w1432, timeout in ms (-1)=0) -> (element=w1434:T9, timed out?=w1436:bool, error out=w1435:errorcluster)  [unwired: 1 in, 1 out]
                n914 = case shown="False" w1436 {
                  tunnel: w1434 -> [w1439 _]
                  tunnel: w1435 -> [w1440 _]
                  tunnel: w1431 -> [w1438 _]
                  frame False {
                    # "Reset sequence and\nrun with new varset"
                    n915 = call "LoadJSONVarSetIntoVM.vi"("error in (no error)"=w1440, "JSONVarSet"=w1439, "VariableManagerRef in"=w1438) -> ("error out"=w1437:errorcluster)  [unwired: 7 in, 1 out]
                    n916 = property on="Run Seq Button" class="Bool (strict)"(error in=w1437, "Val(Sgnl)"=TRUE ("Value (Signaling)")) -> ()  [unwired: 1 in, 2 out]
                  }
                  frame True {
                    w1443 = T12."Enabled" ("Disabled")
                    w1442 = FALSE
                    n917 = property on="Run Button" class="Bool (strict)"("Value"=w1442, "DisabledEnum"=w1443) -> ()  [unwired: 2 in, 2 out]
                    n918 = property on="Run Seq Button" class="Bool (strict)"("Value"=w1442, "DisabledEnum"=w1443) -> ()  [unwired: 2 in, 2 out]
                    n919 = property on="RandomSequence" class="Bool (strict)"("DisabledEnum"=w1443) -> ()  [unwired: 2 in, 2 out]
                    n920 = property on="StopExperiment" class="Bool (strict)"("Value"=w1442, "DisabledEnum"=T12."Disabled and Grayed Out" ("Disabled")) -> ()  [unwired: 2 in, 2 out]
                  }
                }
              }
              frame True {
                # "Run Waiting Sequence"
                n921 = stacked-sequence {
                  seq-local: [_ w1453 _ _] -> [_ _ _ w1474]
                  tunnel: w1446 -> [w1448 w1452 w1471 w1473]
                  tunnel: w1445 -> [_ w1451 _ _]
                  frame #0 {
                    # "Update SequenceHistory Status"
                    n922 = invoke on="SequenceHistory" class="Tbl (strict)" method="Set Cell Value"("X Index"=2 ("disabled index (col)"), "Y Index"=w1448, "Value"="Programming") -> ()  [unwired: 3 in, 6 out]
                  }
                  frame #1 {
                    # "Row number of waiting sequence"
                    n923 = case shown="False" w1451 {
                      selector: w1451 -> [_ w1469]
                      tunnel: [w1460 w1469] -> w1450
                      frame False {
                        # "Force update if changing\nvars"
                        # "Active in Cycle Mode, so Update Vars"
                        n924 = local read "FBVarSeqSetJSON queue"() -> (w1464:refnum<queue>)
                        n925 = control-ref of="VariableManager"() -> (w1459:refnum<vi>)
                        n926 = Dequeue Element(queue=w1464, timeout in ms (-1)=0) -> (element=w1461:T9, timed out?=w1463:bool, error out=w1462:errorcluster)  [unwired: 1 in, 1 out]
                        n927 = Not(x=w1463) -> (.not. x?=w1460:bool)
                        n928 = case shown="True" w1460 {
                          tunnel: w1462 -> [_ w1466]
                          tunnel: w1461 -> [_ w1467]
                          tunnel: w1459 -> [_ w1468]
                          frame False {
                          }
                          frame True {
                            n929 = call "LoadJSONVarSetIntoVM.vi"("error in (no error)"=w1466, "JSONVarSet"=w1467, "VariableManagerRef in"=w1468) -> ()  [unwired: 7 in, 2 out]
                          }
                        }
                      }
                      frame True {
                        # "Active in Sequence Mode"
                      }
                    }
                    n930 = local read "Update Notifier"() -> (w1455:refnum<notifier>)
                    n931 = local read "Update Event"() -> (w1458:refnum<user-event>)
                    n932 = Bundle(w1452, w1450) -> (w1457:cluster{i32, bool})  [unwired: 1 in]
                    n933 = Generate User Event(user event=w1458, event data cluster=w1457) -> (error out=w1454:errorcluster)  [unwired: 2 in, 1 out]
                    n934 = Wait on Notification(notifier=w1455, ignore previous (F)=TRUE, error in (no error)=w1454) -> (notification=w1453:errorcluster)  [unwired: 1 in, 3 out]
                  }
                  frame #2 {
                    # "Update SequenceHistory Status"
                    n935 = invoke on="SequenceHistory" class="Tbl (strict)" method="Set Cell Value"("X Index"=2 ("disabled index (col)"), "Y Index"=w1471, "Value"="Executing") -> ()  [unwired: 3 in, 6 out]
                  }
                  frame #3 {
                    n936 = local read "CycleX Event"() -> (w1476:refnum<user-event>)
                    n937 = Bundle(w1473, FALSE) -> (w1477:cluster{i32, bool})  [unwired: 1 in]
                    n938 = Generate User Event(user event=w1476, event data cluster=w1477, error in=w1474) -> ()  [unwired: 1 in, 2 out]
                  }
                }
              }
            }
          }
          frame True {
            w1479 = T12."Enabled" ("Disabled")
            w1480 = FALSE
            # "Stop experiment when Stop request"
            n939 = property on="Run Button" class="Bool (strict)"("Value"=w1480, "DisabledEnum"=w1479) -> ()  [unwired: 2 in, 2 out]
            n940 = property on="Run Seq Button" class="Bool (strict)"("Value"=w1480, "DisabledEnum"=w1479) -> ()  [unwired: 2 in, 2 out]
            n941 = property on="RandomSequence" class="Bool (strict)"("DisabledEnum"=w1479) -> ()  [unwired: 2 in, 2 out]
            n942 = property on="StopExperiment" class="Bool (strict)"("Value"=w1480, "DisabledEnum"=T12."Disabled and Grayed Out" ("Disabled")) -> ()  [unwired: 2 in, 2 out]
          }
        }
      }
      event "quit": Value Change {
        n943 = event-data() -> ("NewVal"=w1481:bool)  [unwired: 1 in, 1 out]
      }
    }
  }
  n944 = Get Date/Time In Seconds() -> (seconds since 1Jan1904=w28:timestamp)
  n945 = To Quad Integer(1:w28) -> (0:w27:i64)
  n946 = disable-structure shown="Disabled" {
    frame Disabled {
      n947 = while {
        i -> [w1486]
        stop <- w1482 stop-if-true
        # "Diagnostics..."
        n948 = flat-sequence {
          tunnel: [w1495] -> w1483
          frame #0 {
            n949 = Wait (ms)(milliseconds to wait=u32 100) -> ()  [unwired: 1 out]
          }
          frame #1 {
            n950 = property on="SetList Table" class="Tbl (strict)"() -> (error out=w1491:errorcluster, "OwningVI"=w1493:refnum<vi>)  [unwired: 2 in, 1 out]
            n951 = property on="SetList Table" class="Tbl (strict)"() -> ("Key Focus"=→"Key Focus":bool, "EditPos"=→"Edit Position":T4, "Selection Size"=→"Selection Size":T4, "Selection Start"=→"Selection Start":T4, "Index Values"=→"Index Values":T3)  [unwired: 2 in, 2 out]
            n952 = local read "quit"() -> (w1495:bool)
            n953 = property class="VI"(reference=w1493, error in=w1491) -> (error out=w1490:errorcluster, "Panel"=w1492:refnum<vi>)  [unwired: 1 out]
            n954 = property class="Pnl"(reference=w1492, error in=w1490) -> ("DeferPanUpdts"=→"Defer Pnl Upd":bool)  [unwired: 2 out]
            n955 = local write "Val Change"(FALSE ("Val Change")) -> ()
          }
        }
        n956 = Not(x="Diag. loop?") -> (.not. x?=w1484:bool)
        n957 = Or(x=w1483, y=w1484) -> (x .or. y?=w1482:bool)
        "diag. loop cnt" <- w1486
      }
    }
    frame Enabled {
    }
  }
  n958 = while {
    shift-right: [w1504] -> _
    shift-left: w27 -> [w1503]
    shift-right: [w1502] -> _
    shift-left: i64 600 -> [w1501]
    stop <- w1500 stop-if-true
    # "Auto-Save\nPeriod"
    # "Last Save/Load"
    # "Autosave Loop"
    n959 = event shown="[0] Timeout" {
      selector: _ -> [_ _ _]
      dyn-events: _ -> [_ _ _]
      timeout: 15000 -> [_ _ _]
      tunnel: [w1506 w1553 w1555] -> w1504
      tunnel: w1503 -> [w1507 w1553 _]
      tunnel: [w1511 w1552 w1557] -> w1502
      tunnel: w1501 -> [w1511 w1552 w1557]
      tunnel: [FALSE ("NewVal") w1551 FALSE ("NewVal")] -> w1500
      event Timeout {
        # "Timeout every 15s, check if save time"
        n960 = event-data() -> ()  [unwired: 1 in, 1 out]
        n961 = Get Date/Time In Seconds() -> (seconds since 1Jan1904=w1513:timestamp)
        n962 = To Quad Integer(1:w1513) -> (0:w1508:i64)
        n963 = Subtract(x=w1508, y=w1507) -> (x-y=w1512:i64)
        n964 = Less Or Equal?(x=w1511, y=w1512) -> (x <= y?=w1509:bool)
        n965 = case shown="True" w1509 {
          frame False {
          }
          frame True {
            # "Autosave!"
            n966 = local read "Devices queue"() -> (w1523:refnum<queue>)
            n967 = local read "DevNums"() -> (w1524:i32[])
            n968 = property on="SetList Table" class="Tbl (strict)"() -> (error out=w1525:errorcluster, "Value"=w1526:string[][])  [unwired: 2 in, 1 out]
            n969 = property on="Select Layout" class="Ring (strict)"() -> ("Value"=w1516:i32, "StringsAndValues[]"=w1515:T20)  [unwired: 2 in, 2 out]
            n970 = local read "User defined functions"() -> (w1517:string)
            n971 = control-ref of="VariableManager"() -> (w1522:refnum<vi>)
            n972 = global read "PrefsGlobal.vi" "SetListPrefs.lvclass"() -> (w1531:refnum<class "SetListPrefs.lvclass">)
            n973 = call "Read ProcRepo.vi"("SetListPrefs in"=w1531) -> ("error out"=w1535:errorcluster, "ProcRepo"=w1532:path)  [unwired: 8 in, 1 out]
            n974 = Current VI's Path() -> (path=w1527:path)
            n975 = call "SetList SWI to Devices.vi"("error in (no error)"=w1525, "SWI table"=w1526, "DevNums In"=w1524, "Devices queue"=w1523) -> ("Devices out"=w1520:refnum<class "Device.lvclass">[])  [unwired: 5 in, 2 out]
            n976 = call "VMExport.vi"("VariableManagerRef in"=w1522) -> ("VariableManagerExportCopy"=w1519:refnum<class "VariableManager.lvclass">)  [unwired: 8 in, 2 out]
            n977 = call "GetVersionString.vi"("SetList root path"=w1527) -> ("Version String"=w1518:string)  [unwired: 2 in]
            n978 = Build Path(base path=w1532, name or relative path="AutoSaves\\") -> (appended path=w1534:path)
            n979 = call <vilib>:"Check if File or Folder Exists.vi"("error in (no error)"=w1535, "path"=w1534) -> ("error out"=w1537:errorcluster, "file or folder exists?"=w1538:bool, "dup path"=w1536:path)  [unwired: 7 in]
            n980 = local read "Procedure Name"() -> (w1528:string)
            n981 = Bundle By Name(cluster=T19 {"Version"="", "Devices"=[], "Select Layout"=0, "Layout:Strings And Values []"=[], "User defined functions"="", "VariableManager"=refnum}, "Version"=w1518, "Devices"=w1520, "Select Layout"=w1516, "Layout:Strings And Values []"=w1515, "User defined functions"=w1517, "VariableManager"=w1519) -> (w1521:T19)
            n982 = case shown="False" w1538 {
              tunnel: w1536 -> [w1544 w1546]
              tunnel: w1537 -> [w1543 w1545]
              tunnel: [w1542 w1545] -> w1529
              tunnel: [w1541 w1546] -> w1530
              frame False {
                n983 = Create Folder(path (use dialog)=w1544, error in=w1543) -> (created path=w1541:path, error out=w1542:errorcluster)  [unwired: 1 in, 1 out]
              }
              frame True {
              }
            }
            n984 = call "Autosave.vi"("error in (no error)"=w1529, "Base Name"=w1528, "Save Cluster"=w1521, "Autosave Path"=w1530) -> ("error out (passthrough)"=w1540:errorcluster, "Autosave Success"=w1539:bool)  [unwired: 6 in]
            n985 = case shown="True" w1539 {
              tunnel: w1540 -> [w1547 w1550]
              tunnel: w1530 -> [_ w1548]
              frame False {
                n986 = call <vilib>:"Clear Errors.vi"("error in (no error)"=w1547) -> ()  [unwired: 6 in, 1 out]
              }
              frame True {
                n987 = call "PruneAutosaves.vi"("error in"=w1550, "Autosave Depth"=20, "Autosave Directory"=w1548) -> ()  [unwired: 4 in, 5 out]
              }
            }
          }
        }
        n988 = Select(t=w1508, s=w1509, f=w1507) -> (s? t:f=w1506:i64)
      }
      event "quit": Value Change {
        n989 = event-data() -> ("NewVal"=w1551:bool)  [unwired: 1 in, 5 out]
      }
      event "Load from File", "Load keep cur. format", "Load Old", "Load Recent", "Save to Repo", "Load from Repo": Value Change {
        # "New Save/Load Time"
        n990 = event-data() -> ()  [unwired: 1 in, 1 out]
        n991 = Get Date/Time In Seconds() -> (seconds since 1Jan1904=w1556:timestamp)
        n992 = To Quad Integer(1:w1556) -> (0:w1555:i64)
      }
    }
  }
  n993 = property on="TCP Quit Signal" class="Bool (strict)"("Value"=FALSE ("TCP Quit Signal")) -> (error out=w48:errorcluster)  [unwired: 2 in, 1 out]
  n994 = control-ref of="VariableManager"() -> (w21:refnum<vi>)
  n995 = control-ref of="SequenceHistory"() -> (w60:refnum<vi>)
  n996 = Obtain Queue(name (unnamed)=w56, element data type=w56, error in (no error)=w48) -> (queue out=w61:refnum<queue>, error out=w57:errorcluster)  [unwired: 2 in, 1 out]
  n997 = Obtain Queue(name (unnamed)="FBVarSetJSONNow", element data type=T9 [] ("JSONVarSet"), error in (no error)=w48) -> (queue out=w54:refnum<queue>, error out=w44:errorcluster)  [unwired: 2 in, 1 out]
  n998 = while {
    stop <- w1558 stop-if-true
    # "Handles running CycleX, which runs once per step"
    n999 = local read "Dyn.\nRegist.\nCycleX\nEvent"() -> (w1559:refnum<event-registration>)
    n1000 = event shown="[0] <CycleX Event>: User Event" {
      selector: w1559 -> [_ _]
      dyn-events: _ -> [_ _]
      timeout: _ -> [_ _]
      tunnel: [_ w1606] -> w1558
      event User Event {
        # "log file number"
        # "replace file number"
        n1001 = event-data() -> ("Seq. Idx"=w1564:i32)  [unwired: 1 in, 1 out]
        n1002 = local read "File Number"() -> (w1567:i32)
        n1003 = local read "Load Long Hash/Filename"() -> (w1562:string)
        n1004 = Format Into String(format string="%d", w1567) -> (resulting string=w1565:string)  [unwired: 2 in, 1 out]
        n1005 = local read "Igor Inform Array"() -> (w1575:string[])
        n1006 = invoke on="SequenceHistory" class="Tbl (strict)" method="Set Cell Value"("X Index"=0, "Y Index"=w1564, "Value"=w1565) -> ()  [unwired: 3 in, 6 out]
        n1007 = Increment(x=w1567) -> (x+1=w1579:i32)
        n1008 = local write "File Number"(w1579) -> ()
        n1009 = shared-variable ".\\VariableLibrary.lvlib\\FileNum"(w1579) -> ()  [unwired: 1 in, 1 out]
        n1010 = Concatenate Strings("FileNumber=" ("string"), w1565, "\n" ("string")) -> (w1569:string)
        n1011 = Format Into String(format string="LastSave=%s\n" ("string"), w1562) -> (resulting string=w1560:string)  [unwired: 2 in, 1 out]
        n1012 = Replace Array Subset(array=w1575, new element=w1569, index=0) -> (w1573:string[])
        n1013 = Concatenate Strings(w1560, w1573) -> (w1580:string)
        "Igor Inform String" <- w1580
        n1014 = Build Array(w1580) -> (w1576:string[])
        n1015 = local read "Devices queue"() -> (w1563:refnum<queue>)
        n1016 = call "CycleX.vi"("Devices queue"=w1563, "Program only changes"="Program only changes", "Program during MOT loading"="Program during MOT loading", "Igor Inform String"=w1576, "Additional wait time (s)"="Additional wait time (s)") -> ("error out"=w1572:errorcluster)  [unwired: 10 in]
        n1017 = case shown="No Error" w1572 {
          tunnel: [w1593 "HW Error"] -> w1581
          frame No Error {
            # "If cycle run,\nwait again"
            n1018 = property on="SequenceHistory" class="Tbl (strict)"() -> ("Value"=w1592:string[][])  [unwired: 2 in, 2 out]
            n1019 = Index Array(array=w1592, index (row)=0, index (col)=1 ("disabled index (col)")) -> (element=w1591:string)
            n1020 = property on="Cycle" class="Bool (strict)"() -> ("Value"=w1589:bool)  [unwired: 2 in, 2 out]
            n1021 = Equal?(x="-1", y=w1591) -> (x = y?=w1588:bool)
            n1022 = And(x=w1589, y=w1588) -> (x .and. y?=w1585:bool)
            n1023 = case shown="False" w1585 {
              tunnel: ["Complete" "Waiting"] -> w1593
              frame False {
              }
              frame True {
              }
            }
          }
          frame Error {
            # "don't want \"complete\" if error!"
          }
        }
        n1024 = invoke on="SequenceHistory" class="Tbl (strict)" method="Set Cell Value"("X Index"=2 ("disabled index (col)"), "Y Index"=w1564, "Value"=w1581) -> (error out=w1578:errorcluster)  [unwired: 3 in, 5 out]
        n1025 = case shown="No Error" w1572 {
          selector: w1572 -> [w1597 w1605]
          tunnel: w1578 -> [_ _]
          frame No Error {
            n1026 = local write "Run/Sequence Error"(w1597) -> ()
            n1027 = local read "Seq. Event"() -> (w1600:refnum<user-event>)
            n1028 = Bundle("milliseconds to wait"=u32 0, FALSE) -> (w1601:cluster{"milliseconds to wait":u32, bool})  [unwired: 1 in]
            n1029 = Generate User Event(user event=w1600, event data cluster=w1601, error in=w1597) -> ()  [unwired: 1 in, 2 out]
          }
          frame Error {
            w1603 = T12."Enabled" ("Disabled")
            w1602 = FALSE
            n1030 = property on="Run/Sequence Error" class="Clust (strict)"("Val(Sgnl)"=w1605) -> ()  [unwired: 2 in, 2 out]
            n1031 = property on="Run Button" class="Bool (strict)"("Value"=w1602, "DisabledEnum"=w1603) -> ()  [unwired: 2 in, 2 out]
            n1032 = property on="Run Seq Button" class="Bool (strict)"("Value"=w1602, "DisabledEnum"=w1603) -> ()  [unwired: 2 in, 2 out]
            n1033 = property on="RandomSequence" class="Bool (strict)"("DisabledEnum"=w1603) -> ()  [unwired: 2 in, 2 out]
            n1034 = property on="StopExperiment" class="Bool (strict)"("Value"=w1602, "DisabledEnum"=T12."Disabled and Grayed Out" ("Disabled")) -> ()  [unwired: 2 in, 2 out]
          }
        }
      }
      event "quit": Value Change {
        n1035 = event-data() -> ("NewVal"=w1606:bool)  [unwired: 1 in, 1 out]
      }
    }
  }
  n1036 = Obtain Queue(name (unnamed)="FBVarSeqSetJSON", element data type=T9 [] ("JSONVarSet")) -> (queue out=w1:refnum<queue>, error out=w43:errorcluster)  [unwired: 3 in, 1 out]
  "FBVarSeqSetJSON queue" <- w1
  n1037 = call "TCPListenJSON.vi"("error in (no error)"=w44) -> ("error out"=w50:errorcluster, "listener ID"=w51:refnum<k5>)  [unwired: 9 in]
  n1038 = while {
    shift-right: [w1612] -> w52
    shift-left: w54 -> [w1616]
    tunnel: w21 -> [w1609]
    tunnel: [w1610] -> w53
    shift-right: [w1607] -> _
    shift-left: w44 -> [w1607]
    stop <- w1608 stop-if-true
    # "Check every 1s if we need to stop"
    # "Manage Variables Requests"
    n1039 = local read "TCP Quit Signal"() -> (w1608:bool)
    n1040 = Dequeue Element(queue=w1616, timeout in ms (-1)=1000, error in (no error)=w1607) -> (queue out=w1612:refnum<queue>, element=w1614:T9, timed out?=w1613:bool, error out=w1611:errorcluster)
    n1041 = case shown="False" w1613 {
      tunnel: [w1617 w1621] -> w1610
      tunnel: w1614 -> [w1619 _]
      tunnel: w1611 -> [w1618 w1621]
      tunnel: w1609 -> [w1620 _]
      frame False {
        n1042 = call "LoadJSONVarSetIntoVM.vi"("error in (no error)"=w1618, "JSONVarSet"=w1619, "VariableManagerRef in"=w1620) -> ("error out"=w1617:errorcluster)  [unwired: 7 in, 1 out]
      }
      frame True {
      }
    }
  }
  n1043 = while {
    shift-right: [w1629] -> w58
    shift-left: w61 -> [w1633]
    tunnel: w60 -> [w1627]
    tunnel: [w1624] -> w59
    shift-right: [w1622] -> _
    shift-left: w57 -> [w1622]
    stop <- w1625 stop-if-true
    # "Check every 1s if we need to stop"
    # "Manage Mulligan Requests"
    n1044 = Dequeue Element(queue=w1633, timeout in ms (-1)=1000, error in (no error)=w1622) -> (queue out=w1629:refnum<queue>, element=w1631:string, timed out?=w1630:bool, error out=w1628:errorcluster)
    n1045 = case shown="False" w1630 {
      tunnel: [w1637 w1638] -> w1624
      tunnel: w1631 -> [w1636 _]
      tunnel: w1628 -> [w1635 w1638]
      tunnel: w1627 -> [w1634 _]
      frame False {
        n1046 = call "MulliganFilenumber.vi"("error in (no error)"=w1635, "FileNumber"=w1636, "SequenceHistory ref"=w1634) -> ("error out"=w1637:errorcluster)  [unwired: 2 in, 2 out]
      }
      frame True {
      }
    }
    n1047 = local read "TCP Quit Signal"() -> (w1626:bool)
    n1048 = Unbundle By Name(w1624) -> ("status"=w1623:bool)
    n1049 = Or(x=w1623, y=w1626) -> (x .or. y?=w1625:bool)
  }
  n1050 = while {
    tunnel: w43 -> [_]
    shift-right: [w1640] -> w47
    shift-left: w51 -> [w1641]
    shift-right: [w1639] -> _
    shift-left: w50 -> [w1639]
    stop <- w1642 stop-if-true
    # "Watch for Variables Requests over TCP"
    n1051 = local read "TCP Quit Signal"() -> (w1642:bool)
    n1052 = TCP Wait On Listener(8:w1639, 9:1000 ("timeout in ms (-1)"), 11:w1641) -> (0:w1645:errorcluster, 3:w1640:refnum<k5>, 4:w1644:refnum<k5>)  [unwired: 1 in, 2 out]
    n1053 = case shown="No Error" w1645 {
      selector: w1645 -> [w1647 w1648]
      tunnel: w1644 -> [w1646 _]
      frame No Error {
        n1054 = call "TCPGetProcessJSON.vi"("error in (no error)"=w1647, "connection ID"=w1646) -> ()  [unwired: 10 in]
      }
      frame Error {
        w1650 = T26 2 items=["no dialog", "OK message", "continue or stop message", "OK message + warnings", "continue/stop + warnings"] ("type of dialog (OK msg:1)")
        w1651 = 1 items=["no exception", "cancel error on match", "set error on match"] ("[exception action] (none:0)")
        # "Timed Out"
        n1055 = call "ClearTCPTimeout.vi"("error in (no error)"=w1648) -> ("error out"=w1649:errorcluster)  [unwired: 9 in, 1 out]
        n1056 = call <vilib>:"General Error Handler.vi"("type of dialog (OK msg:1)"=w1650, "error in (no error)"=w1649, "[exception action] (none:0)"=w1651, "[exception code]"=-1967390702 ("y")) -> ()  [unwired: 7 in, 5 out]
      }
    }
  }
  n1057 = Release Queue(queue=w52, error in (no error)=w53) -> (error out=w45:errorcluster)  [unwired: 1 in, 2 out]
  n1058 = Release Queue(queue=w1, error in (no error)=w45) -> ()  [unwired: 1 in, 3 out]
  n1059 = TCP Close Connection(connection ID=w47) -> ()  [unwired: 2 in, 2 out]
  n1060 = Release Queue(queue=w58, error in (no error)=w59) -> ()  [unwired: 1 in, 3 out]
